vi "Real-Time v01.vi"() -> ()   [LabVIEW 2014]
uses:
  <vilib>/rvi/interface/nirviOpenFPGA/nirviOpenFPGA.xnode
  <vilib>/rvi/interface/nirviReadWriteControl/nirviReadWriteControl.xnode
  <vilib>/Platform/TimedLoop/XDataNode/XDataNode.xnode
  <vilib>/Platform/TimedLoop/XDataNode/nitl_modes.ctl
  <vilib>/Platform/TimedLoop/XDataNode/XDNodeRunTimeDep.lvlib
  <vilib>/Platform/TimedLoop/XDataNode/wakeup.ctl
  <vilib>/Platform/TimedLoop/XDataNode/timing_clust.ctl
  <vilib>/addons/control/pid/NI_PID_pid.lvlib
  <vilib>/rvi/errors/niLvFpgaAdjustHostInterfaceError.vi
  <vilib>/rvi/interface/nirviCloseFPGA/nirviCloseFPGA.xnode
  <vilib>/addons/control/pid/pid.llb/PID (DBL).vi
  NiFpgaLv.dll
  <vilib>/Utility/error.llb/Error Cluster From Error Code.vi
  FPGA Bitfiles/OMEGA_FPGATarget2_FPGASlavev02_Fgk3BcBTm4Y.lvbitx
  FPGA Bitfiles/OMEGA_FPGATarget_FPGAMainv01_bQBX2IVMCsY.lvbitx
  <vilib>/FPGAPlugInAG/cRIO-9067/niLvFpga_Open_cRIO-9067.vi
  <vilib>/FPGAPlugInAG/NI 9146/niLvFpga_Open_NI 9146.vi
  <vilib>/FPGAPlugInAG/cRIO-9067/niLvFpga_Close_cRIO-9067.vi
panel:
  in  "Tc":i32=1
  out "Selectable Tc Tref":dbl format="%#_13g"
  out "Selectable Tc MA":dbl format="%#_13g"
  in  "Red Limit":dbl
  in  "T ref":bool
  in  "Tc Alarm":bool
  in  "Target Temperature":dbl format="%0.2f"
  in  "Yellow Limit":dbl
  out "Fan Factor Speed":dbl
  in  "Fan Speed Recipe":bool
  out "Tstoic 2 R":bool
  out "Tstoic 2 Y":bool
  out "Tstoic 1 R":bool
  out "Tstoic 1 Y":bool
  out "Tspike 2 R":bool
  out "Tspike 2 Y":bool
  out "Omicron 2":bool
  out "Tspike 1 R":bool
  out "Tspike 1 Y":bool
  out "Tref 2 R":bool
  out "Tref 2 Y":bool
  out "Tref 1 R":bool
  out "Tref 1 Y":bool
  out "AutoChanges Spike":string[][](table)
  out "UserChanges Spike":string[][](table)
  out "HC Add":dbl
  out "Exceeded 2":bool
  in  "Write Log":bool
  out "AutoChanges":string[][](table)
  out "UserChanges":string[][](table)
  out "Furnace SP":dbl
  out "Exceeded":bool
  in  "Spike Control":bool
  in  "Target Tspike":dbl
  in  "Target Tstoic":dbl
  in  "Control TC 2":i32=2
  out "T Spike 2":dbl format="%0.2f"
  out "T Max 2":dbl format="%0.2f"
  out "T Stoic 2":dbl
  out "T Ref 2":dbl
  in  "HC 2 Factor":dbl
  in  "HC 2 Add Factor":dbl
  in  "Air-2 Factor":dbl
  in  "Air-2 Add Factor":dbl
  in  "O2-2 Factor":dbl
  in  "Power Limit":dbl
  out "Omicron":bool
  out "T Spike":dbl format="%0.2f"
  in  "TSpike":bool
  in  "TSpike Target":dbl format="%0.2f"
  in  "TStoic":bool
  in  "TStoic Target":dbl format="%0.2f"
  out "Alarm Output 2":bool[](array[boolean])
  in  "Flow":bool
  in  "Lambda":bool
  in  "Pressure":bool
  in  "Heat Exch Fan V":fxp<+/-,20,5>
  in  "Air Bal Transient":dbl
  in  "Air Bal Adaptive Control":bool
  in  "HC Bal Adaptive Control":bool
  in  "HC Bal Transient":dbl
  in  "TRef":bool
  in  "TRef Target":dbl format="%0.2f"
  out "T Max":dbl format="%0.2f"
  out "T Stoic":dbl
  out "T Ref":dbl
  in  "Extract Fan V":fxp<+/-,20,5>
  in  "ETAS Control":bool
  in  "Dual Evac":bool
  out "Valve 4":dbl
  out "Valve 3":dbl
  out "OSCArray":dbl[](array[numeric])
  out "Flow rate g/s":dbl
  out "OSC Stop":bool
  in  "O2 Factor":dbl
  in  "HC Switch":bool
  out "Time Step":i32
  out "O2":bool
  out "HC-2":bool
  out "N2-2":bool
  in  "Valve 3 SP":dbl=1.0
  in  "Valve 4 SP":dbl=1.0
  in  "N2 Age":dbl
  in  "N2 2":dbl format="%#_13g"
  in  "N2":dbl format="%#_13g"
  in  "O2":dbl format="%#_13g"
  out "Flow Avg":dbl
  in  "Flow Up":sgl=50.0
  in  "Flow Low":sgl
  out "Avg Control":dbl format="%0.2f"
  out "Uego Avg Fur":dbl
  in  "PID gains O2":T1={"proportional gain (Kc)"=1.0, "integral time (Ti, min)"=0.01, "derivative time (Td, min)"=0.0} {"derivative time (Td, min)" format="%.3f"; "integral time (Ti, min)" format="%.3f"; "proportional gain (Kc)" format="%.3f"}
  in  "PID gains CO":T1={"proportional gain (Kc)"=1.0, "integral time (Ti, min)"=0.01, "derivative time (Td, min)"=0.0} {"derivative time (Td, min)" format="%.3f"; "integral time (Ti, min)" format="%.3f"; "proportional gain (Kc)" format="%.3f"}
  in  "Manual Valve":bool
  in  "Control TC":i32=1
  in  "Flow Offset":dbl
  in  "HC Fact HCLO":dbl
  in  "HC Base HCLO":dbl
  in  "O2 Base HCLO":dbl
  in  "O2 Fact HCLO":dbl
  in  "Ageing Metric\nControl":enum32{"Catalyst 1 ", "Catalyst 2 ", "All"}(radio)
  out "UEGO Array":dbl[](array[numeric])
  in  "UEGO 3":i64=200
  out "UEGO Sensor Results":T2
  in  "SensorControl":T3={"UEGO1Enable"=TRUE, "UEGO2Enable"=TRUE, "EGO1Enable"=FALSE, "EGO2Enable"=FALSE, "EGO3Enable"=FALSE, "EGO4Enable"=FALSE, "UEGO1Range"=FALSE, "UEGO2Range"=FALSE, "FilterCutoff (Hz)"=10.0}
  in  "UEGO Back Pressure (bar)":T4={"UEGO1BackPressure (bar)"=1.013, "UEGO2BackPressure (bar)"=1.013}
  in  "UEGOModuleEnable":bool=TRUE
  out "UEGO Heater (V)":T5
  out "UEGO Diagnostics":T6={"ModulePresent"=FALSE, "UEGO1SensorFault"=63, "UEGO2SensorFault"=63, "UEGO1HeaterFault"=192, "UEGO2HeaterFault"=192, "UEGOFuseStatus"=0, "Battery (V)"=0.0, "LSUType"=0} {"LSUType" items=["LSU 4.9", "LSU 4.2"]; "UEGOFuseStatus" items=["FUSE OK", "FUSE BLOWN"]; "UEGO2SensorFault" items=["NO FAULT"=63, "SHORT TO GND OR BATT"=0]; "UEGO2HeaterFault" items=["SHORT TO GROUND"=0, "OPEN CIRCUIT"=64, "SHORT TO BATTERY"=128, "NO FAULT"=192]; "UEGO1SensorFault" items=["NO FAULT"=63, "SHORT TO GND OR BATT"=0]; "UEGO1HeaterFault" items=["SHORT TO GROUND"=0, "OPEN CIRCUIT"=64, "SHORT TO BATTERY"=128, "NO FAULT"=192]}
  out "UEGO Temperature (C)":T7
  in  "Start Test":bool
  out "Ready":bool
  in  "Reset AM 2":bool
  out "% Complete 2":dbl
  out "Complete 2":dbl(slide) scale=0.0..100.0
  out "Remaining Time 2":dbl format="%<%H:%M:%S>t"
  out "Ageing Time 2":dbl format="%<%H:%M:%S>t"
  in  "P-Transducer 1":enum32{"Druck ", "FUJI ", "Impress"}(radio)=enum."FUJI "
  out "Valve 2":dbl
  out "Valve 1":dbl
  in  "Valve 2 SP":dbl=1.0
  in  "Valve 1 SP":dbl=1.0
  out "Lambda Avg":dbl
  in  "Press Up":sgl=5.0
  in  "Press Low":sgl
  out "Loop No.":i32
  out "Air-2":bool
  out "HC-B":bool
  out "Air-B":bool
  out "N2":bool
  out "NO":bool
  out "Air":bool
  out "HC":bool
  out "CO":bool
  in  "NO/CO-2 Factor":dbl
  in  "CO Factor":dbl
  in  "Set-point Fan":dbl
  in  "Fan PID":bool
  in  "Furnace SP":dbl=2.0
  in  "Furnace Manual":bool
  in  "Reset AM 1":bool
  in  "Lambda Control":bool
  in  "Lambda SP 3":dbl
  in  "Output Low 3":dbl
  in  "Output High 3":dbl
  in  "PID Mop-up Catalyst":T1={"proportional gain (Kc)"=0.8, "integral time (Ti, min)"=0.8, "derivative time (Td, min)"=0.0}
  in  "NO PID Light-Off":T1={"proportional gain (Kc)"=1.0, "integral time (Ti, min)"=0.0, "derivative time (Td, min)"=0.0}
  in  "NO PID Sweep Test":T1={"proportional gain (Kc)"=1.0, "integral time (Ti, min)"=0.0, "derivative time (Td, min)"=0.0}
  in  "NO":dbl format="%#_13g"
  in  "CO":dbl format="%#_13g"
  out "% Complete":dbl
  out "Complete":dbl(slide) scale=0.0..100.0
  out "Remaining Time":dbl format="%<%H:%M:%S>t"
  out "Ageing Time":dbl format="%<%H:%M:%S>t"
  out "Tank Pressure":dbl
  out "Inlet Temp":sgl
  out "Cycle Length":i32
  in  "HC Cyc 2":dbl format="%#_13g"
  in  "HC Bal":dbl format="%#_13g"
  in  "Air Cyc 1":dbl format="%#_13g"
  in  "Air Cyc 2":dbl format="%#_13g"
  in  "Air Bal":dbl format="%#_13g"
  in  "HC Cyc 1":dbl format="%#_13g"
  in  "Furnace 1":sgl=10.0
  in  "Air Cyc Add Factor":dbl
  in  "Air Cyc Factor":dbl
  in  "HC Cyc Add Factor":dbl
  in  "HC Bal Factor":dbl
  in  "Air Bal Factor":dbl
  in  "HC Cyc Factor":dbl
  in  "Stoic Control":bool
  in  "Lambda \nTarget":sgl=5.0
  out "Flow 1":dbl
  out "Test Start":i32
  out "Control Variables":dbl[](array[numeric])
  out "Iteration \nDuration 3":i64
  in  "NO Base NOLO":dbl
  in  "NO Factor NOLO":dbl
  in  "CO Base NOLO":dbl
  in  "CO Factor NOLO":dbl
  in  "CO Base COLO":dbl
  in  "O2 Base COLO":dbl
  in  "CO Fact COLO":dbl
  in  "O2 Fact COLO":dbl
  in  "NO Furnace Inlet":dbl=5.0
  in  "CO Furnace Inlet":dbl=5.0
  in  "OSC Furnace Inlet":dbl=5.0
  in  "HC Furnace Inlet":dbl=0.2
  in  "Sw time":dbl
  in  "Age Furnace Inlet":dbl=5.0
  in  "Age Lam Lim":dbl=5.0
  in  "OSC Lam lim":dbl=5.0
  in  "CO Lam Lim":dbl=5.0
  in  "NO Lam Lim":dbl=5.0
  in  "Fan Speed V":dbl
  in  "HC Lam lim":dbl=0.2
  in  "STOP":bool
  in  "TankLo":dbl=1.5
  in  "TankHi":dbl=2.0
  out "DI no1":u32
  in  "PID Inverter":T1={"proportional gain (Kc)"=0.8, "integral time (Ti, min)"=0.8, "derivative time (Td, min)"=0.0}
  out "Iteration Duration 2":i64
  # "Spike Change Log"
  # "Furnace Change Log"
  # "OMEGA Real-Time"
  # "Loop Readings"
  # "MFC Alarms"
  # "System Readings"
  # "Pressure Release Limits"
  # "Ageing Metric 1"
  # "kPa"
  # "kPa"
  # "Fan Control"
  # "Cooling Fan Control"
  # "Warm-up"
  # "Rapidox Limit"
  # "Furnace Limit"
  # "Ageing Metric 2"
  # "g/s"
  # "Furnace Control"
  # "Ageing"
  # "Cycle Alarms"
  # "System Settings"
  # "Cycle Factors"
  # "System Balance Factors"
  # "Mopup Lambda PID Control"
  # "When Adaptive Control \nSelected Air Bal Factor \nwill adjust lambda up or\n down it will not affect \nTransients"
  # "When Adaptive Control \nSelected HC Bal Factor \nwill adjust lambda up or\n down it will not affect \nTransients"
  # "On ETAS\nOff Furnace"
  # "Furnace PID Control"
  # "Other PID Control"
  # "Select for Tref calc,\notherwise MA is used"
  # "Light Off's"
  # "UEGO Module 3"
  # "NO Light - off"
  # "HC Light - off"
  # "CO Light - off"
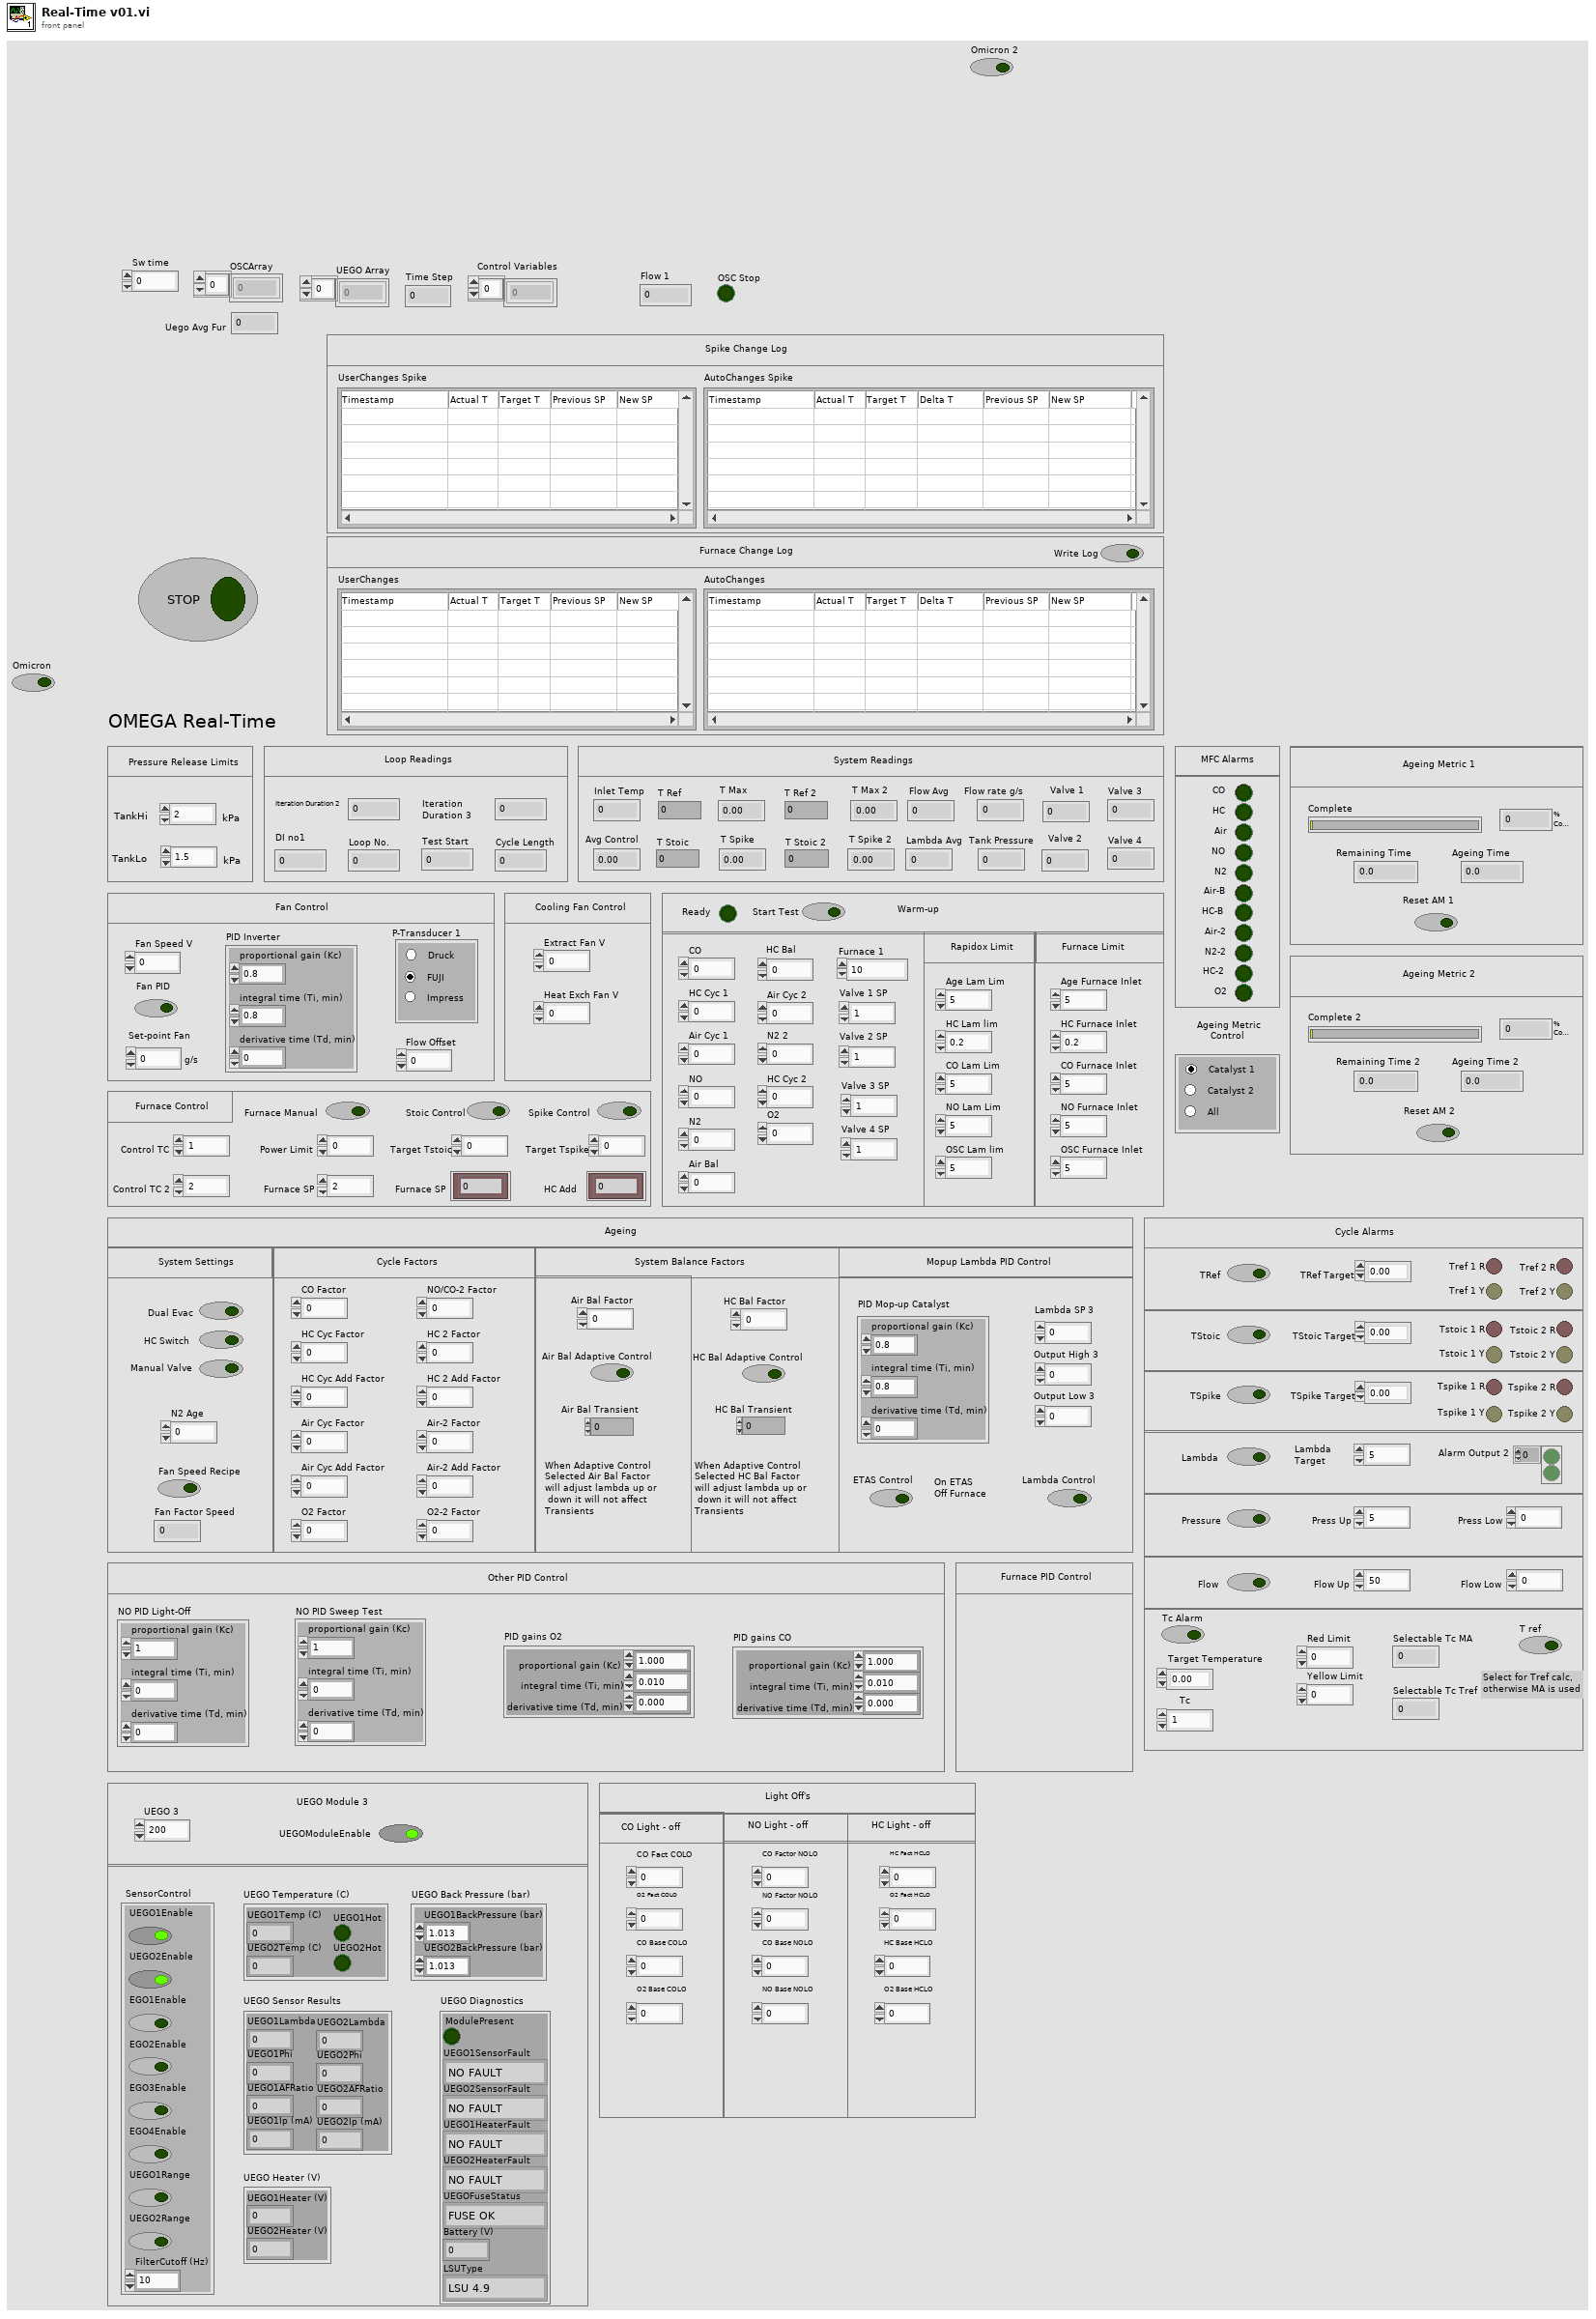
[diagram p1: front panel]
types:
  T1 = cluster{"proportional gain (Kc)":dbl, "integral time (Ti, min)":dbl, "derivative time (Td, min)":dbl}
  T2 = cluster{"UEGO1Lambda":sgl, "UEGO1Phi":sgl, "UEGO1AFRatio":sgl, "UEGO1Ip (mA)":sgl, "UEGO2Lambda":sgl, "UEGO2Phi":sgl, "UEGO2AFRatio":sgl, "UEGO2Ip (mA)":sgl}
  T3 = cluster{"UEGO1Enable":bool, "UEGO2Enable":bool, "EGO1Enable":bool, "EGO2Enable":bool, "EGO3Enable":bool, "EGO4Enable":bool, "UEGO1Range":bool, "UEGO2Range":bool, "FilterCutoff (Hz)":dbl}
  T4 = cluster{"UEGO1BackPressure (bar)":sgl, "UEGO2BackPressure (bar)":sgl}
  T5 = cluster{"UEGO1Heater (V)":sgl, "UEGO2Heater (V)":sgl}
  T6 = cluster{"ModulePresent":bool, "UEGO1SensorFault":u8, "UEGO2SensorFault":u8, "UEGO1HeaterFault":u8, "UEGO2HeaterFault":u8, "UEGOFuseStatus":u8, "Battery (V)":sgl, "LSUType":u8}
  T7 = cluster{"UEGO1Temp (C)":sgl, "UEGO2Temp (C)":sgl, "UEGO1Hot":bool, "UEGO2Hot":bool}
  T8 = cluster{string[][], string[][], dbl[], "Furnace Set-point":dbl, "It Out":i32}
  T9 = typedef "XDNodeRunTimeDep.lvlib/timing_clust.ctl" = cluster{"Expected End [f-1]":u64, "Actual End [f-1]":u64, "Finished Late? [f-1]":bool, "Expected End [i-1]":u64, "Actual End [i-1]":u64, "Finished Late? [i-1]":bool, "Expected Start [i]":u64, "Actual Start [i]":u64, "Expected Start [f]":u64, "Actual Start [f]":u64, "Source Name":string, "Structure Name":string, "Period":i64, "Deadline":i64, "Offset":i64, "Start":i64, "Priority":i32, "Timeout":i32, "Mode":T10, "Wakeup Reason":T11, "Error":errorcluster, "Source Type":string, "Secondary Source Type":string, "Global End Time":u64, "Global Start Time":u64, "Frame Duration":u64, "Iteration Duration":u64, "Assigned CPU":i32, "I/O Scan Engine Mode":u32}
  T10 = typedef "XDNodeRunTimeDep.lvlib/nitl_modes.ctl" = enum32{"No Change", "Process missed periods, maintain original phase", "Discard missed periods, maintain original phase", "Process missed periods, ignore original phase", "Discard missed periods, ignore original phase"}
  T11 = typedef "XDNodeRunTimeDep.lvlib/wakeup.ctl" = enum32{"Normal", "Aborted", "Asynchronous wakeup", "Timing source error", "Timed loop error", "Timeout"}
  T12 = cluster{"UserChanges":string[][], "AutoChanges":string[][], "Stoich Array":dbl[], "Furnace SP":dbl, "It Out":i32}
  T13 = cluster{"UserChanges":string[][], "AutoChanges":string[][], "Spike Array":dbl[], "User HC Add":dbl, "countdown":i32}
  T14 = cluster{"Stoich A/F Ratio":sgl, "IpArray (mA)":sgl[], "LambdaArray":sgl[]}
  T15 = cluster{"UEGO1Diag":u8, "UEGO2Diag":u8, "UEGO1Sensor":u16, "UEGO2Sensor":u16, "UEGO1Heater":u16, "UEGO2Heater":u16, "UEGO1AmpOffset":u16, "UEGO2AmpOffset":u16, "UEGO1RIOffset":u16, "UEGO2RIOffset":u16, "UEGO1HeaterGain":u16, "UEGO2HeaterGain":u16, "Fuse":u16, "EGO1Sensor":u16, "EGO2Sensor":u16, "EGO3Sensor":u16, "EGO4Sensor":u16, "Battery":u16, "ModulePresent":bool, "UEGO1ID":u8, "UEGO2ID":u8, "LSUType":u8}
  T16 = cluster{"ModuleEnable":bool, "WatchdogIn":bool, "UEGO1Hot":bool, "UEGO2Hot":bool, "Cal1Request":bool, "Cal2Request":bool, "UEGOHeaterPeriod":u16, "UEGO1HeaterPulseWidth":u16, "UEGO2HeaterPulseWidth":u16, "UEGO1Range":bool, "UEGO2Range":bool, "LSUType (F=4.9,T=4.2)":bool}
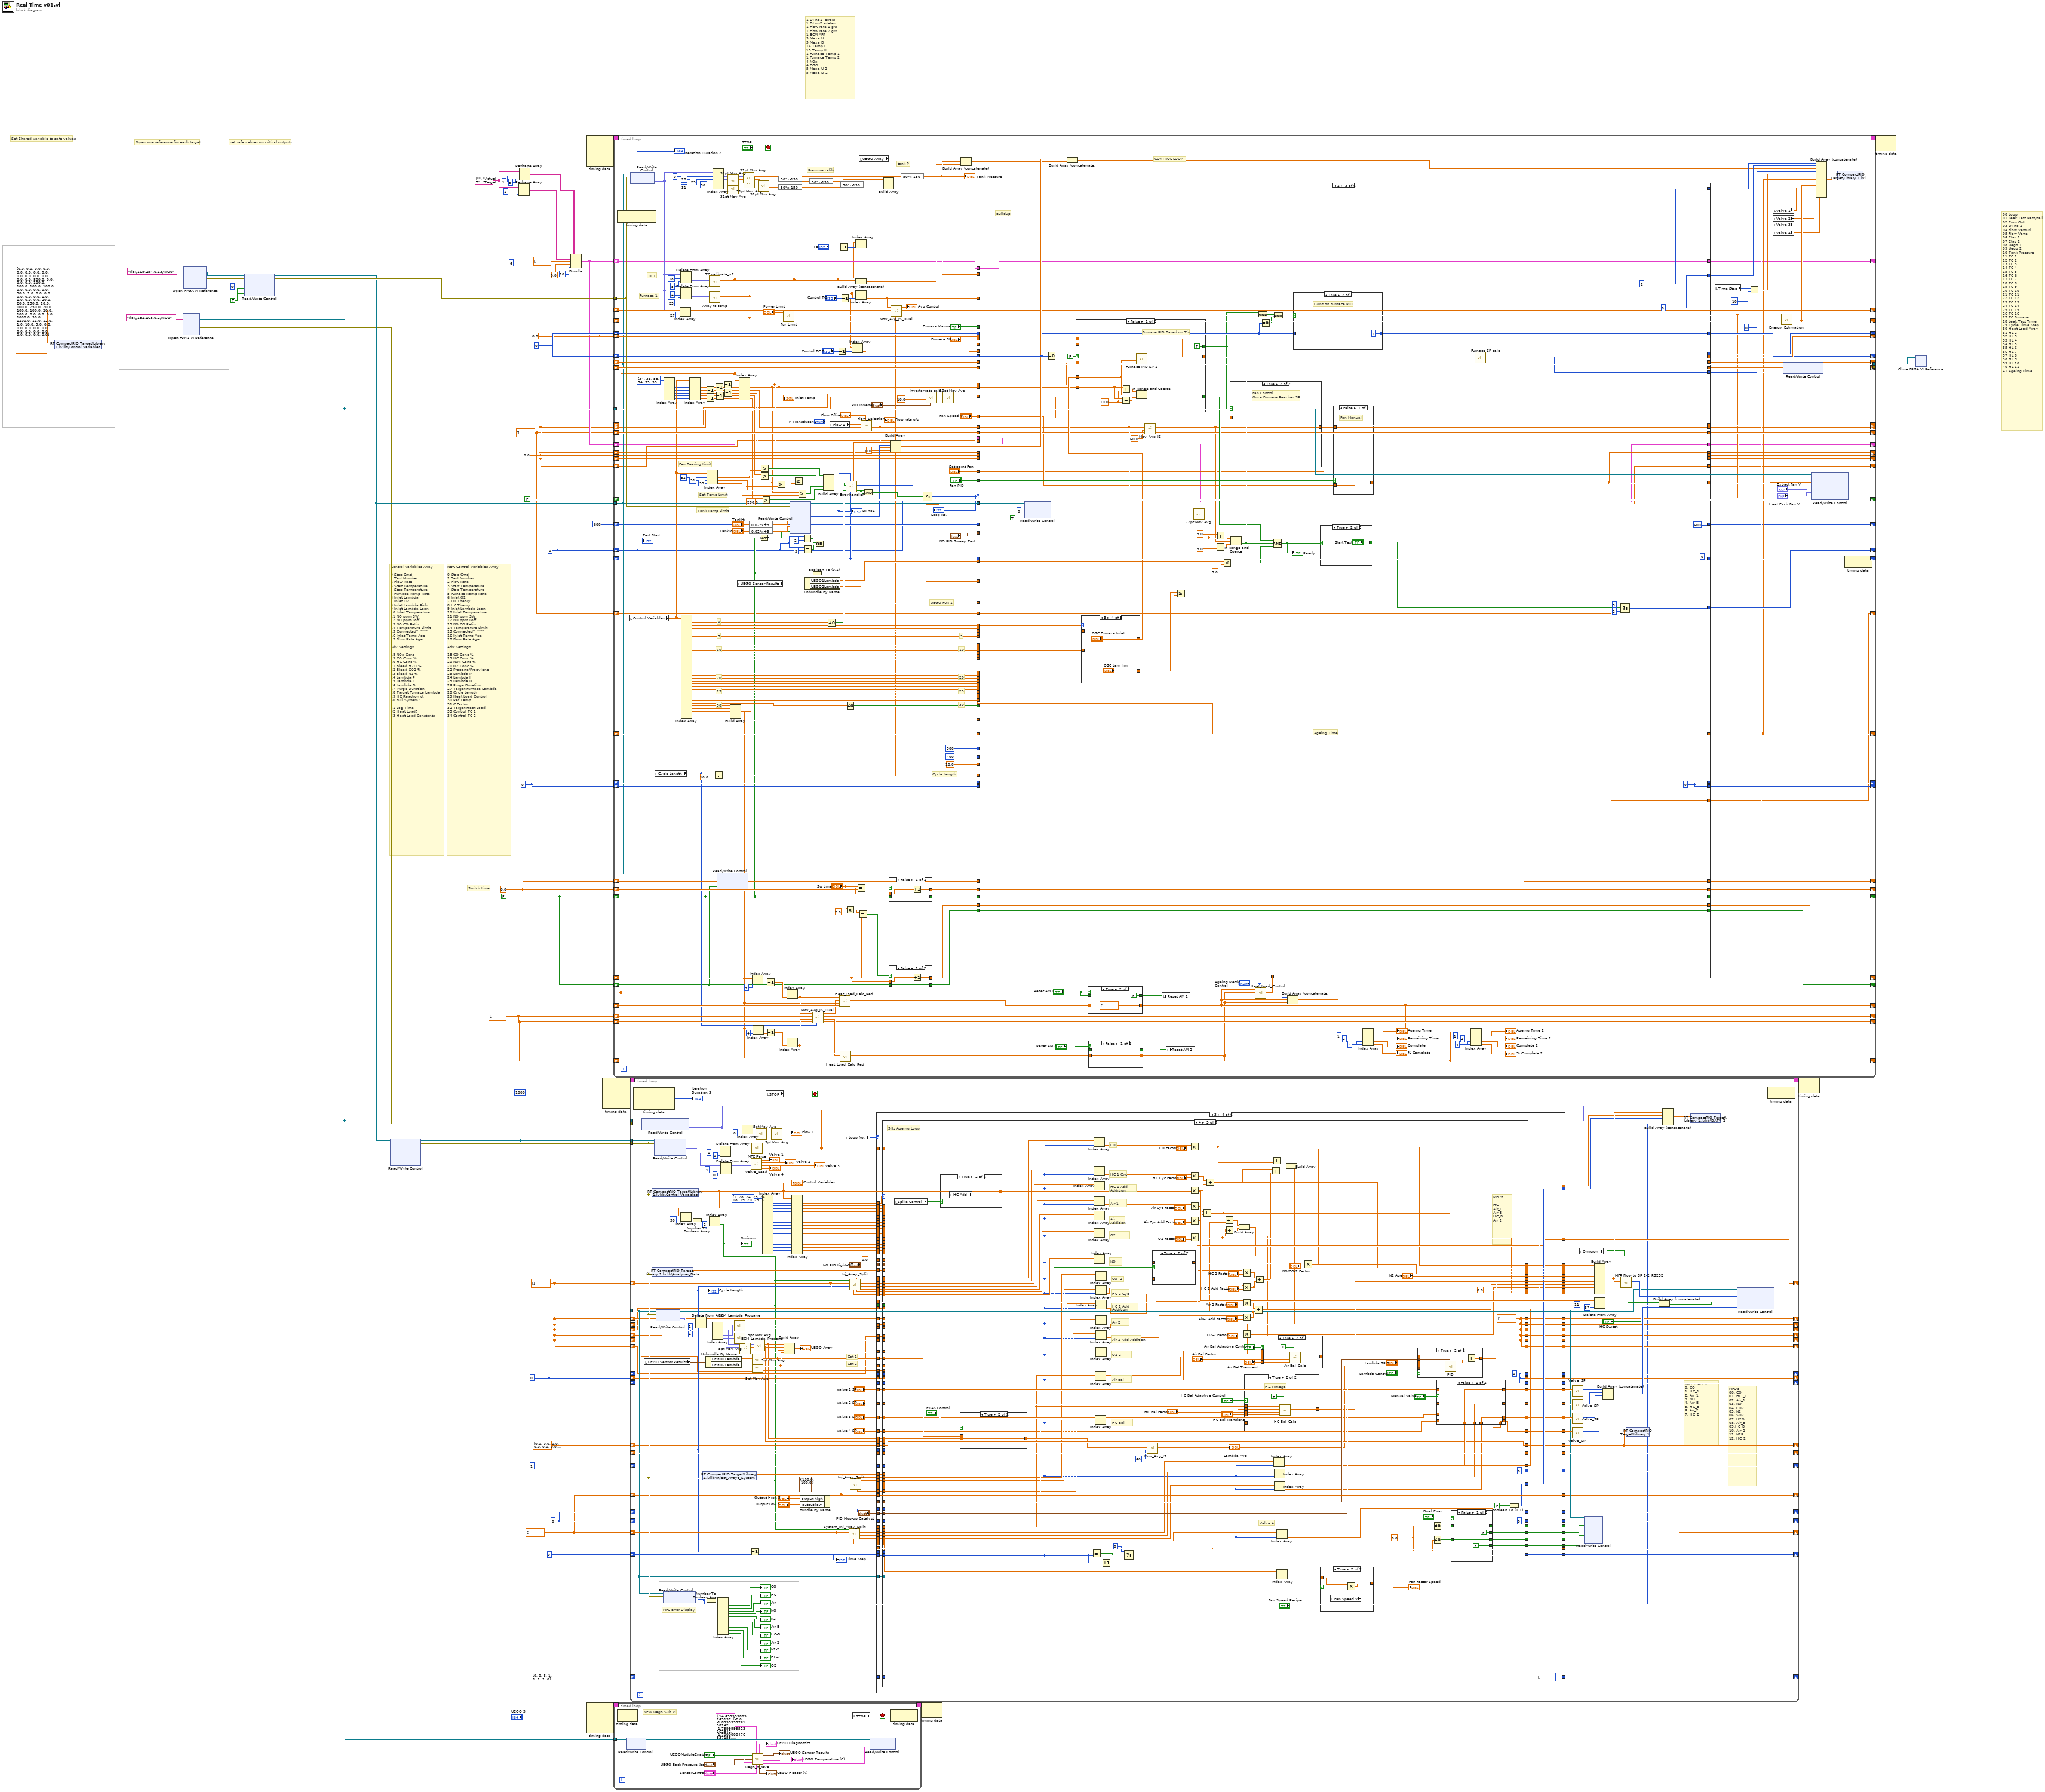
[diagram p0: block diagram]
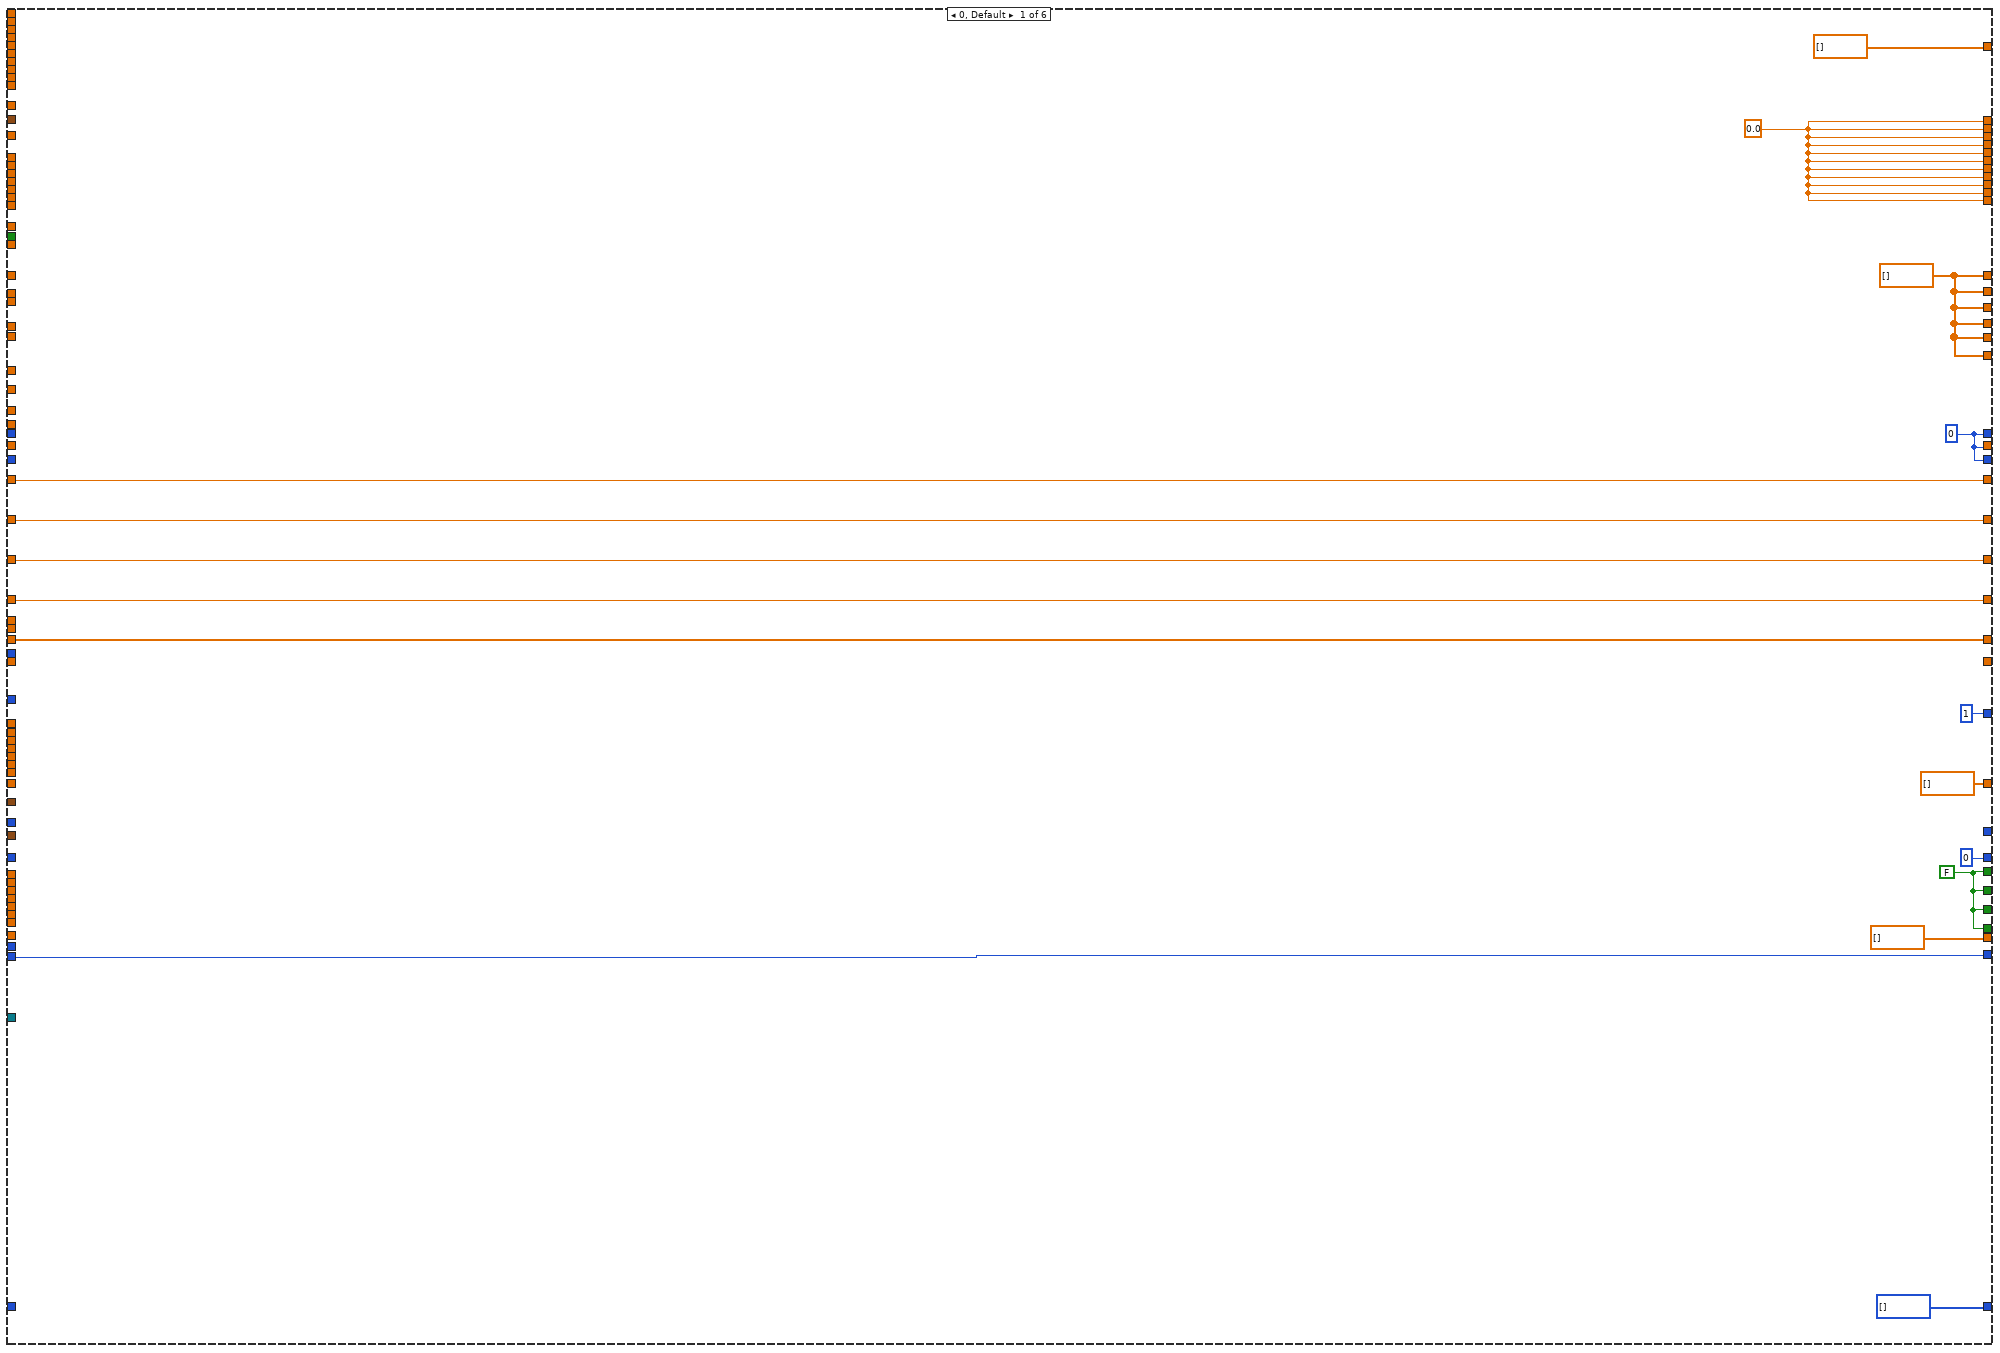
[diagram p2: hidden frame]
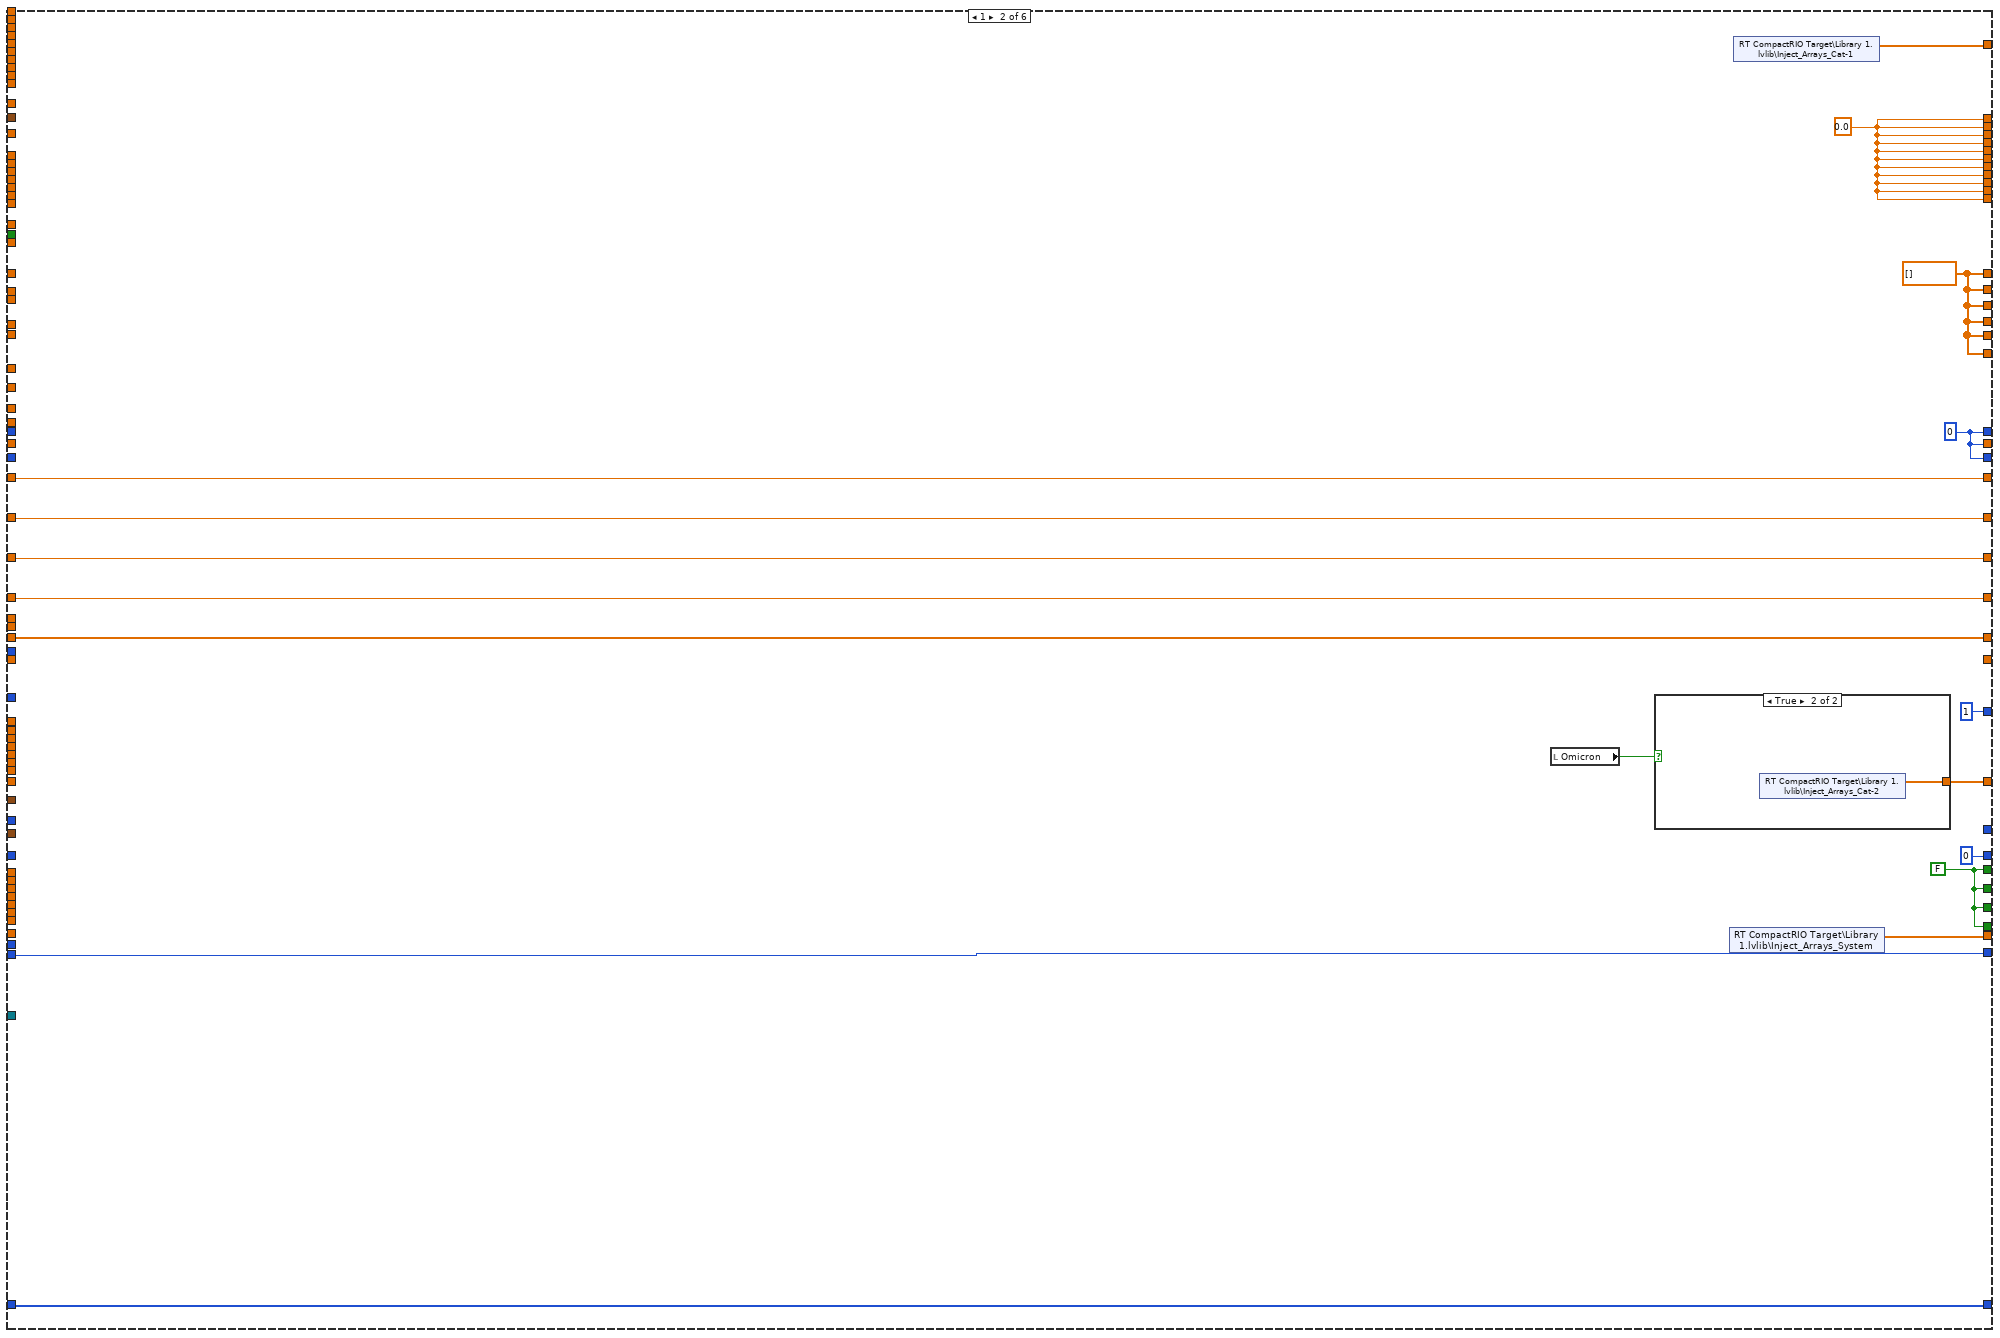
[diagram p3: hidden frame]
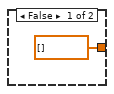
[diagram p4: hidden frame]
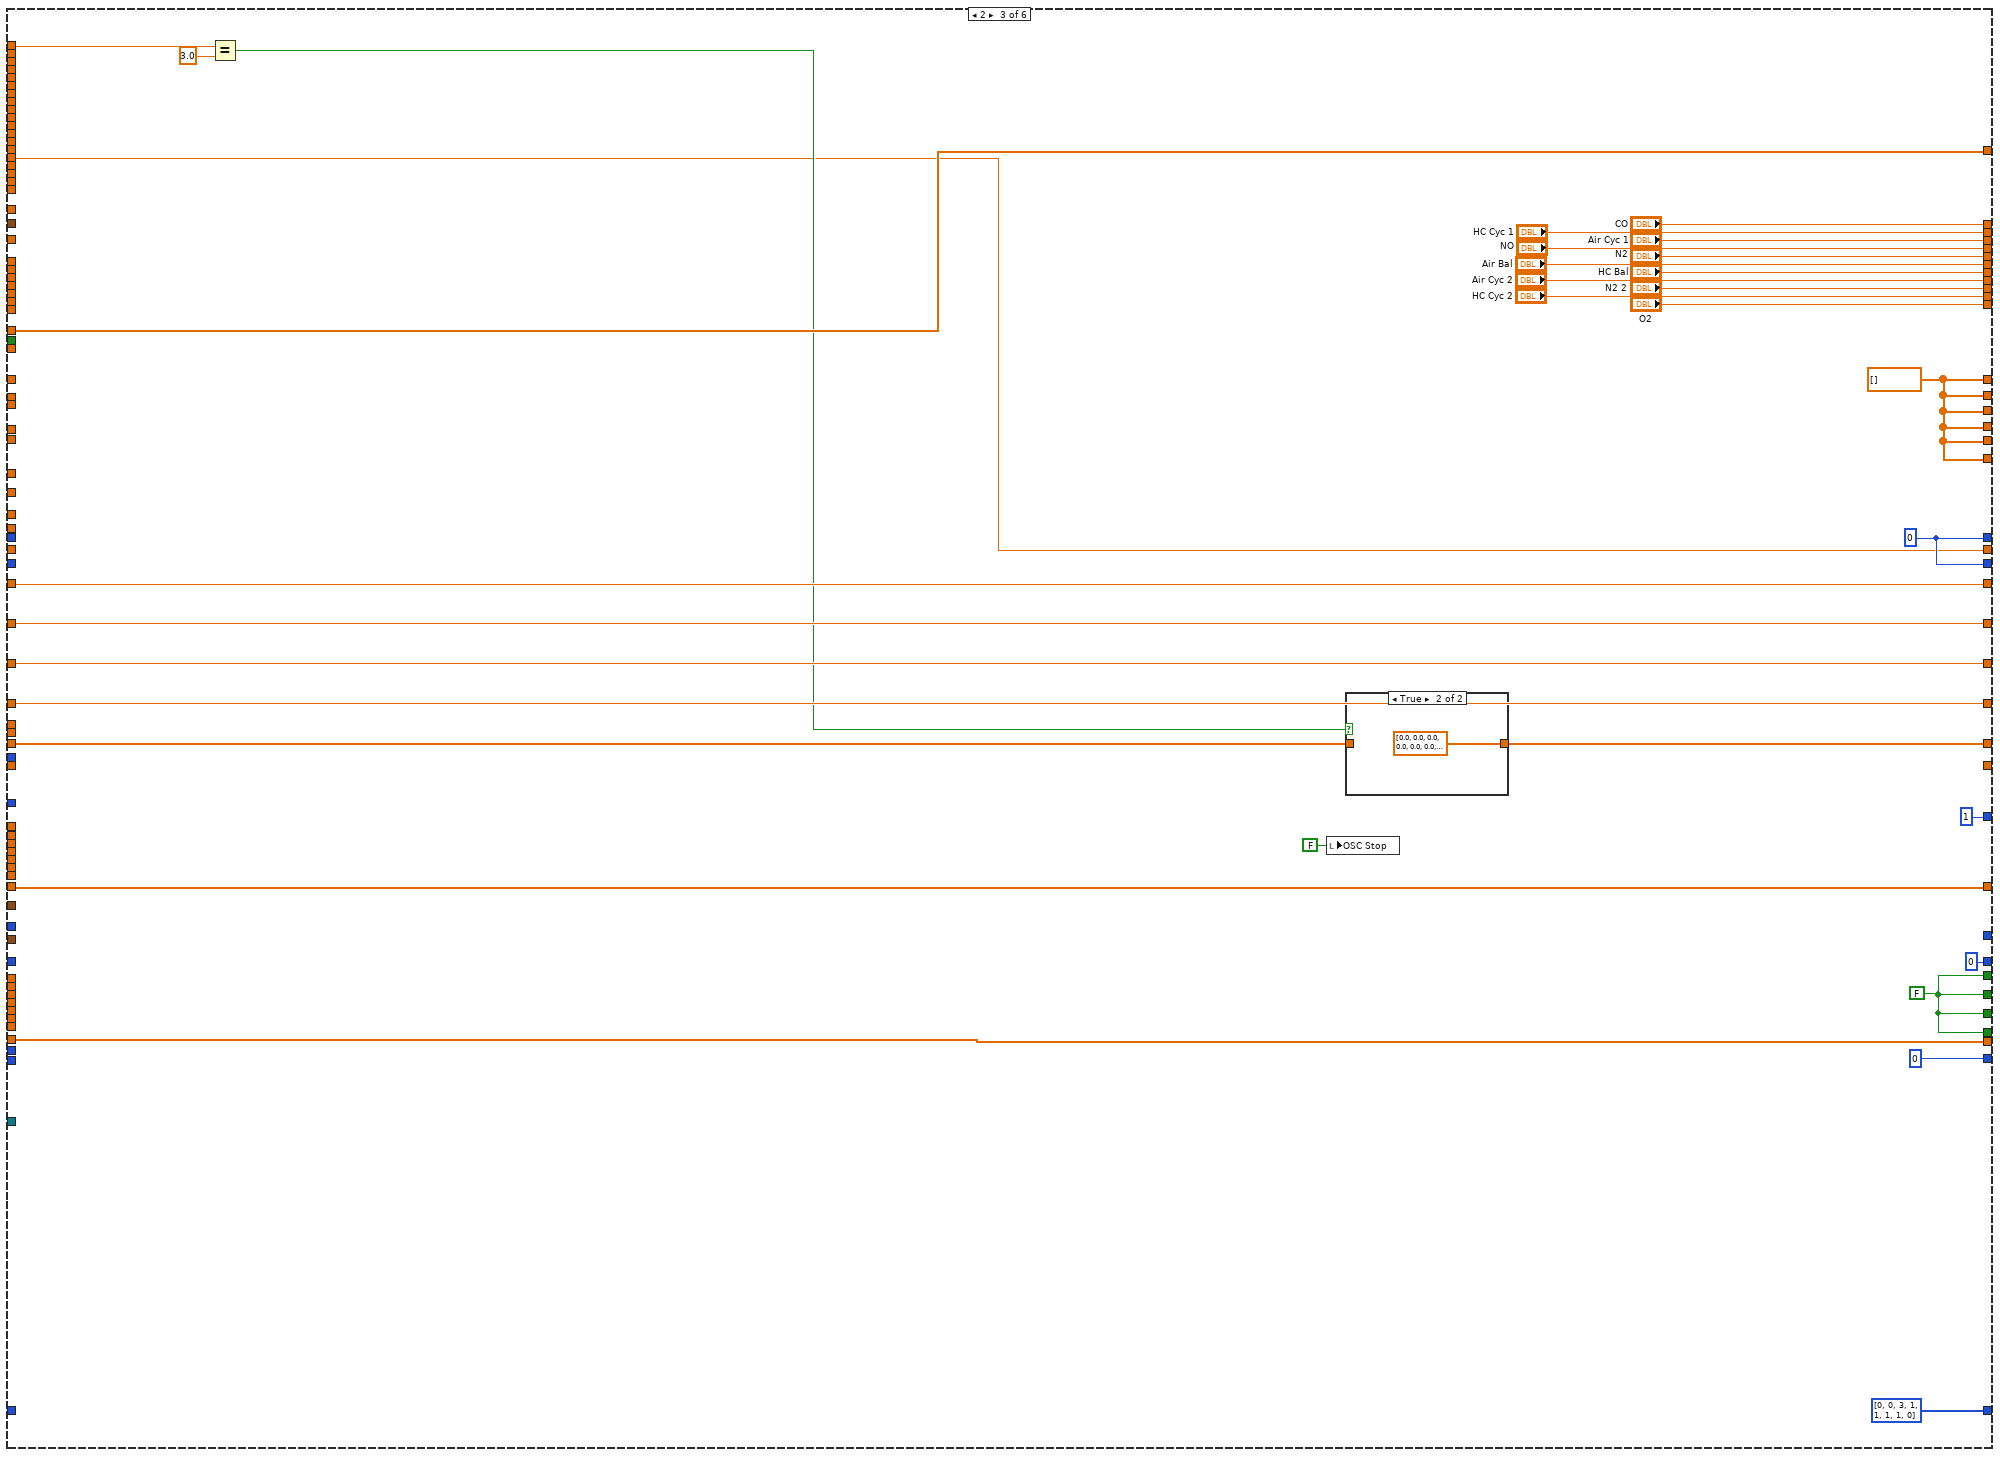
[diagram p5: hidden frame]
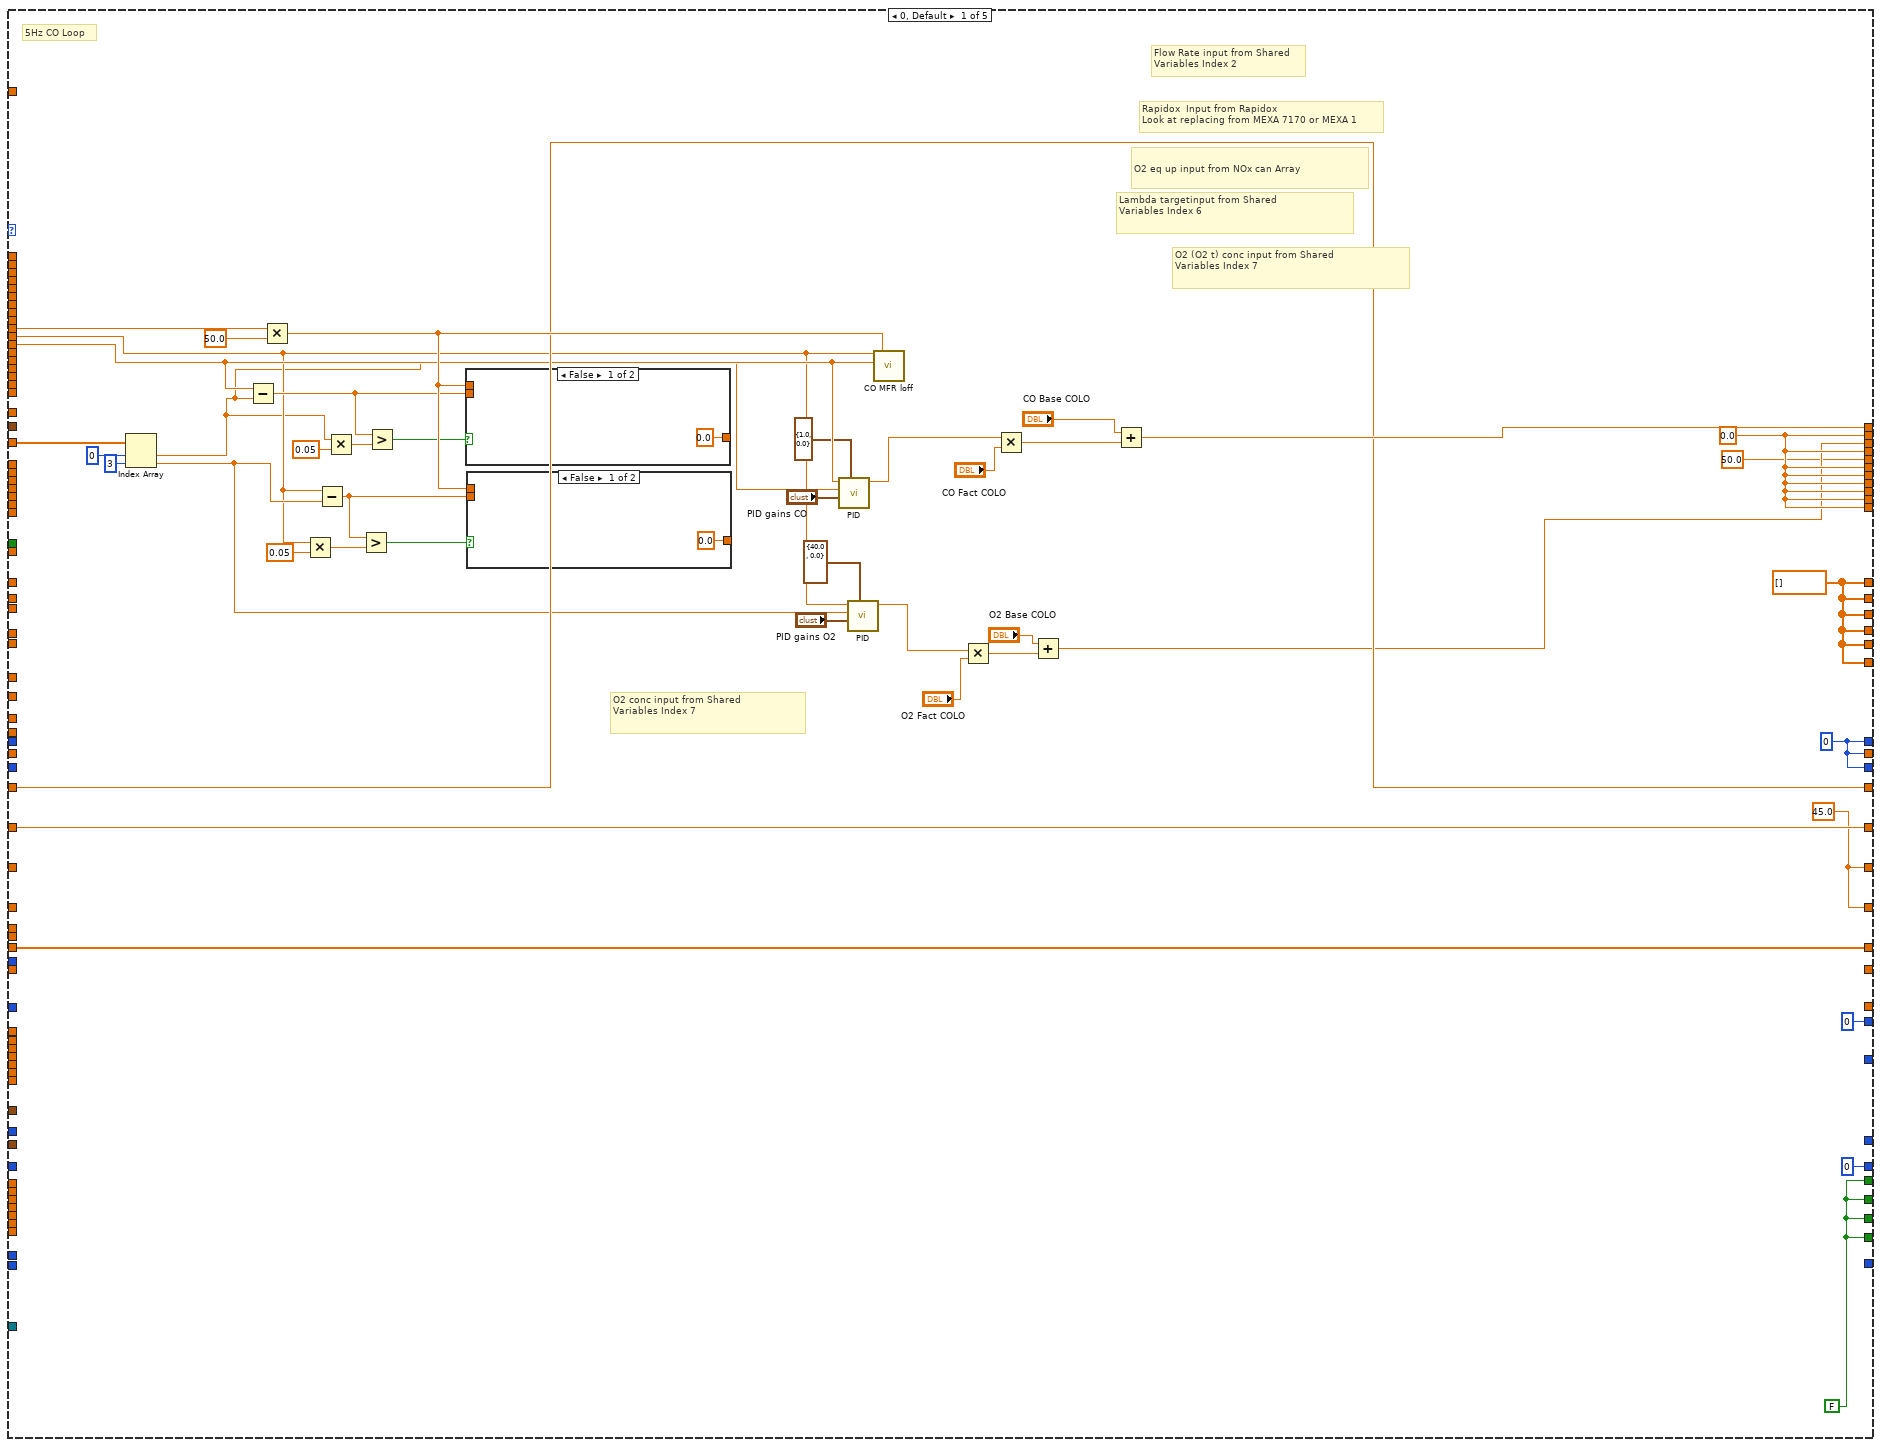
[diagram p7: hidden frame]
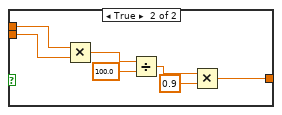
[diagram p8: hidden frame]
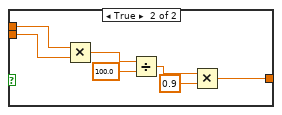
[diagram p9: hidden frame]
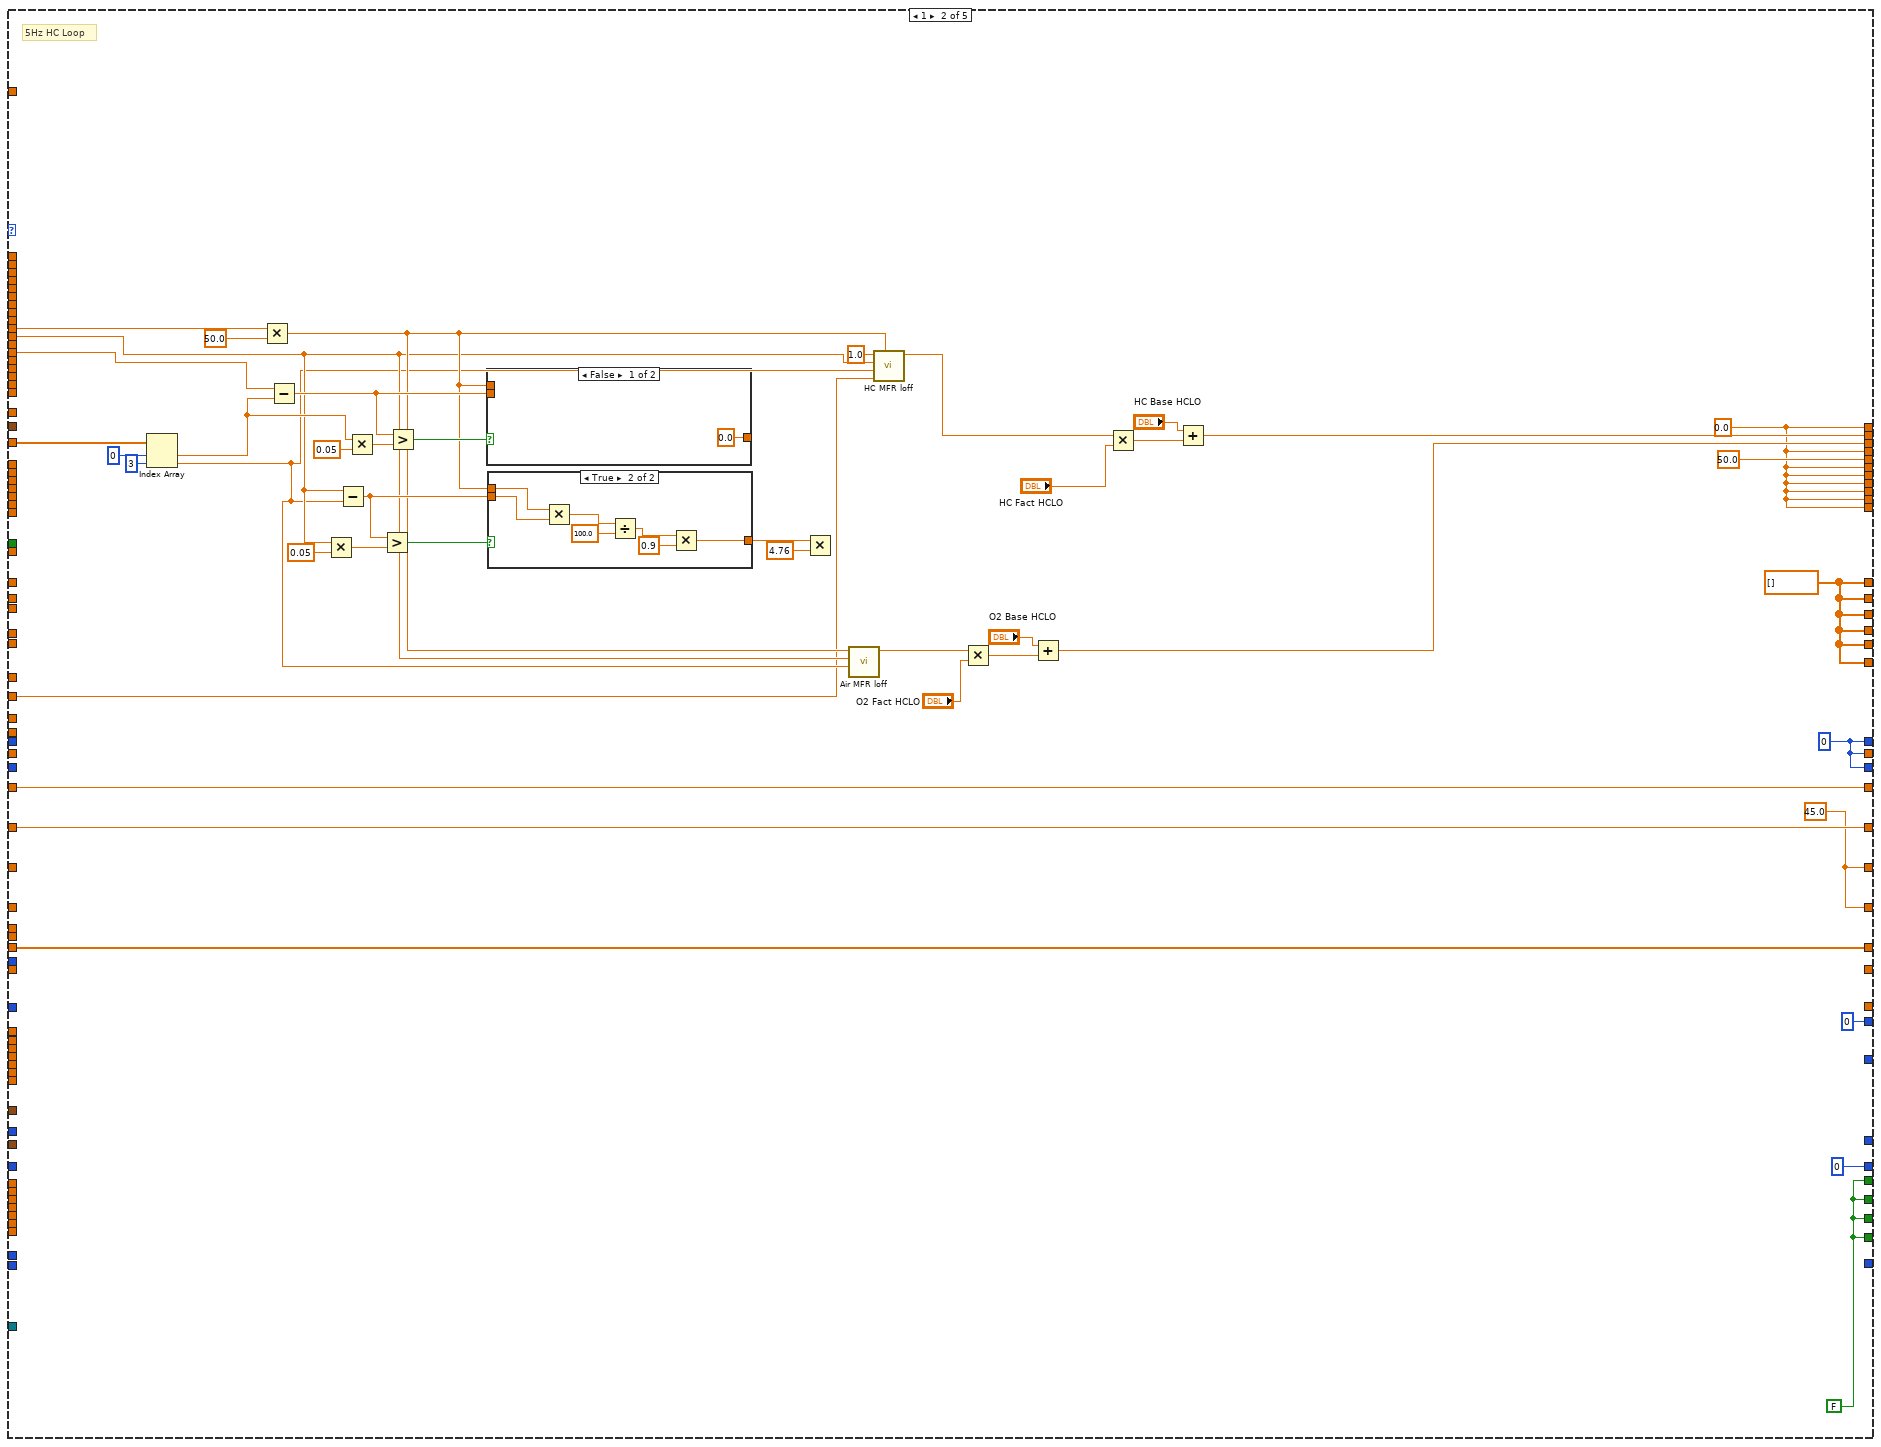
[diagram p10: hidden frame]
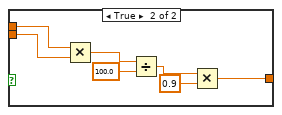
[diagram p11: hidden frame]
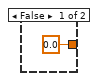
[diagram p12: hidden frame]
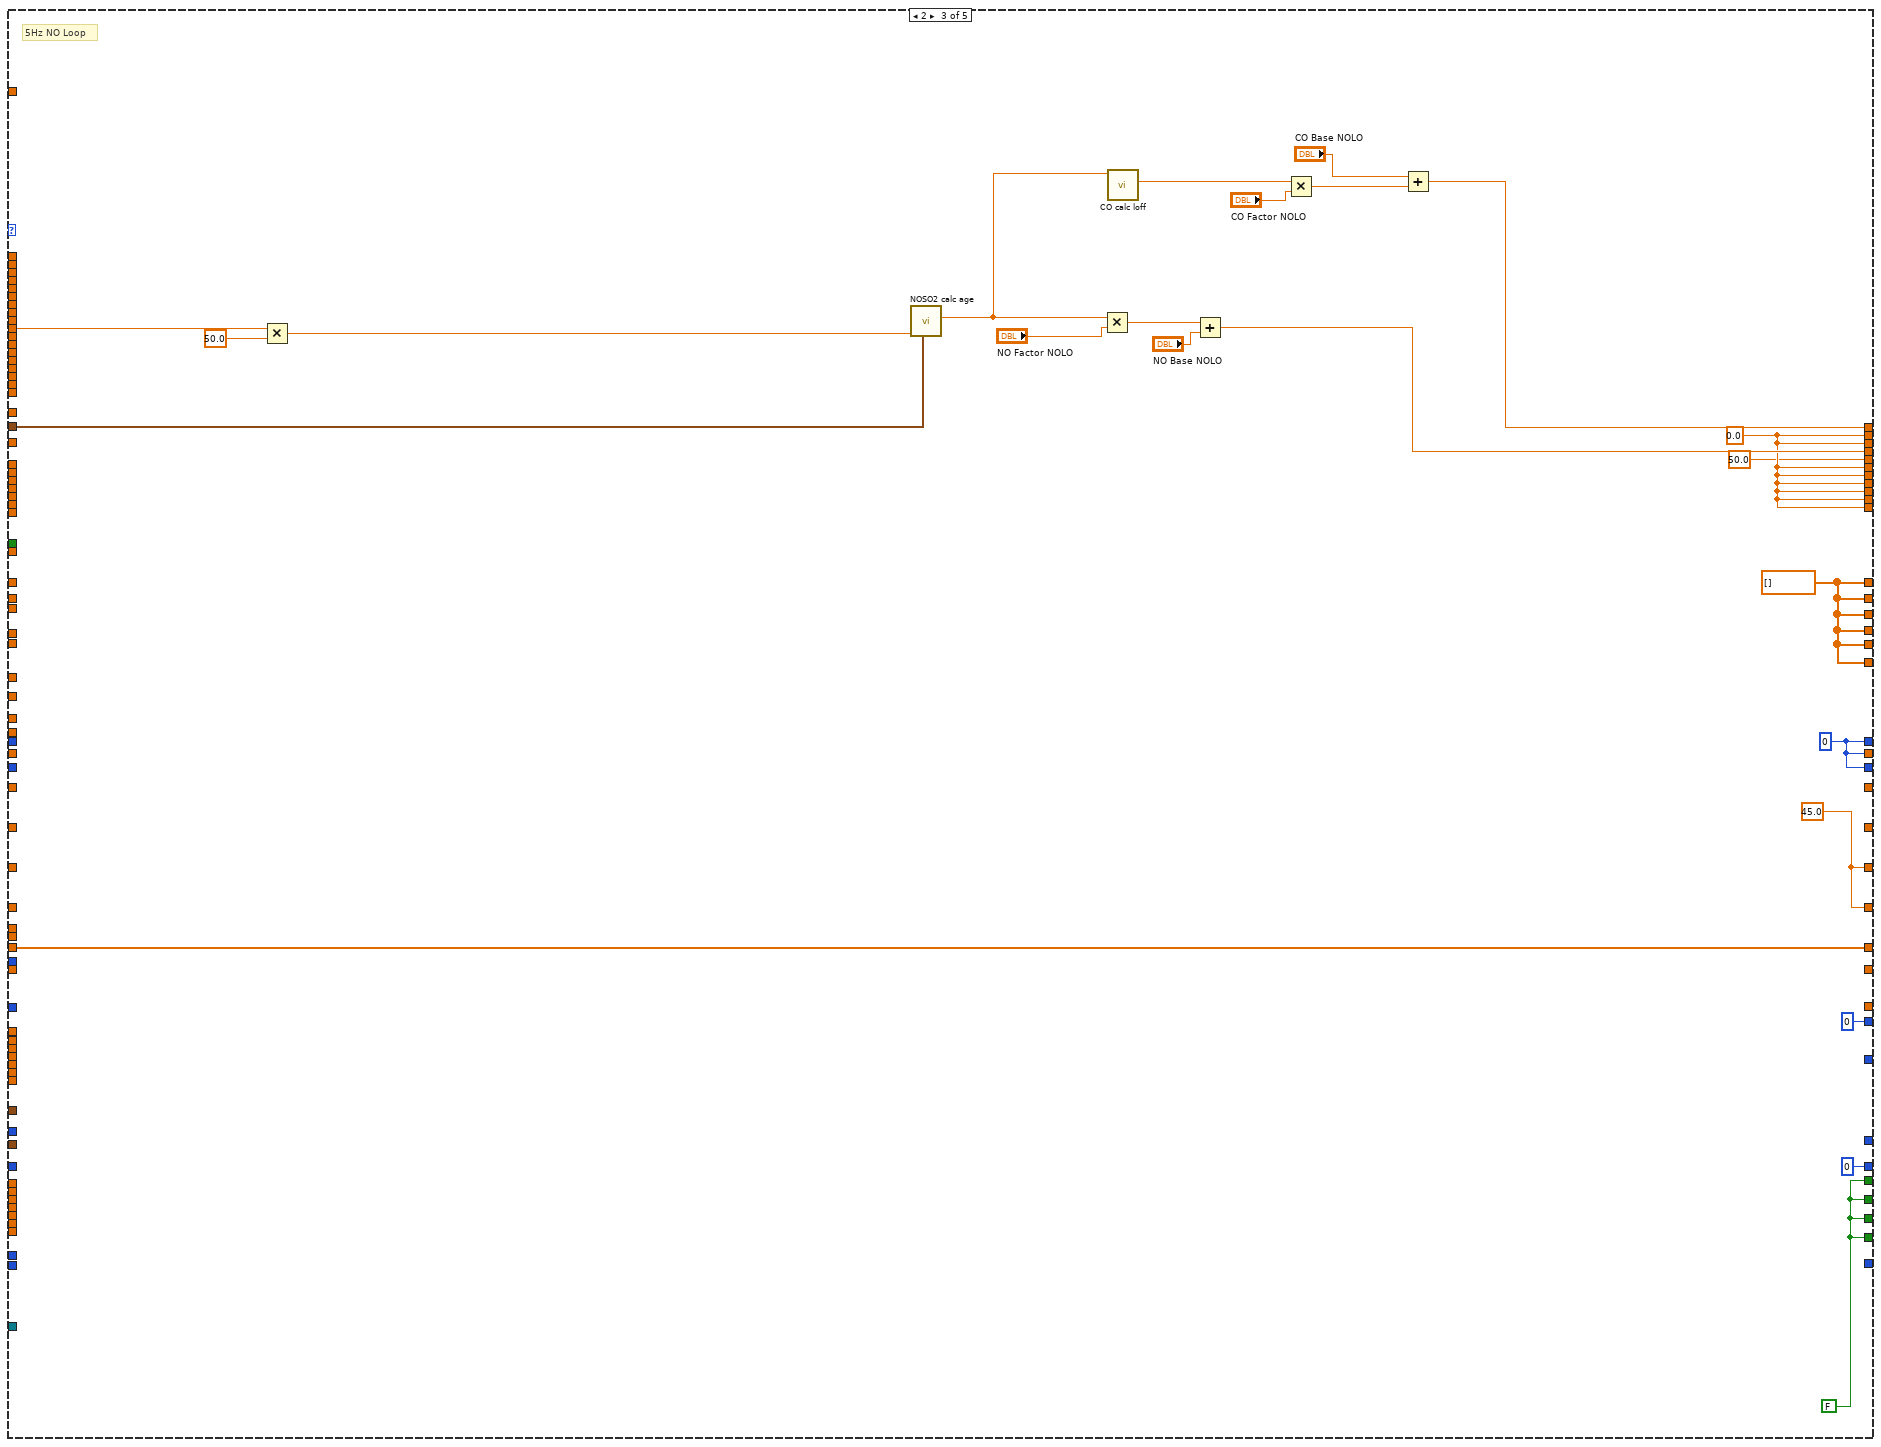
[diagram p13: hidden frame]
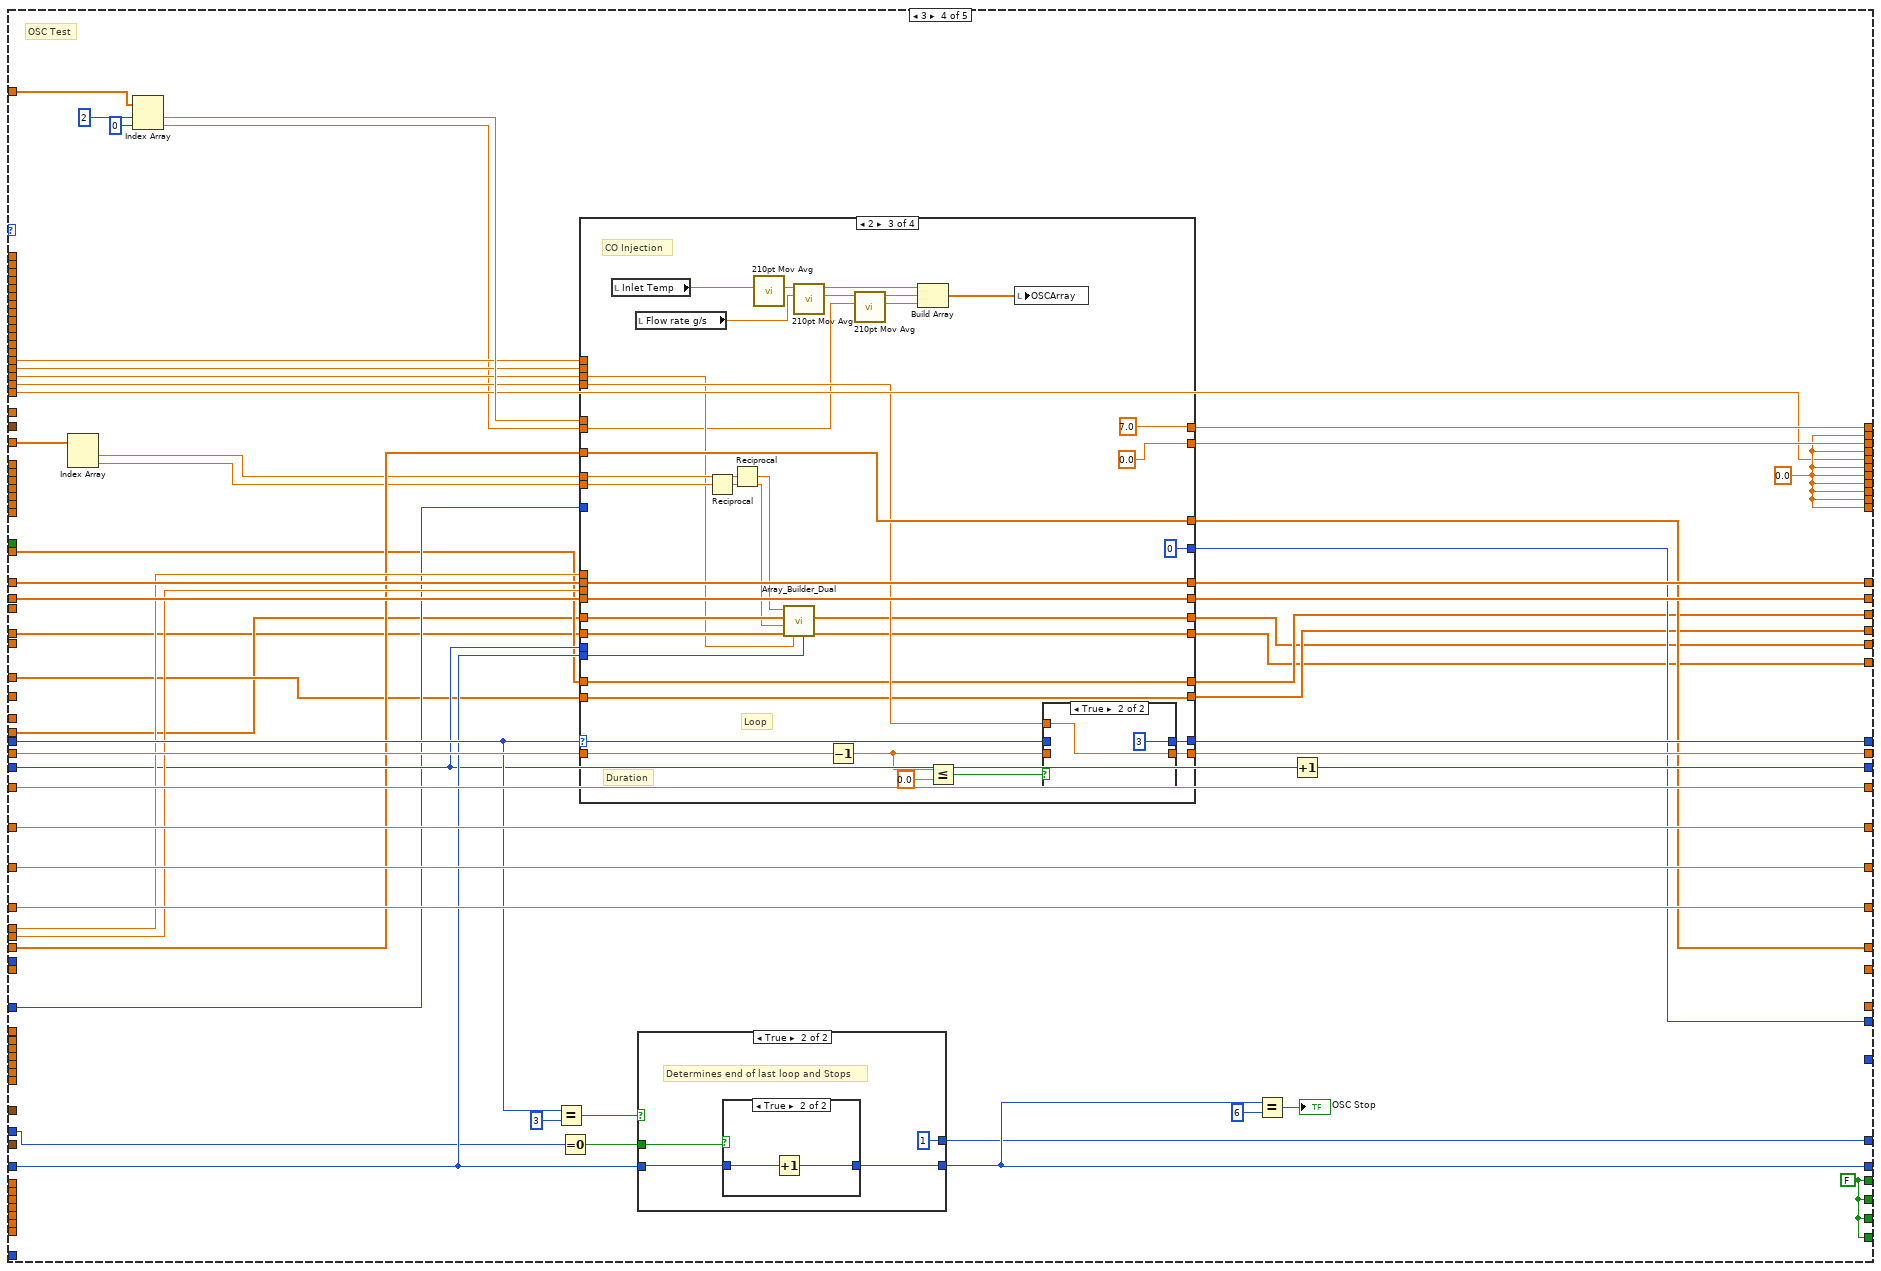
[diagram p14: hidden frame]
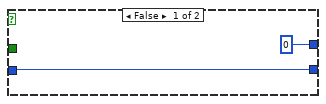
[diagram p15: hidden frame]
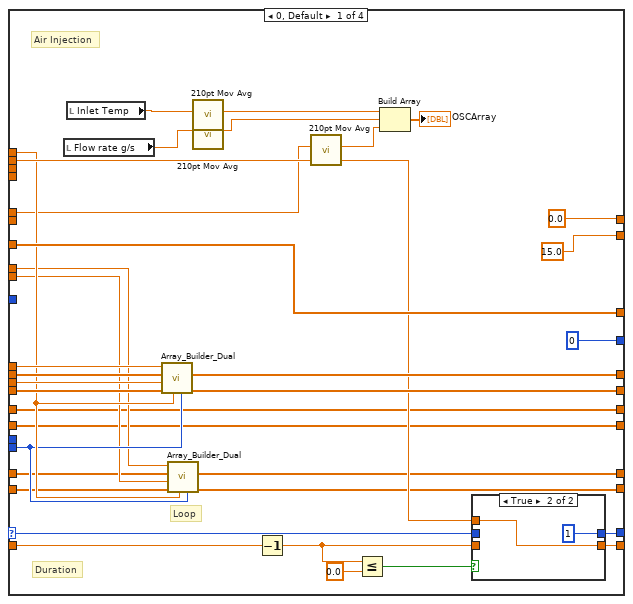
[diagram p17: hidden frame]
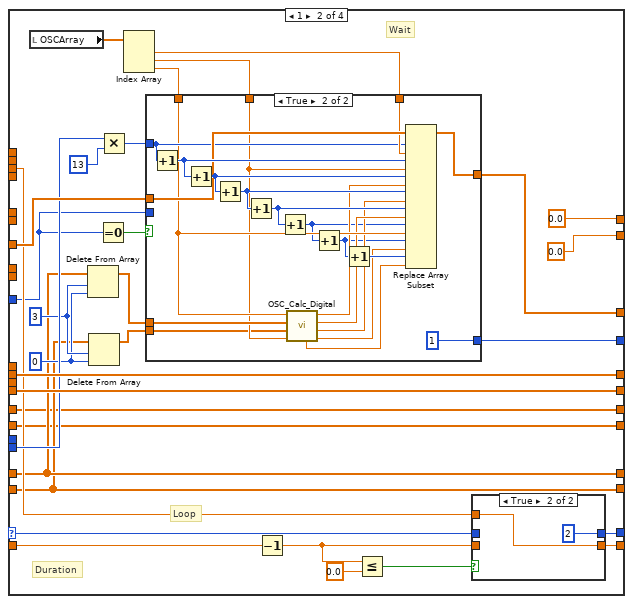
[diagram p19: hidden frame]
diagram:
  w4 = string[] ["", "Actual T", "Target T", "Delta T", "Previous Sp", "New Sp"]
  w1 = dbl[] [] ("Array Out Main")
  w21 = 0 ("t")
  w22 = i16 0
  w18 = dbl[] [] ("Array of Double")
  w14 = dbl[] [] ("Array of Double")
  w15 = dbl[] [] ("Array Out Main")
  w16 = 0.0 ("Furnace Set-point")
  w29 = 0 ("It Out")
  w25 = FALSE
  w30 = 0.0 ("Time to shut down 3")
  w2 = 0.0 ("output V")
  w34 = FALSE ("DIO On?")
  w23 = u16 0 ("UInt16")
  w53 = u16 0 ("length")
  # "00 Loop\n01 Leak Test Pass/Fail\n02 Error Out\n03 DI no 2\n04 Flow Venturi\n05 Flow Vane\n06 Etas 1\n07 Etas 2\n08 Uego 1\n09 Uego 2\n10 Tank Pressure\n11 TC 1\n12 TC 2\n13 TC 3\n14 TC 4\n15 TC 5\n16 TC 6\n17 TC 7\n18 TC 8\n19 TC 9\n20 TC 10\n21 TC 11\n22 TC 12\n23 TC 13\n24 TC 14\n25 TC 15\n26 TC 16\n27 TC Furnace\n28 Leak Test Time\n29 Cycle Time Step\n30 Heat Load Array\n31 HL 2\n32 HL 3\n33 HL 4\n34 HL 5\n35 HL 6\n36 HL 7\n37 HL 8\n38 HL 9\n39 HL 10\n40 HL 11\n41 Ageing Time"
  # "New Control Variables Array\n\n0 Stop Cmd\n1 Test Number\n2 Flow Rate\n3 Start Temperature\n4 Stop Temperature\n5 Furnace Ramp Rate\n6 Inlet O2\n7 CO Theory\n8 HC Theory\n9 Inlet Lambda Lean\n10 Inlet Temperature\n11 NO ppm SW\n12 NO ppm Loff\n13 NO:CO Ratio\n14 Temperature Limit\n15 Connected?  ****\n16 Inlet Temp Age\n17 Flow Rate Age\n\nAdv Settings\n\n18 CO Conc %\n19 HC Conc %\n20 NOx Conc %\n21 O2 Conc % \n22 Propane/Propylene\n23 Lambda P\n24 Lambda I\n25 Lambda D\n26 Purge Duration\n27 Target Furnace Lambda\n28 Cycle Length\n29 Heat Load Control\n30 Ref Temp\n31 C Factor\n32 Target Heat Load\n33 Control TC 1\n34 Control TC 2"
  # "1 DI no1 -errors\n1 DI no2 -states\n1 Flow rate 1 g/s\n1 Flow rate 2 g/s\n1 ECM AFR\n5 Mexa U\n5 Mexa D\n16 Temp I\n15 Temp II\n1 Furnace Temp 1\n1 Furnace Temp 2\n4 NOx\n4 EGO\n5 Mexa U 2\n5 MExa D 2"
  # "Control Variables Array\n\n0 Stop Cmd\n1 Test Number\n2 Flow Rate\n3 Start Temperature\n4 Stop Temperature\n5 Furnace Ramp Rate\n6 Inlet Lambda\n7 Inlet O2\n8 Inlet Lambda Rich\n9 Inlet Lambda Lean\n10 Inlet Temperature\n11 NO ppm SW\n12 NO ppm Loff\n13 NO:CO Ratio\n14 Temperature Limit\n15 Connected?  ****\n16 Inlet Temp Age\n17 Flow Rate Age\n\nAdv Settings\n\n18 NOx Conc\n19 CO Conc %\n20 HC Conc %\n21 Bleed H2O %\n22 Bleed CO2 %\n23 Bleed N2 %\n24 Lambda P\n25 Lambda I\n26 Lambda D\n27 Purge Duration\n28 Target Furnace Lambda\n29 HC Reaction ct\n30 Full System?\n\n31 Log Time\n32 Heat Load?\n33 Heat Load Constants"
  # "set safe values on critical outputs"
  # "Open one reference for each target"
  # "Set Shared Variable to safe values"
  # "Switch time"
  n1 = shared-variable "RT CompactRIO Target\\Library 1.lvlib\\Control Variables"(dbl[] [0.0, 0.0, 0.0, 0.0, 0.0, 0.0, 0.0, 0.0, 0.0, 0.0, 0.0, 0.0, 0.0, 0.0, 800.0, 0.0, 0.0, 0.0, 100.0, 100.0, 100.0, 100.0, 0.0, 0.0, 0.0, 0.0, 30.0, 1.0, 0.0, 0.0, 0.0, 0.0, 0.0, 1.0, 1.0, 0.0, 0.0, 20.0, 20.0, 250.0, 20.0, 100.0, 250.0, 20.0, 100.0, 100.0, 20.0, 100.0, 0.0, 0.0, 0.0, 1000.0, 50.0, 1200.0, 11.0, 12.0, 1.0, 10.0, 9.0, 0.0, 0.0, 0.0, 0.0, 0.0, 0.0, 0.0, 0.0, 0.0, 0.0, 0.0, 0.0, 0.0] ("Control Variables")) -> ()  [unwired: 1 in, 1 out]
  n2 = xnode "Open FPGA VI Reference"("resource name"=tag "rio://192.168.0.2/RIO0") -> ("FPGA VI Reference Out"=w24:refnum<k20>, "error out"=w33:errorcluster)  [unwired: 1 in]
  n3 = xnode "Open FPGA VI Reference"("resource name"=tag "rio:/169.254.0.13/RIO0") -> ("FPGA VI Reference Out"=w31:refnum<k20>, "error out"=w46:errorcluster)  [unwired: 1 in]
  n4 = xnode "Read/Write Control"("FPGA VI Reference In"=w31, "error in"=w46, "Command"=0, "Leak test on?"=w34, "DO On?"=w34) -> ("FPGA VI Reference Out"=w41:refnum<k20>, "error out"=w45:errorcluster)
  n5 = xnode "Read/Write Control"("FPGA VI Reference In"=w41) -> ("FPGA VI Reference Out"=w37:refnum<k20>, "error out"=w42:errorcluster)  [unwired: 5 in]
  n6 = Reshape Array(w4, 1 ("Settling Time"), 6 ("Settling Time")) -> (w5:string[][])
  n7 = Reshape Array(w4, 1 ("Settling Time"), 5 ("Settling Time")) -> (w6:string[][])
  n8 = Bundle(w6, w5, dbl[] [], "Furnace Set-point"=0.0, "It Out"=10) -> (w3:T8)  [unwired: 1 in]
  n9 = node-c288() -> (w50:T9)  [unwired: 4 in]
  n10 = node-c288("UEGO 3") -> (w28:T9)  [unwired: 3 in]
  n11 = node-c288(i64 1000 ("Period")) -> (w44:T9)  [unwired: 3 in]
  n12 = timed-loop {
    shift-right: [w327] -> _
    shift-left: w23 -> [w71]
    tunnel: w41 -> [w191]
    shift-right: [w326] -> _
    shift-left: w53 -> [w324]
    shift-right: [w325] -> _
    shift-left: w53 -> [w323]
    timing: w50 -> [_]
    timing-out: [_] -> w49
    shift-right: [w314] -> _
    shift-left: FALSE ("Alarm?") -> [_]
    tunnel: w24 -> [w275]
    tunnel: w45 -> [w296]
    shift-right: [w309] -> _
    shift-left: w2 -> [w308]
    shift-right: [w307] -> _
    shift-left: w2 -> [w306]
    shift-right: [w250] -> _
    shift-left: w30 -> [w253]
    shift-right: [w249] -> _
    shift-left: w25 -> [w150]
    shift-right: [w292] -> _
    shift-left: w23 -> [w77]
    shift-right: [w291] -> _
    shift-left: w29 -> [w289]
    shift-right: [w290] -> _
    shift-left: w16 -> [w288]
    shift-right: [w162] -> _
    shift-left: _ -> [w286]
    shift-right: [w166] -> _
    shift-left: _ -> [w285]
    tunnel: [w279] -> w36
    tunnel: [w278] -> w35
    shift-right: [w262] -> _
    shift-left: w29 -> [w263]
    shift-right: [w165] -> _
    shift-left: w15 -> [w226]
    shift-right: [w255] -> _
    shift-left: w2 -> [w256]
    shift-right: [w247] -> _
    shift-left: w30 -> [w248]
    shift-right: [w243] -> _
    shift-left: _ -> [w245]
    shift-right: [w242] -> _
    shift-left: _ -> [w244]
    shift-right: [w240] -> _
    shift-left: w1 -> [w241]
    shift-right: [w231] -> _
    shift-left: w15 -> [w233]
    shift-right: [w230] -> _
    shift-left: w15 -> [w232]
    shift-right: [w194] -> _
    shift-left: _ -> [w197]
    shift-right: [w193] -> _
    shift-left: w25 -> [w192]
    shift-right: [w187] -> _
    shift-left: _ -> [w188]
    shift-right: [w125] -> _
    shift-left: w2 -> [w124]
    shift-right: [w121] -> _
    shift-left: w2 -> [w123]
    shift-right: [w116] -> _
    shift-left: u32 600 ("number") -> [w115]
    shift-right: [w83] -> _
    shift-left: w16 -> [w84]
    shift-right: [w69] -> _
    shift-left: w3 -> [w70]
    shift-right: [w68] -> _
    shift-left: w3 -> [w67]
    shift-right: [w66] -> _
    shift-left: w2 -> [w65]
    shift-right: [w58] -> _
    shift-left: w1 -> [w59]
    stop <- "STOP" stop-if-true
    w210 = 4 ("index")
    w211 = 4 ("index")
    # "Tank Temp Limit"
    # "Set Temp Limit"
    # "Fan Bearing Limit"
    # "UEGO FUR 1"
    # "Cycle Length"
    # "30"
    # "25"
    # "20"
    # "10"
    # "5"
    # "30"
    # "25"
    # "20"
    # "10"
    # "5"
    # "0"
    # "Pressure calib"
    # "Furnace 1"
    # "tank P"
    # "CONTROL LOOP"
    # "TC I"
    n13 = node-c288() -> (→"Iteration Duration 2":i64)  [unwired: 1 in]
    n14 = local read "Control Variables"() -> (w139:dbl[])
    n15 = xnode "Read/Write Control"("FPGA VI Reference In"=w191, "error in"=w296) -> ("Array 1 In"=w107:fxp<+/-,35,9>[])  [unwired: 2 out]
    n16 = local read "Cycle Length"() -> (w223:i32)
    n17 = Index Array(array=i32[] [34, 33, 58, 54, 55, 59]) -> (element #1=w135:i32, element #2=w134:i32, element #3=w132:i32, element #4=w133:i32, element #5=w131:i32, element #6=w109:i32)  [unwired: 6 in]
    n18 = Index Array(array=w107, index=27) -> (element=w104:fxp<+/-,35,9>)
    n19 = Delete From Array(array=w107, length=18 ("index"), index=5 ("length")) -> (deleted portion=w102:fxp<+/-,35,9>[])  [unwired: 1 out]
    n20 = Delete From Array(array=w107, length=4, index=23) -> (deleted portion=w339:fxp<+/-,35,9>[])  [unwired: 1 out]
    n21 = Index Array(array=w139) -> (element #1=w337:dbl, element #2=w151:dbl, element #3=w336:dbl, element #4=w335:dbl, element #5=w311:dbl, element #6=w334:dbl, element #9=w332:dbl, element #10=w331:dbl, element #11=w158:dbl, element #12=w330:dbl, element #13=w329:dbl, element #14=w328:dbl, element #19=w305:dbl, element #20=w304:dbl, element #21=w159:dbl, element #22=w303:dbl, element #23=w302:dbl, element #24=w301:dbl, element #25=w299:dbl, element #26=w298:dbl, element #27=w297:dbl, element #28=w300:dbl, element #29=w154:dbl, element #30=w155:dbl, element #31=w152:dbl, element #32=w160:dbl, element #33=w153:dbl, element #34=w283:dbl, element #35=w282:dbl)  [unwired: 35 in, 6 out]
    n22 = Index Array(array=w139, index #1=w135, index #2=w134, index #3=w132, index #4=w133, index #5=w131, index #6=w109) -> (element #1=w180:dbl, element #2=w179:dbl, element #3=w178:dbl, element #4=w138:dbl, element #5=w137:dbl, element #6=w114:dbl)
    n23 = Decrement(x=w178) -> (x-1=w176:dbl)
    n24 = Decrement(x=w114) -> (x-1=w113:dbl)
    n25 = Index Array(array=w139, index #1=52 ("index"), index #2=51 ("index"), index #3=53 ("index")) -> (element #1=w182:dbl, element #2=w120:dbl, element #3=w181:dbl)
    n26 = call "TC calibrate_v2.vi"("TC in"=w102) -> ("TC out"=w55:sgl[])  [unwired: 10 in]
    n27 = call "Array to temp.vi"("Array"=w339) -> ("Temperature"=w105:sgl)  [unwired: 10 in]
    n28 = Index Array(array=w107, index #1=0 ("length"), index #2=28 ("index"), index #3=29 ("index"), index #4=30 ("index"), index #5=31 ("index")) -> (element #1=w228:fxp<+/-,35,9>, element #2=w94:fxp<+/-,35,9>, element #3=w95:fxp<+/-,35,9>, element #4=w96:fxp<+/-,35,9>, element #5=w97:fxp<+/-,35,9>)
    n29 = Divide(x=w223, y=10.0) -> (x/y=w189:dbl)
    n30 = Decrement(x=w179) -> (x-1=w177:dbl)
    n31 = Decrement(x=w137) -> (x-1=w174:dbl)
    n32 = xnode "Read/Write Control"("FPGA VI Reference In"=w191, "Emission SV 1"=w150, "Emission SV 2"=w192) -> ()  [unwired: 1 in, 2 out]
    n33 = Decrement(x=w180) -> (x-1=w173:dbl)
    n34 = Decrement(x=w138) -> (x-1=w175:dbl)
    n35 = call "31pt Mov Avg.vi"("Value in"=w94) -> ("Value out"=w93:dbl)  [unwired: 10 in]
    n36 = call "31pt Mov Avg.vi"("Value in"=w97) -> ("Value out"=w90:dbl)  [unwired: 10 in]
    n37 = Build Array(w152, w160, w153, w283, w282) -> (w222:dbl[])
    n38 = local read "UEGO Sensor Results"() -> (w272:T2)
    n39 = Index Array(array=w55, index #1=w173, index #2=w177, index #3=w176, index #4=w175, index #5=w174, index #6=w113) -> (element #1=w142:sgl, element #2=w119:sgl, element #3=w170:sgl, element #4=w171:sgl, element #5=w172:sgl, element #6=w112:sgl)
    "Inlet Temp" <- w119
    n40 = call "31pt Mov Avg.vi"("Value in"=w228) -> ("Value out"=w287:dbl)  [unwired: 10 in]
    n41 = call "31pt Mov Avg.vi"("Value in"=w95) -> ("Value out"=w92:dbl)  [unwired: 10 in]
    n42 = expression code="0.02*x+3"("TankHi") -> (w317:dbl)
    n43 = expression code="0.02*x+3"("TankLo") -> (w318:dbl)
    n44 = Index Array(array=w222, index=3) -> (element=w265:dbl)
    n45 = Index Array(array=w222, index=4) -> (element=w260:dbl)
    n46 = call "31pt Mov Avg.vi"("Value in"=w96) -> ("Value out"=w91:dbl)  [unwired: 10 in]
    n47 = Not(x=w150) -> ()  [unwired: 1 out]
    n48 = Greater?(x=w171, y=w182) -> (0:w146:bool)
    n49 = Greater?(x=w172, y=w182) -> (0:w145:bool)
    n50 = Greater?(x=w112, y=sgl 280.0) -> (0:w111:bool)
    n51 = Decrement(x=w265) -> (x-1=w264:dbl)
    n52 = Decrement(x=w260) -> (x-1=w261:dbl)
    n53 = Greater Or Equal?(x=w119, y=w120) -> (x >= y?=w143:bool)
    n54 = expression code="50*x-150"(w93) -> (w89:dbl)
    n55 = expression code="50*x-150"(w90) -> (w86:dbl)
    n56 = call "Fur_Limit.vi"("Furnace Temp"=w105, "Eurotherm Input"=w104, "Fur Limit"="Power Limit") -> ("Signal Out"=w85:dbl)  [unwired: 8 in]
    n57 = Index Array(array=w55, index=w264) -> (element=w237:sgl)
    n58 = Index Array(array=w55, index=w261) -> (element=w236:sgl)
    n59 = xnode "Read/Write Control"("FPGA VI Reference In"=w191, "error in"=w296, "TankHi"=w317, "TankLo"=w318, "ISO1_SV"=w150) -> ("FPGA VI Reference Out"=w157:refnum<k20>, "DI no 1"=w156:u16, "DI no 2"=w294:u8)  [unwired: 1 out]
    "DI no1" <- w156
    n60 = Greater Or Equal?(x=w142, y=w120) -> (x >= y?=w141:bool)
    n61 = Greater?(x=w119, y=w181) -> (0:w144:bool)
    n62 = Equal?(x=w71, y=u32 2) -> (x = y?=w75:bool)
    n63 = Equal?(x=w71, y=u32 3) -> (x = y?=w76:bool)
    n64 = Unbundle By Name(w272) -> ("UEGO1Lambda"=w212:sgl, "UEGO2Lambda"=w190:sgl)
    n65 = expression code="50*x-150"(w92) -> (w88:dbl)
    n66 = Boolean To (0,1)(Boolean=w150) -> ()  [unwired: 1 out]
    n67 = call "Mov_Avg_JS_Dual.vi"("Cycle Length"=w223, "Array In 2"=w232, "Input 2"=w236, "Array In"=w233, "Input"=w237) -> ("Array Out Main 2"=w230:dbl[], "Mean 2"=w234:dbl, "Array Out Main"=w231:dbl[], "Mean"=w235:dbl)  [unwired: 3 in]
    n68 = Or(x=w75, y=w76) -> (x .or. y?=w72:bool)
    n69 = Build Array(w146, w145, w141, w143, w144, w111) -> (w140:bool[])
    n70 = Not Equal To 0?(x=w337) -> (x != 0?=w322:bool)
    n71 = local read "Flow 1"() -> (w202:dbl)
    n72 = Decrement(x="Control TC 2") -> (x-1=w81:i32)
    n73 = Decrement(x="Tc") -> (x-1=w57:i32)
    n74 = Decrement(x="Control TC") -> (x-1=w204:i32)
    n75 = call "Heat_Load_Calc_Red.vi"("Input Array 2"=w285, "Input Array"=w222, "Avg Temp In"=w235, "Temp In"=w237) -> ("Output Array"=w224:dbl[])  [unwired: 4 in, 3 out]
    n76 = call "Heat_Load_Calc_Red.vi"("Input Array 2"=w226, "Input Array"=w222, "Avg Temp In"=w234, "Temp In"=w236) -> ("Output Array"=w225:dbl[])  [unwired: 4 in, 3 out]
    n77 = expression code="50*x-150"(w91) -> (w87:dbl)
    n78 = Not Equal To 0?(x=w155) -> (x != 0?=w310:bool)
    n79 = Multiply(x="Sw time", y=2.0) -> (x*y=w200:dbl)
    n80 = call "Error handler.vi"("Test Alarms"=w77, "DI no 1 in"=w156, "Stop Test"=w322, "Alarm Input Array"=w140) -> ("Alarm?"=w314:bool, "Loop out"=w321:u16, "Error no out"=w295:dbl)  [unwired: 5 in]
    n81 = Index Array(array=w55, index=w81) -> (element=w79:sgl)
    n82 = Index Array(array=w55, index=w57) -> (element=w54:sgl)
    n83 = Build Array (concatenate)(w55, w105) -> (w185:sgl[])
    n84 = Index Array(array=w55, index=w204) -> (element=w184:sgl)
    n85 = Equal?(x="Sw time", y=w253) -> (x = y?=w254:bool)
    n86 = Equal?(x=w200, y=w197) -> (x = y?=w201:bool)
    n87 = local read "UEGO Array"() -> (w227:dbl[])
    n88 = call "Flow_Selection.vi"("Offset"="Flow Offset", "Linearized Temperature"=w170, "Flow"=w202, "Pressure Transducer 2"="P-Transducer 1") -> ("Flow rate g/s"=w238:dbl)  [unwired: 6 in, 1 out]
    "Flow rate g/s" <- w238
    n89 = And(x=w314, y=w72) -> (x .and. y?=w313:bool)
    n90 = Build Array(w89, w88, w87, w86) -> (w82:dbl[])
    n91 = case shown="False" w254 {
      tunnel: [w352 w354] -> w251
      tunnel: w150 -> [w352 w355]
      tunnel: [w351 0.0] -> w252
      tunnel: w253 -> [w350 _]
      frame False {
        n92 = Increment(x=w350) -> (x+1=w351:dbl)
      }
      frame True {
        n93 = Not(x=w355) -> (.not. x?=w354:bool)
      }
    }
    n94 = case shown="False" w201 {
      tunnel: [w346 w348] -> w195
      tunnel: w192 -> [w346 w349]
      tunnel: [w345 0.0] -> w196
      tunnel: w197 -> [w344 _]
      frame False {
        n95 = Increment(x=w344) -> (x+1=w345:dbl)
      }
      frame True {
        n96 = Not(x=w349) -> (.not. x?=w348:bool)
      }
    }
    n97 = Build Array(w295, w294, w238, 0.0 ("element")) -> (w293:dbl[])
    n98 = call "Mov_Avg_JS_Dual.vi"("Cycle Length"=w189, "Array In"=w188, "Input"=w184) -> ("Array Out Main"=w187:dbl[], "Mean"=→"Avg Control":dbl)  [unwired: 5 in, 2 out]
    n99 = expression code="50*x-150"(w287) -> (w229:dbl)
    "Tank Pressure" <- w229
    n100 = Select(t=w321, s=w313, f=w71) -> (s? t:f=w78:i32)
    "Loop No." <- w78
    n101 = call "Invertor rate calc.vi"("PID gains"="PID Inverter", "V Max Flow"=sgl 10.0, "process variable g/s"=w124, "User setpoint g/s"=w123) -> ("output V"=w129:dbl)  [unwired: 5 in, 2 out]
    n102 = call "10pt Mov Avg.vi"("Value in"=w129) -> ("Value out"=w128:dbl)  [unwired: 10 in]
    n103 = Build Array (concatenate)(w227, w229, w185) -> (w273:dbl[])
    n104 = Build Array (concatenate)(w293, w273) -> (w274:dbl[])
    n105 = case shown="True" "Reset AM 1" {
      tunnel: [w361 dbl[] [] ("Output Array")] -> w166
      tunnel: w224 -> [w361 _]
      tunnel: "Reset AM 1" -> [w360 _]
      tunnel: [w360 FALSE ("Reset Heat Load")] -> w266
      frame False {
      }
      frame True {
      }
    }
    n106 = case shown="False" "Reset AM 2" {
      tunnel: [w357 dbl[] [] ("Output Array")] -> w165
      tunnel: w225 -> [w357 _]
      tunnel: "Reset AM 2" -> [w356 _]
      tunnel: [w356 FALSE ("Reset Heat Load")] -> w258
      frame False {
      }
      frame True {
      }
    }
    n107 = local write "Reset AM 1"(w266) -> ()
    n108 = local write "Reset AM 2"(w258) -> ()
    n109 = call "Heat_Load_Control.vi"("Heat Load Control"="Ageing Metric\nControl", "Catalyst 2"=w165, "Catalyst 1"=w166) -> ("Control Cat"=w221:dbl)  [unwired: 7 in, 1 out]
    n110 = case shown="2" w78 {
      tunnel: w157 -> [w381 w402 w464 w568 _ w1073]
      tunnel: [w383 2 w468 w584 w1054 u16 0 ("length")] -> w327
      tunnel: w238 -> [_ _ w418 w585 _ _]
      tunnel: w335 -> [_ _ w459 w520 _ _]
      tunnel: w336 -> [_ _ _ w586 _ _]
      tunnel: w334 -> [_ w401 _ _ _ _]
      tunnel: w311 -> [_ _ _ w583 _ _]
      tunnel: w151 -> [_ _ w458 w582 _ _]
      tunnel: w229 -> [_ _ _ w581 _ _]
      tunnel: w332 -> [_ _ _ w574 _ _]
      tunnel: w331 -> [_ _ _ w575 _ _]
      tunnel: w158 -> [_ _ w460 w578 _ _]
      tunnel: w324 -> [_ _ _ w580 _ _]
      tunnel: [w384 w405 w467 w579 w1053 w1072] -> w326
      tunnel: w323 -> [_ _ _ w577 _ _]
      tunnel: [w384 w405 w467 w576 w1053 w1072] -> w325
      tunnel: w330 -> [_ _ _ w573 _ _]
      tunnel: w329 -> [_ _ _ w572 _ _]
      tunnel: w328 -> [_ _ _ w571 _ _]
      tunnel: w305 -> [_ _ _ w570 _ _]
      tunnel: [w380 1 2 3 4 5] -> w333
      tunnel: w304 -> [_ _ _ w567 _ _]
      tunnel: w159 -> [_ _ _ w556 _ _]
      tunnel: w301 -> [_ _ _ w566 _ _]
      tunnel: w302 -> [_ _ _ w565 _ _]
      tunnel: [w380 0 0 w564 0 0] -> w316
      tunnel: "NO PID Sweep Test" -> [_ _ _ w563 _ _]
      tunnel: w300 -> [_ _ w430 _ _ _]
      tunnel: w303 -> [_ _ _ w561 _ _]
      tunnel: w310 -> [_ _ _ w562 _ _]
      tunnel: [_ _ _ w560 _ _] -> w309
      tunnel: w308 -> [_ _ _ w559 _ _]
      tunnel: [_ _ _ w558 _ _] -> w307
      tunnel: w306 -> [_ _ _ w557 _ _]
      tunnel: w299 -> [_ _ _ _ _ _]
      tunnel: w298 -> [_ _ _ _ _ _]
      tunnel: w297 -> [_ _ _ _ _ _]
      tunnel: [w379 w396 w457 w555 w1046 _] -> w292
      tunnel: w77 -> [w379 w396 w457 w554 w1046 _]
      tunnel: w105 -> [_ _ w453 w553 _ _]
      tunnel: [_ _ _ w552 _ _] -> w291
      tunnel: [_ _ _ w551 _ _] -> w290
      tunnel: w289 -> [_ _ _ w550 _ _]
      tunnel: w288 -> [_ _ _ w549 _ _]
      tunnel: [0.0 ("Numeric") 0.0 ("Numeric") w420 w547 0.0 ("Numeric") 0.0 ("Numeric")] -> w162
      tunnel: w286 -> [_ _ _ w548 _ _]
      tunnel: w153 -> [_ _ _ w546 _ _]
      tunnel: "Furnace Manual" -> [_ _ _ w545 _ _]
      tunnel: [u8[] [64, 160, 0, 0, 133, 108, 64, 160, 0, 0, 133, 108] ("SP&CRC") u8[] [64, 160, 0, 0, 133, 108, 64, 160, 0, 0, 133, 108] ("SP&CRC") w422 w544 w1036 u8[] [64, 160, 0, 0, 133, 108, 64, 160, 0, 0, 133, 108] ("SP&CRC")] -> w280
      tunnel: "Furnace SP" -> [_ _ w424 w543 _ _]
      tunnel: "Fan PID" -> [_ _ w451 w542 _ _]
      tunnel: 400 ("y") -> [_ _ _ w541 _ _]
      tunnel: 10.0 ("y") -> [_ _ _ w540 _ _]
      tunnel: w190 -> [_ _ w421 w539 _ _]
      tunnel: 300 ("y") -> [_ _ _ w538 _ _]
      tunnel: w263 -> [_ _ w441 _ _ _]
      tunnel: w119 -> [_ _ w439 _ _ _]
      tunnel: [_ _ w440 0 ("index") _ _] -> w262
      tunnel: w256 -> [_ _ _ w536 _ _]
      tunnel: [_ _ w423 _ _ _] -> w255
      tunnel: w142 -> [_ _ w433 _ _ _]
      tunnel: w252 -> [_ _ w432 w535 _ _]
      tunnel: w251 -> [_ _ w431 w534 _ _]
      tunnel: [w376 w393 w432 w535 w1039 w1063] -> w250
      tunnel: [w375 w392 w431 w534 w1038 w1062] -> w249
      tunnel: w248 -> [_ _ _ w533 w1041 _]
      tunnel: [w376 w393 w430 w533 w1040 w1063] -> w247
      tunnel: w189 -> [_ _ _ w532 _ _]
      tunnel: w245 -> [_ _ _ w531 _ _]
      tunnel: w244 -> [_ _ _ w530 _ _]
      tunnel: [_ _ _ w529 _ _] -> w243
      tunnel: [_ _ _ w528 _ _] -> w242
      tunnel: w241 -> [_ _ w417 w527 _ _]
      tunnel: [_ _ w416 w526 _ _] -> w240
      tunnel: w221 -> [_ _ _ w525 _ _]
      tunnel: w212 -> [_ _ w427 _ _ _]
      tunnel: w184 -> [_ _ _ w524 _ _]
      tunnel: w196 -> [_ _ w426 w523 _ _]
      tunnel: w195 -> [_ _ w425 w522 _ _]
      tunnel: [w376 w393 w426 w523 w1039 w1063] -> w194
      tunnel: [w375 w392 w425 w522 w1038 w1062] -> w193
      tunnel: [0.0 ("Value out") 0.0 ("Value out") w423 w521 0.0 ("Value out") 0.0 ("Value out")] -> w183
      tunnel: w154 -> [_ _ w420 _ _ _]
      tunnel: w128 -> [_ _ w413 w519 _ _]
      tunnel: "Fan Speed V" -> [_ _ w414 w518 _ _]
      tunnel: [w372 w390 w412 w516 w1035 w1060] -> w125
      tunnel: "Set-point Fan" -> [_ _ w411 w517 _ _]
      tunnel: [w372 w390 w411 w517 w1035 w1060] -> w121
      tunnel: [u32 600 ("number") u32 600 ("number") u32 600 ("number") w515 u32 600 ("number") u32 600 ("number")] -> w116
      tunnel: w115 -> [_ _ _ w514 _ _]
      tunnel: w79 -> [_ _ _ w513 _ _]
      tunnel: w70 -> [w370 w388 w409 w512 w1033 w1058]
      tunnel: [w370 w388 w409 w511 w1033 w1058] -> w69
      tunnel: [w369 w387 w407 w510 w1032 w1057] -> w68
      tunnel: w67 -> [w369 w387 w407 w509 w1032 w1057]
      tunnel: [w368 w386 w408 w508 w1031 w1056] -> w66
      tunnel: w65 -> [w368 w386 w408 w507 w1031 w1056]
      tunnel: w59 -> [w367 w385 w406 w506 w1030 w1055]
      tunnel: [w367 w385 w406 w505 w1030 w1055] -> w58
      tunnel: w54 -> [_ _ _ w504 _ _]
      frame 0, Default {
        w372 = 0.0 ("Set-point Fan")
        w376 = 0.0 ("Sw time")
        w375 = FALSE
        w380 = 0
        w384 = u16 0 ("length")
        n111 = local write "Lambda Avg"(1.0 ("Uego Avg")) -> ()
        n112 = xnode "Read/Write Control"("FPGA VI Reference In"=w381, "Command"=0) -> ()  [unwired: 1 in, 2 out]
        n113 = shared-variable "RT CompactRIO Target\\Library 1.lvlib\\Enum 1"() -> (w383:u16)  [unwired: 1 in, 1 out]
      }
      frame 1 {
        w390 = 0.0 ("Set-point Fan")
        w393 = 0.0 ("Sw time")
        w392 = FALSE
        w405 = u16 0
        # "Initialise"
        n114 = call "Furnace rate SP calc.vi"("SP"=w401) -> ("SP&CRC"=w397:u8[])  [unwired: 10 in]
        n115 = xnode "Read/Write Control"("FPGA VI Reference In"=w402, "Ramp rate,SP&CRC"=w397, "Command"=i16 1, "DO On?"=TRUE) -> ()  [unwired: 1 in, 2 out]
      }
      frame 2 {
        (unwired) u16 0 ("UInt16")
        w467 = u16 0
        # "Buildup"
        # "Ageing Time"
        n116 = xnode "Read/Write Control"("FPGA VI Reference In"=w464, "Command"=0, "DO On?"=TRUE) -> ()  [unwired: 1 in, 2 out]
        n117 = Equal To 0?(x=w441) -> ()  [unwired: 1 out]
        n118 = case shown="3" w458 {
          tunnel: w459 -> [_ _ _ _ _]
          tunnel: w460 -> [_ _ _ _ _]
          tunnel: ["CO Furnace Inlet" "HC Furnace Inlet" "NO Furnace Inlet" "OSC Furnace Inlet" "Age Furnace Inlet"] -> w445
          tunnel: ["CO Lam Lim" "HC Lam lim" "NO Lam Lim" "OSC Lam lim" "Age Lam Lim"] -> w456
          frame 0, Default {
          }
          frame 1 {
          }
          frame 2 {
          }
          frame 3 {
          }
          frame 4 {
          }
        }
        n119 = case shown="False" FALSE {
          tunnel: [w475 "Furnace 1"] -> w454
          tunnel: w453 -> [_ w484]
          tunnel: [TRUE w482] -> w438
          tunnel: w433 -> [w481 _]
          tunnel: w445 -> [w477 _]
          tunnel: w439 -> [w474 _]
          tunnel: [w476 FALSE] -> w435
          tunnel: w424 -> [w475 _]
          frame False {
            w473 = sgl 10.0 ("y")
            # "Furnace PID Based on Tin"
            n120 = Subtract(x=w474, y=w473) -> (x-y=w479:sgl)
            n121 = Add(x=w474, y=w473) -> (x+y=w478:sgl)
            n122 = call "Furnace PID SP 1.vi"("PV deg C"=w481, "User SP Deg C"=w477) -> ()  [unwired: 8 in, 2 out]
            n123 = In Range and Coerce(upper limit=w478, x=w477, lower limit=w479) -> (In Range?=w476:bool)  [unwired: 1 out]
          }
          frame True {
            # "Initial Temperature Ramp @ 1V"
            n124 = Subtract(x="Furnace 1", y=sgl 10.0) -> (x-y=w487:sgl)
            n125 = Add(x=sgl 10.0, y="Furnace 1") -> (x+y=w489:sgl)
            n126 = In Range and Coerce(upper limit=w489, x=w484, lower limit=w487) -> (In Range?=w482:bool)  [unwired: 1 out]
          }
        }
        n127 = call "Mov_Avg_JS.vi"("Array In"=w417, "Cycle Length"=60.0, "Input"=w418) -> ("Array Out Main"=w416:dbl[], "Mean"=w412:dbl)  [unwired: 7 in]
        n128 = Greater Or Equal?(x=w456, y=w421) -> ()  [unwired: 1 out]
        n129 = call "72pt Mov Avg.vi"("Value in"=w418) -> ("Value out"=w434:dbl)  [unwired: 10 in]
        n130 = Subtract(x=w434, y=sgl 3.0) -> (x-y=w449:dbl)
        n131 = Add(x=sgl 3.0, y=w434) -> (x+y=w450:dbl)
        n132 = Less?(x=w427, y=sgl 5.0) -> (x < y?=w436:bool)
        n133 = case shown="True" w438 {
          tunnel: [sgl 1.0 ("y") w493] -> w452
          tunnel: w413 -> [_ w493]
          frame False {
            # "Initial Fan SP"
          }
          frame True {
            # "Fan Control\nOnce Furnace Reaches SP"
          }
        }
        n134 = In Range and Coerce(upper limit=w450, x=w412, lower limit=w449) -> (In Range?=w437:bool)  [unwired: 1 out]
        n135 = And(x=w438, y=w437) -> (x .and. y?=w444:bool)
        n136 = Equal To 0?(x=w441) -> (x = 0?=w442:bool)
        n137 = And(x=w444, y=w442) -> (x .and. y?=w443:bool)
        n138 = Compound Arithmetic op=AND(w435, w437, w436) -> (w428:bool)
        "Ready" <- w428
        n139 = case shown="True" w443 {
          tunnel: w441 -> [w471 _]
          tunnel: [w471 1 ("index")] -> w440
          frame False {
          }
          frame True {
            # "Turns on Furnace PID"
          }
        }
        n140 = case shown="True" w428 {
          tunnel: [FALSE "Start Test"] -> w429
          frame False {
          }
          frame True {
          }
        }
        n141 = case shown="False" w451 {
          tunnel: w452 -> [_ w491]
          tunnel: [w490 w491] -> w423
          tunnel: w414 -> [w490 _]
          frame False {
            # "Fan Manual"
          }
          frame True {
          }
        }
        n142 = call "Furnace SP calc.vi"("SP"=w454) -> ("SP&CRC"=w422:u8[])  [unwired: 10 in]
        n143 = Select(t=3, s=w429, f=2) -> (s? t:f=w468:i32)
      }
      frame 3 {
        n144 = case shown="3" w582 {
          tunnel: w586 -> [_ _ w665 _ _]
          tunnel: w585 -> [w598 w624 w649 w692 w892]
          tunnel: [w610 w636 w670 w710 w909] -> w584
          tunnel: w583 -> [w607 w634 w669 _ _]
          tunnel: w581 -> [_ _ _ _ w895]
          tunnel: w580 -> [_ _ _ _ _]
          tunnel: [w608 w633 w672 w713 w912] -> w579
          tunnel: w578 -> [_ _ _ _ _]
          tunnel: w577 -> [_ _ _ _ _]
          tunnel: [w608 w633 w672 w713 w912] -> w576
          tunnel: w575 -> [_ _ _ _ _]
          tunnel: w574 -> [_ _ _ _ _]
          tunnel: w573 -> [_ _ _ _ _]
          tunnel: w572 -> [_ _ w661 _ _]
          tunnel: w571 -> [_ _ w659 _ _]
          tunnel: w570 -> [_ _ w660 _ _]
          tunnel: w568 -> [_ _ _ _ _]
          tunnel: [0 0 0 0 0] -> w564
          tunnel: w567 -> [_ _ w658 _ _]
          tunnel: w556 -> [_ _ _ _ _]
          tunnel: w566 -> [_ _ _ _ _]
          tunnel: w565 -> [_ _ _ _ _]
          tunnel: w563 -> [_ _ _ _ _]
          tunnel: w562 -> [_ _ _ _ w882]
          tunnel: w561 -> [_ _ _ _ _]
          tunnel: [_ _ _ w700 w749] -> w560
          tunnel: w559 -> [_ _ _ w708 w908]
          tunnel: [_ _ _ w700 w749] -> w558
          tunnel: w557 -> [_ _ _ w707 w907]
          tunnel: w518 -> [w603 w626 w650 w700 w750]
          tunnel: [_ _ _ _ w889] -> w555
          tunnel: w554 -> [_ _ _ _ _]
          tunnel: w553 -> [_ _ _ w703 w898]
          tunnel: [_ _ _ w702 w897] -> w552
          tunnel: [_ _ _ w701 w831] -> w551
          tunnel: w550 -> [_ _ _ w705 w900]
          tunnel: w549 -> [_ _ _ w704 w899]
          tunnel: w548 -> [_ _ _ _ w906]
          tunnel: [_ _ _ _ w903] -> w547
          tunnel: w546 -> [_ _ _ _ w902]
          tunnel: w545 -> [_ _ _ w706 w901]
          tunnel: [w595 w621 w646 w684 w884] -> w544
          tunnel: w543 -> [_ _ _ w699 w896]
          tunnel: w542 -> [w602 w627 w651 w698 w880]
          tunnel: w541 -> [_ _ _ _ _]
          tunnel: w540 -> [_ _ _ _ _]
          tunnel: w539 -> [_ _ w654 _ w883]
          tunnel: w538 -> [_ _ _ _ _]
          tunnel: w536 -> [_ _ _ _ _]
          tunnel: w532 -> [_ _ _ w689 w747]
          tunnel: w531 -> [_ _ _ w697 w894]
          tunnel: w530 -> [_ _ _ w696 w893]
          tunnel: [_ _ _ w694 w842] -> w529
          tunnel: [_ _ _ w693 w840] -> w528
          tunnel: w527 -> [w601 w629 w653 w691 w891]
          tunnel: [w600 w628 w652 w690 w890] -> w526
          tunnel: w525 -> [_ _ _ _ w888]
          tunnel: w524 -> [w599 w625 w648 w686 w887]
          tunnel: [w594 w620 w647 w685 w885] -> w521
          tunnel: w520 -> [_ _ _ _ _]
          tunnel: w519 -> [w592 w618 w645 w682 w879]
          tunnel: [w593 w619 w644 w681 w878] -> w516
          tunnel: [u32 600 ("number") u32 600 ("number") u32 600 ("number") u32 600 ("number") w850] -> w515
          tunnel: w514 -> [_ _ _ _ w849]
          tunnel: w513 -> [_ _ _ _ w839]
          tunnel: w512 -> [w590 w616 w642 w678 w838]
          tunnel: [w590 w616 w642 w678 w830] -> w511
          tunnel: [w589 w615 w641 w677 w820] -> w510
          tunnel: w509 -> [w589 w615 w641 w677 w813]
          tunnel: [w588 w614 w640 w676 w812] -> w508
          tunnel: w507 -> [w588 w614 w640 w676 w811]
          tunnel: w506 -> [w587 w613 w639 w675 w742]
          tunnel: [w587 w613 w639 w675 w741] -> w505
          tunnel: w504 -> [_ _ _ _ w737]
          frame 0, Default {
            w608 = u16 0
            # "1Hz MFC's\n\n0. CO2\n1. N2\n2. SO2\n3. H2O\n4. N2P"
            # "CO Light-Off"
            n145 = Greater Or Equal?(x=w599, y=w607) -> (x >= y?=w609:bool)
            n146 = call "Mov_Avg_JS.vi"("Array In"=w601, "Cycle Length"=60.0, "Input"=w598) -> ("Array Out Main"=w600:dbl[], "Mean"=w593:dbl)  [unwired: 7 in]
            n147 = case shown="True" w602 {
              tunnel: [w611 w612] -> w594
              tunnel: w603 -> [w611 _]
              tunnel: w592 -> [_ w612]
              frame False {
                # "Manual Set-point"
              }
              frame True {
              }
            }
            n148 = Select(t=4, s=w609, f=3) -> (s? t:f=w610:i32)
            n149 = call "Furnace SP calc.vi"("SP"=sgl 1000.0) -> ("SP&CRC"=w595:u8[])  [unwired: 10 in]
          }
          frame 1 {
            w633 = u16 0
            # "1Hz MFC's\n\n0. CO2\n1. N2\n2. SO2\n3. H2O\n4. N2P"
            # "Need to Review for new injection"
            # "Need to Review for new injection"
            # "HC Light-Off"
            n150 = call "Mov_Avg_JS.vi"("Array In"=w629, "Cycle Length"=60.0, "Input"=w624) -> ("Array Out Main"=w628:dbl[], "Mean"=w619:dbl)  [unwired: 7 in]
            n151 = Greater Or Equal?(x=w625, y=w634) -> (x >= y?=w635:bool)
            n152 = case shown="True" w627 {
              tunnel: [w637 w638] -> w620
              tunnel: w626 -> [w637 _]
              tunnel: w618 -> [_ w638]
              frame False {
                # "Manual Set-point"
              }
              frame True {
              }
            }
            n153 = Select(t=4, s=w635, f=3) -> (s? t:f=w636:i32)
            n154 = call "Furnace SP calc.vi"("SP"=sgl 1000.0) -> ("SP&CRC"=w621:u8[])  [unwired: 10 in]
          }
          frame 2 {
            w672 = 0 ("t")
            # "NO Light-Off"
            n155 = Multiply(x=w665, y=60.0) -> (x*y=w666:dbl)
            n156 = Divide(x=w666, y=1.2) -> (x/y=w664:dbl)
            n157 = Greater Or Equal?(x=w648, y=w669) -> (x >= y?=w671:bool)
            n158 = call "NOSO2 calc age.vi"("Flow Rate"=w664, "NO/SO2 m ppm"=w654, "NO/SO2 Conc"=w660, "NO/SO2 t ppm"=w661) -> ("NO/SO2 MFR"=w656:dbl)  [unwired: 7 in]
            n159 = call "Mov_Avg_JS.vi"("Array In"=w653, "Input"=w649) -> ("Array Out Main"=w652:dbl[], "Mean"=w644:dbl)  [unwired: 8 in]
            n160 = call "CO calc loff.vi"("CO conc"=w658, "NO conc"=w660, "NO:CO ratio"=w659, "NOx MFR"=w656) -> ()  [unwired: 7 in, 1 out]
            n161 = case shown="False" w651 {
              tunnel: [w673 w674] -> w647
              tunnel: w650 -> [w673 _]
              tunnel: w645 -> [_ w674]
              frame False {
                # "Manual Set-point"
              }
              frame True {
              }
            }
            n162 = Select(t=4, s=w671, f=3) -> (s? t:f=w670:i32)
            n163 = call "Furnace SP calc.vi"("SP"=sgl 1000.0) -> ("SP&CRC"=w646:u8[])  [unwired: 10 in]
          }
          frame 3 {
            w713 = 0
            # "Full System"
            # "1Hz MFC's\n\n0. CO2\n1. N2\n2. SO2\n3. H2O\n4. N2P"
            # "last value of the fan"
            # "Original\n0. CO - x\n1. HC - x\n2. Air - x\n3. NO - x\n4. CO2 \n5. N2\n6. SO2\n7. H2O\n8. AirB - x"
            # "OSC Test"
            n164 = call "Mov_Avg_JS_Dual.vi"("Cycle Length"=w689, "Array In 2"=w696, "Array In"=w697, "Input"=w686) -> ("Array Out Main 2"=w693:dbl[], "Array Out Main"=w694:dbl[], "Mean"=w695:dbl)  [unwired: 4 in, 1 out]
            n165 = call "Mov_Avg_JS.vi"("Array In"=w691, "Cycle Length"=60.0, "Input"=w692) -> ("Array Out Main"=w690:dbl[], "Mean"=w681:dbl)  [unwired: 7 in]
            n166 = Multiply(x=w689, y=10.0) -> (x*y=w688:dbl)
            n167 = case shown="False" w706 {
              tunnel: [w722 w733] -> w701
              tunnel: [w721 w734] -> w702
              tunnel: w705 -> [w720 w734]
              tunnel: w704 -> [w719 _]
              tunnel: w695 -> [w718 _]
              tunnel: w703 -> [w717 _]
              tunnel: w699 -> [w714 w733]
              tunnel: w688 -> [w716 _]
              frame False {
                # "Closed Loop"
                n168 = case shown="False" TRUE {
                  tunnel: [w723 w732] -> w722
                  tunnel: [w724 w731] -> w721
                  tunnel: w720 -> [w724 w730]
                  tunnel: w719 -> [_ w729]
                  tunnel: w714 -> [w723 w728]
                  tunnel: w718 -> [_ w727]
                  tunnel: w717 -> [_ w726]
                  tunnel: w716 -> [_ w725]
                  frame False {
                    # "Furnace PID"
                  }
                  frame True {
                    # "Furnace VI"
                    n169 = call "Furnace_Control_2.vi"("T Furnace"=w726, "Counter Interval"=w725, "T Cat"=w727, "T Set-Point"=w728, "Furnace Set-point"=w729, "Counter In"=w730) -> ("Furnace Set-point"=w732:dbl, "Counter Out"=w731:i32)  [unwired: 4 in]
                  }
                }
              }
              frame True {
                # "Furnace Manual Mode"
              }
            }
            n170 = case shown="False" w698 {
              tunnel: [w735 w736] -> w685
              tunnel: w708 -> [_ _]
              tunnel: w707 -> [_ _]
              tunnel: w700 -> [w735 _]
              tunnel: w682 -> [_ w736]
              frame False {
                # "Manual Set-point"
              }
              frame True {
              }
            }
            n171 = call "Furnace SP calc.vi"("SP"=w701) -> ("SP&CRC"=w684:u8[])  [unwired: 10 in]
            n172 = local read "OSC Stop"() -> (w683:bool)
            n173 = Select(t=4 ("s? t:f"), s=w683, f=3 ("s? t:f")) -> (s? t:f=w710:i32)
          }
          frame 4 {
            w841 = 5.0 ("Multiple")
            w912 = 0
            # "last value of the fan"
            # "NO"
            # "Ageing Test"
            n174 = local read "Fan Speed Recipe"() -> (w751:bool)
            n175 = case shown="True" w751 {
              tunnel: w750 -> [w913 _]
              tunnel: [w913 w914] -> w749
              frame False {
              }
              frame True {
                n176 = local read "Fan Factor Speed"() -> (w914:dbl)
              }
            }
            n177 = call "60pt Mov Avg.vi"("Value in"=w883) -> ("Value out"=→"Uego Avg Fur":dbl)  [unwired: 10 in]
            n178 = Multiply(x=5.0, y=w747) -> (x*y=w877:dbl)
            n179 = call "Mov_Avg_JS_Dual.vi"("Cycle Length"=w877, "Array In 2"=w893, "Input 2"=w839, "Array In"=w894, "Input"=w887) -> ("Array Out Main 2"=w840:dbl[], "Array Out Main"=w842:dbl[])  [unwired: 3 in, 2 out]
            n180 = case shown="True" "Pressure" {
              tunnel: w895 -> [_ w968]
              tunnel: [FALSE w967] -> w859
              frame False {
              }
              frame True {
                # "Press Alarm"
                n181 = Greater?(x=w968, y="Press Up") -> (0:w969:bool)
                n182 = Less?(x=w968, y="Press Low") -> (x < y?=w970:bool)
                n183 = Or(x=w969, y=w970) -> (x .or. y?=w967:bool)
              }
            }
            n184 = call "Mov_Avg_JS.vi"("Array In"=w891, "Cycle Length"=w747, "Input"=w892) -> ("Array Out Main"=w890:dbl[], "Mean"=w878:dbl)  [unwired: 7 in]
            "Flow Avg" <- w878
            n185 = case shown="True" "Flow" {
              tunnel: w878 -> [_ w961]
              tunnel: [FALSE w960] -> w858
              frame False {
              }
              frame True {
                # "Flow Alarm"
                n186 = Greater?(x=w961, y="Flow Up") -> (0:w965:bool)
                n187 = Less?(x=w961, y="Flow Low") -> (x < y?=w964:bool)
                n188 = Or(x=w965, y=w964) -> (x .or. y?=w960:bool)
              }
            }
            n189 = call "Ref_Temp_Calc.vi"("Temp Array"=w842) -> ("T Ref"=w875:dbl)  [unwired: 10 in]
            "T Ref" <- w875
            n190 = call "Stoic_Mean_Calc.vi"("Cycle Length"=w747, "Multiple"=w841, "Array In"=w842) -> ("Max"=w862:dbl, "Mean"=w861:dbl)  [unwired: 1 in, 6 out]
            "T Stoic" <- w861
            "T Max" <- w862
            n191 = call "Alarm_Limit.vi"("Alarm On"="TRef", "Yellow Limit"=7.0, "Red Limit"=12.0, "Target"="TRef Target", "Reading"=w875) -> ("Alarm Output"=w802:bool[])  [unwired: 6 in]
            n192 = Subtract(x=w862, y=w861) -> (x-y=w819:dbl)
            "T Spike" <- w819
            n193 = call "Alarm_Limit.vi"("Alarm On"="TStoic", "Yellow Limit"=7.0, "Red Limit"=12.0, "Target"="TStoic Target", "Reading"=w861) -> ("Alarm Output"=w856:bool[])  [unwired: 6 in]
            n194 = call "Alarm_Limit.vi"("Alarm On"="TSpike", "Yellow Limit"=7.0, "Red Limit"=12.0, "Target"="TSpike Target", "Reading"=w819) -> ("Alarm Output"=w855:bool[])  [unwired: 6 in]
            n195 = Unbundle(w838) -> ("UserChanges"=w837:string[][], "AutoChanges"=w836:string[][], "Stoich Array"=w835:dbl[], "Furnace Set-point"=w834:dbl, "It Out"=w833:i32)
            n196 = local read "Omicron"() -> (w755:bool)
            n197 = case shown="True" w880 {
              tunnel: [w1028 w1029] -> w885
              tunnel: w908 -> [_ _]
              tunnel: w907 -> [_ _]
              tunnel: w749 -> [w1028 _]
              tunnel: w879 -> [_ w1029]
              frame False {
                # "Manual Set-point"
              }
              frame True {
              }
            }
            n198 = local read "Omicron"() -> (w780:bool)
            n199 = Index Array(array=w856, index #1=0 ("index"), index #2=1 ("index")) -> (element #1=w759:bool, element #2=w760:bool)
            "Tstoic 1 Y" <- w760
            "Tstoic 1 R" <- w759
            n200 = Index Array(array=w802, index #1=0 ("index"), index #2=1 ("index")) -> (element #1=w794:bool, element #2=w791:bool)
            "Tref 1 Y" <- w791
            "Tref 1 R" <- w794
            n201 = local read "Omicron"() -> (w800:bool)
            n202 = Index Array(array=w855, index #1=0 ("index"), index #2=1 ("index")) -> (element #1=w771:bool, element #2=w774:bool)
            "Tspike 1 Y" <- w774
            "Tspike 1 R" <- w771
            n203 = case shown="False" w901 {
              tunnel: [w980 w1017] -> w831
              tunnel: [w990 w1021] -> w897
              tunnel: w900 -> [w989 w1021]
              tunnel: w899 -> [w988 _]
              tunnel: w898 -> [_ _]
              tunnel: w896 -> [w985 w1017]
              tunnel: w861 -> [w986 _]
              tunnel: w837 -> [w977 w1020]
              tunnel: w836 -> [w976 w1019]
              tunnel: w835 -> [w975 w1018]
              tunnel: w834 -> [w974 _]
              tunnel: w833 -> [w973 w1016]
              tunnel: [w983 w1020] -> w826
              tunnel: [w982 w1019] -> w827
              tunnel: [w981 w1018] -> w832
              tunnel: [w979 w1017] -> w829
              tunnel: [w978 w1016] -> w828
              frame False {
                n204 = case shown="True" "Stoic Control" {
                  tunnel: [w997 w1013] -> w980
                  tunnel: [w998 w1015] -> w990
                  tunnel: w989 -> [w998 w1015]
                  tunnel: w988 -> [_ w1004]
                  tunnel: w985 -> [w997 w1001]
                  tunnel: w986 -> [_ w1003]
                  tunnel: [FALSE w1014] -> w984
                  tunnel: [w995 w1012] -> w983
                  tunnel: [w994 w1011] -> w982
                  tunnel: [w992 w1010] -> w979
                  tunnel: [w993 w1009] -> w981
                  tunnel: [w991 w1008] -> w978
                  tunnel: w977 -> [w995 w1007]
                  tunnel: w976 -> [w994 w1006]
                  tunnel: w975 -> [w993 w1002]
                  tunnel: w974 -> [w992 w1000]
                  tunnel: w973 -> [w991 w999]
                  frame False {
                    # "Manual Mode"
                  }
                  frame True {
                    # "Furnace VI"
                    n205 = call "FurnaceControl_ME.vi"("StoichTemp"=w1003, "Stoich Array"=w1002, "Target Temp"="Target Tstoic", "Furnace Setpoint"=w1004, "Previous Setpoint"=w1000, "User Setpoint"=w1001, "Auto Change"=w1006, "Countdown"=w999, "User Change"=w1007) -> ("UserChanges"=w1012:string[][], "AutoChanges"=w1011:string[][], "Furnace Setpoint"=w1013:dbl, "User Setpoint"=w1010:dbl, "Stoich Array"=w1009:dbl[], "countdown"=w1008:i32, "Limit Exceeded"=w1014:bool)  [unwired: 4 in]
                  }
                }
                "Furnace SP" <- w980
                "Exceeded" <- w984
              }
              frame True {
                # "Furnace Manual Mode"
              }
            }
            "UserChanges" <- w826
            "AutoChanges" <- w827
            n206 = Decrement(x=w906) -> (x-1=w905:dbl)
            n207 = And(x=w780, y="TSpike") -> (x .and. y?=w778:bool)
            n208 = And(x=w800, y="TRef") -> (x .and. y?=w801:bool)
            n209 = call "Ref_Temp_Calc.vi"("Temp Array"=w840) -> ("T Ref"=w806:dbl)  [unwired: 10 in]
            "T Ref 2" <- w806
            n210 = And(x=w755, y="TStoic") -> (x .and. y?=w754:bool)
            n211 = call "Stoic_Mean_Calc.vi"("Cycle Length"=w747, "Multiple"=w841, "Array In"=w840) -> ("Max"=w843:dbl, "Mean"=w752:dbl)  [unwired: 1 in, 6 out]
            "T Stoic 2" <- w752
            "T Max 2" <- w843
            n212 = Subtract(x=w843, y=w752) -> (x-y=w776:dbl)
            "T Spike 2" <- w776
            n213 = call "Alarm_Limit.vi"("Alarm On"=w754, "Yellow Limit"=7.0, "Red Limit"=12.0, "Target"="TStoic Target", "Reading"=w752) -> ("Alarm Output"=w765:bool[])  [unwired: 6 in]
            n214 = call "Alarm_Limit.vi"("Alarm On"=w801, "Yellow Limit"=7.0, "Red Limit"=12.0, "Target"="TRef Target", "Reading"=w806) -> ("Alarm Output"=w798:bool[])  [unwired: 6 in]
            n215 = call "Alarm_Limit.vi"("Alarm On"=w778, "Yellow Limit"=7.0, "Red Limit"=12.0, "Target"="TSpike Target", "Reading"=w776) -> ("Alarm Output"=w783:bool[])  [unwired: 6 in]
            n216 = Index Array(array=w783, index #1=0 ("index"), index #2=1 ("index")) -> (element #1=w772:bool, element #2=w773:bool)
            "Tspike 2 Y" <- w773
            "Tspike 2 R" <- w772
            n217 = Index Array(array=w765, index #1=0 ("index"), index #2=1 ("index")) -> (element #1=w762:bool, element #2=w761:bool)
            "Tstoic 2 Y" <- w761
            "Tstoic 2 R" <- w762
            n218 = Index Array(array=w798, index #1=0 ("index"), index #2=1 ("index")) -> (element #1=w793:bool, element #2=w792:bool)
            "Tref 2 Y" <- w792
            "Tref 2 R" <- w793
            n219 = call "selectable tc alarm.vi"("Red Limit"="Red Limit", "Linearized Temperature"=w737, "T ref"="T ref", "Array Out Main in"=w742, "Tc Alarm"="Tc Alarm", "Target"="Target Temperature", "Yellow Limit"="Yellow Limit", "Numeric"=w747) -> ("Alarm Output"=w748:bool[], "Tref"=→"Selectable Tc Tref":dbl, "MA"=→"Selectable Tc MA":dbl, "Array Out Main out"=w741:dbl[])
            n220 = Or(x=w792, y=w791) -> (x .or. y?=w788:bool)
            n221 = Or(x=w773, y=w774) -> (x .or. y?=w770:bool)
            n222 = Or(x=w762, y=w759) -> (x .or. y?=w757:bool)
            n223 = Or(x=w793, y=w794) -> (x .or. y?=w790:bool)
            n224 = Or(x=w761, y=w760) -> (x .or. y?=w758:bool)
            n225 = Or(x=w772, y=w771) -> (x .or. y?=w769:bool)
            n226 = local read "HC Cyc Add Factor"() -> (w810:dbl)
            n227 = local read "Lambda Avg"() -> (w869:dbl)
            n228 = case shown="False" w790 {
              selector: w790 -> [w929 w931]
              tunnel: [w927 w930] -> w789
              tunnel: w788 -> [w928 _]
              frame False {
                n229 = Build Array(w929, w928) -> (w927:bool[])
              }
              frame True {
                n230 = Build Array(w931, FALSE) -> (w930:bool[])
              }
            }
            n231 = case shown="False" w757 {
              selector: w757 -> [w923 w925]
              tunnel: [w921 w924] -> w785
              tunnel: w758 -> [w922 _]
              frame False {
                n232 = Build Array(w923, w922) -> (w921:bool[])
              }
              frame True {
                n233 = Build Array(w925, FALSE) -> (w924:bool[])
              }
            }
            n234 = case shown="False" w769 {
              selector: w769 -> [w917 w919]
              tunnel: [w915 w918] -> w786
              tunnel: w770 -> [w916 _]
              frame False {
                n235 = Build Array(w917, w916) -> (w915:bool[])
              }
              frame True {
                n236 = Build Array(w919, FALSE) -> (w918:bool[])
              }
            }
            n237 = Unbundle(w813) -> ("UserChanges"=w818:string[][], "AutoChanges"=w817:string[][], "Spike Array"=w816:dbl[], "Furnace Set-point"=w815:dbl, "It Out"=w814:i32)
            n238 = case shown="False" w882 {
              tunnel: w905 -> [w1023 w1027]
              tunnel: [w1022 w1024] -> w904
              tunnel: [w1023 w1027] -> w903
              tunnel: w902 -> [_ w1025]
              tunnel: w888 -> [_ w1026]
              frame False {
                n239 = Less Or Equal To 0?(x=w1023) -> (x <= 0?=w1022:bool)
              }
              frame True {
                n240 = Greater Or Equal?(x=w1026, y=w1025) -> (x >= y?=w1024:bool)
              }
            }
            n241 = case shown="True" "Spike Control" {
              tunnel: [w939 w955] -> w808
              tunnel: [w938 w954] -> w809
              tunnel: [w937 w953] -> w823
              tunnel: [FALSE w952] -> w824
              tunnel: [w935 w951] -> w821
              tunnel: [w936 w941] -> w822
              tunnel: w818 -> [w939 w950]
              tunnel: w817 -> [w938 w949]
              tunnel: w819 -> [_ w948]
              tunnel: w816 -> [w937 w947]
              tunnel: w815 -> [w936 w945]
              tunnel: w814 -> [w935 w944]
              tunnel: [w934 w940] -> w812
              tunnel: w811 -> [_ w943]
              tunnel: w810 -> [w934 w942]
              frame False {
              }
              frame True {
                n242 = call "SpikeControl_ME.vi"("Temp Spike"=w948, "Spike Array"=w947, "Target Spike"="Target Tspike", "HC Add"=w943, "Previous HC Add"=w945, "User HC Add"=w942, "Auto Change"=w949, "Countdown"=w944, "User Change"=w950) -> ("UserChanges"=w955:string[][], "AutoChanges"=w954:string[][], "HC Add"=w940:dbl, "User HC Add"=w941:dbl, "Spike Array"=w953:dbl[], "countdown"=w951:i32, "Limit Exceeded"=w952:bool)  [unwired: 4 in]
                "HC Add" <- w940
              }
            }
            "Exceeded 2" <- w824
            "UserChanges Spike" <- w808
            "AutoChanges Spike" <- w809
            n243 = call "Alarm_Limit.vi"("Alarm On"="Lambda", "Yellow Limit"=0.03 ("Red Limit"), "Red Limit"=0.07, "Target"="Lambda \nTarget", "Reading"=w869) -> ("Alarm Output"=w860:bool[])  [unwired: 6 in]
            "Alarm Output 2" <- w860
            n244 = Index Array(array=w860, index=0) -> (element=w854:bool)
            n245 = Build Array(w790, w757, w769, w854) -> (w851:bool[])
            n246 = Boolean Array To Number(Boolean array=w851) -> (number=w853:u32)
            n247 = Equal To 0?(x=w853) -> (x = 0?=w852:bool)
            n248 = Less Or Equal To 0?(x=w849) -> (x <= 0?=w848:bool)
            n249 = case shown="True" w852 {
              tunnel: [w957 u32 30 ("number")] -> w850
              tunnel: w849 -> [w956 _]
              frame False {
                n250 = Decrement(x=w956) -> (x-1=w957:u32)
              }
              frame True {
              }
            }
            n251 = call "Furnace SP calc.vi"("SP"=w831) -> ("SP&CRC"=w884:u8[])  [unwired: 10 in]
            n252 = Bundle("UserChanges"=w826, "AutoChanges"=w827, "Stoich Array"=w832, "Furnace SP"=w829, "It Out"=w828) -> (w830:T12)  [unwired: 1 in]
            n253 = Build Array (concatenate)(w789, w785, w786, w860, w859, w748, w858, w848) -> (w857:bool[])
            n254 = Select(t=4 ("s? t:f"), s=w904, f=3 ("s? t:f")) -> (s? t:f=w909:i32)
            n255 = Bundle("UserChanges"=w808, "AutoChanges"=w809, "Spike Array"=w823, "User HC Add"=w822, "countdown"=w821) -> (w820:T13)  [unwired: 1 in]
            n256 = Boolean Array To Number(Boolean array=w857) -> (number=w889:u32)
          }
        }
      }
      frame 4 {
        w1035 = 0.0 ("Set-point Fan")
        w1039 = 0.0 ("Sw time")
        w1038 = FALSE
        w1053 = 0
        # "Shutdown/cooldown"
        # "follow condition \nthen go to standby"
        n257 = Decrement(x=w1041) -> (x-1=w1040:dbl)
        n258 = Less Or Equal?(x=w1040, y=0.0) -> (x <= y?=w1048:bool)
        n259 = Select(t=5, s=w1048, f=4) -> (s? t:f=w1054:i32)
        n260 = local write "TankHi"(0.5 ("TankHi")) -> ()
        n261 = local write "TankLo"(0.0 ("TankHi")) -> ()
        n262 = call "Furnace SP calc.vi"("SP"=sgl 10.0) -> ("SP&CRC"=w1036:u8[])  [unwired: 10 in]
      }
      frame 5 {
        w1060 = 0.0 ("Set-point Fan")
        w1063 = 0.0 ("Sw time")
        w1062 = FALSE
        w1066 = FALSE ("DO On?")
        w1072 = u16 0 ("length")
        # "Off"
        n263 = xnode "Read/Write Control"("FPGA VI Reference In"=w1073, "Command"=2, "DO On?"=w1066, "Leak test on?"=w1066) -> ()  [unwired: 1 in, 2 out]
        n264 = shared-variable "RT CompactRIO Target\\Library 1.lvlib\\Enum 1"(u16 0 ("Enum 1")) -> ()  [unwired: 1 in, 1 out]
      }
    }
    n265 = Build Array (concatenate)("Ageing Metric\nControl", w166, w165) -> (w163:dbl[])
    n266 = Index Array(array=w166, index #1=1 ("index"), index #2=2 ("index"), index #3=w211, index #4=w211) -> (element #1=→"Ageing Time":dbl, element #2=→"Remaining Time":dbl, element #3=→"Complete":dbl, element #4=→"% Complete":dbl)
    n267 = Index Array(array=w165, index #1=1 ("index"), index #2=2 ("index"), index #3=w210, index #4=w210) -> (element #1=→"Ageing Time 2":dbl, element #2=→"Remaining Time 2":dbl, element #3=→"Complete 2":dbl, element #4=→"% Complete 2":dbl)
    n268 = local read "Time Step"() -> (w168:i32)
    n269 = Divide(x=w168, y=10) -> (x/y=w164:dbl)
    n270 = local read "Valve 1"() -> (w64:dbl)
    n271 = local read "Valve 2"() -> (w63:dbl)
    n272 = local read "Valve 3"() -> (w62:dbl)
    n273 = local read "Valve 4"() -> (w61:dbl)
    n274 = call "Energy_Estimation.vi"("Energy Total"=w84, "Signal Out"=w85) -> ("Energy Out"=w83:dbl)  [unwired: 9 in]
    n275 = xnode "Read/Write Control"("FPGA VI Reference In"=w191, "Furnace Array Out"=w280) -> ("FPGA VI Reference Out"=w279:refnum<k20>, "error out"=w278:errorcluster)  [unwired: 1 in]
    n276 = xnode "Read/Write Control"("FPGA VI Reference In"=w275, "Fan Voltage Out"=w183, "Extract Fan Out"="Extract Fan V", "Heat Exch Fan"="Heat Exch Fan V", "Furnace Power"=w85) -> ()  [unwired: 1 in, 2 out]
    n277 = Build Array (concatenate)(w333, w316, w274, 0 ("index"), w164, w163, w162, w82, w83, w64, w63, w62, w61) -> (w338:dbl[])
    n278 = shared-variable "RT CompactRIO Target\\Library 1.lvlib\\DATA"(w338) -> ()  [unwired: 1 in, 1 out]
    n279 = node-c288() -> ()  [unwired: 1 in, 1 out]
    "Test Start" <- w71
  }
  n280 = timed-loop {
    timing: w28 -> [_]
    timing-out: [_] -> w27
    tunnel: w24 -> [w1086]
    stop <- w1074 stop-if-true
    # "NEW Uego Sub Vi"
    n281 = node-c288() -> ()  [unwired: 1 in, 1 out]
    n282 = xnode "Read/Write Control"("FPGA VI Reference In"=w1086) -> ("FPGA VI Reference Out"=w1077:refnum<k20>, "O2Data"=w1078:T15)  [unwired: 1 in, 1 out]
    n283 = call <vilib>:"uego_rt_reve.vi"("UEGOModuleEnable"="UEGOModuleEnable", "UEGOCalibration"=T14 {"Stoich A/F Ratio"=14.7, "IpArray (mA)"=[-2.0, -1.9, -1.8, -1.7, -1.602, -1.5, -1.4, -1.3, -1.243, -1.1, -1.0, -0.927, -0.8, -0.7, -0.652, -0.5, -0.405, -0.183, -0.0746, -0.0398, -0.007, 0.0, 0.0146, 0.057, 0.097, 0.15, 0.193, 0.25, 0.329, 0.35, 0.4, 0.45, 0.509, 0.55, 0.6, 0.67, 0.7, 0.75, 0.8, 0.85, 0.9, 0.938, 1.0, 1.05, 1.1, 1.15, 1.2, 1.25, 1.3, 1.35, 1.4, 1.45, 1.5, 1.55, 1.6, 1.65, 1.7, 1.75, 1.8, 1.85, 1.9, 1.95, 2.0, 2.05, 2.1, 2.15, 2.2, 2.25, 2.3, 2.3565], "LambdaArray"=[0.65, 0.6607, 0.6732, 0.6866, 0.7, 0.714, 0.7278, 0.7418, 0.75, 0.7716, 0.7876, 0.7999, 0.8224, 0.841, 0.8502, 0.8802, 0.8999, 0.9501, 0.9791, 0.9895, 1.0, 1.0032, 1.01, 1.0301, 1.0498, 1.077, 1.1, 1.1319, 1.179, 1.1921, 1.2243, 1.2581, 1.3002, 1.331, 1.3703, 1.4289, 1.4554, 1.5016, 1.5504, 1.6021, 1.657, 1.701, 1.7774, 1.8437, 1.9145, 1.9904, 2.0719, 2.1597, 2.2545, 2.3571, 2.4687, 2.5904, 2.7236, 2.8701, 3.0321, 3.212, 3.4131, 3.6393, 3.8958, 4.189, 4.5275, 4.9229, 5.3907, 5.9531, 6.6421, 7.5061, 8.6219, 10.1187, 12.2328, 15.99]}, "UEGO Back Pressure (bar)"="UEGO Back Pressure (bar)", "UEGOData (From FPGA)"=w1078, "SensorControl"="SensorControl") -> ("UEGO Diagnostics"=→"UEGO Diagnostics":T6, "UEGO Sensor Results"=→"UEGO Sensor Results":T2, "UEGO Heater (V)"=→"UEGO Heater (V)":T5, "UEGO Temperature (C)"=→"UEGO Temperature (C)":T7, "UEGOControl (To FPGA)"=w1079:T16)  [unwired: 1 out]
    n284 = local read "STOP"() -> (w1074:bool)
    n285 = xnode "Read/Write Control"("FPGA VI Reference In"=w1077, "O2Control"=w1079) -> ()  [unwired: 1 in, 2 out]
    n286 = node-c288() -> ()  [unwired: 1 in, 1 out]
  }
  n287 = timed-loop {
    timing: w44 -> [_]
    timing-out: [_] -> w43
    shift-right: [w1289] -> _
    shift-left: 0 ("t") -> [w1290]
    tunnel: w42 -> [w1212]
    tunnel: w37 -> [w1259]
    shift-right: [w1280] -> _
    shift-left: i32[] [0, 0, 3, 1, 1, 1, 1, 0] -> [w1281]
    tunnel: w37 -> [w1178]
    tunnel: w24 -> [w1242]
    tunnel: w33 -> [w1241]
    shift-right: [w1222] -> _
    shift-left: _ -> [w1223]
    shift-right: [w1208] -> _
    shift-left: w18 -> [w1205]
    shift-right: [w1207] -> _
    shift-left: w14 -> [w1206]
    shift-right: [w1170] -> _
    shift-left: w22 -> [w1173]
    shift-right: [w1171] -> _
    shift-left: w22 -> [w1172]
    shift-right: [w1168] -> _
    shift-left: w21 -> [w1169]
    shift-right: [w1164] -> _
    shift-left: w18 -> [w1166]
    shift-right: [w1163] -> _
    shift-left: w18 -> [w1165]
    shift-right: [w1161] -> _
    shift-left: w22 -> [w1162]
    shift-right: [w1111] -> _
    shift-left: dbl[] [0.0, 0.0, 0.0, 0.0, 0.0, 0.0, 0.0, 0.0, 0.0, 0.0, 0.0, 0.0, 0.0, 0.0, 0.0, 0.0, 0.0, 0.0, 0.0, 0.0, 0.0, 0.0, 0.0, 0.0, 0.0, 0.0, 0.0, 0.0, 0.0, 0.0, 0.0, 0.0, 0.0, 0.0, 0.0, 0.0, 0.0, 0.0, 0.0, 0.0, 0.0, 0.0, 0.0, 0.0, 0.0, 0.0, 0.0, 0.0, 0.0, 0.0, 0.0, 0.0, 0.0, 0.0, 0.0, 0.0, 0.0, 0.0, 0.0, 0.0, 0.0, 0.0, 0.0, 0.0, 0.0] ("Array of Double") -> [w1160]
    shift-right: [w1158] -> _
    shift-left: w21 -> [w1157]
    shift-right: [w1127] -> _
    shift-left: 1 ("index") -> [w1126]
    shift-right: [w1120] -> _
    shift-left: w18 -> [w1118]
    shift-right: [w1119] -> _
    shift-left: w18 -> [w1117]
    shift-right: [w1116] -> _
    shift-left: w18 -> [w1114]
    shift-right: [w1115] -> _
    shift-left: w18 -> [w1113]
    shift-right: [w1109] -> _
    shift-left: w14 -> [w1098]
    stop <- w1110 stop-if-true
    # "Cat 2"
    # "Cat 1"
    # "MFC Error Display"
    # "10 Hz MFC's\n0. CO\n1. HC_1\n2. Air_1\n3. NO\n4. Air_B\n5. HC_B\n6. Air_2\n7. HC_2"
    # "MFC's\n00. CO\n01. HC _1\n02. Air_1\n03. NO\n04. CO2\n05. N2\n06. SO2\n07. H2O\n08. Air_B\n09.HC_B\n10. Air_2\n11. N2P\n12. HC_2"
    n288 = node-c288() -> (→"Iteration \nDuration 3":i64)  [unwired: 1 in, 2 out]
    n289 = xnode "Read/Write Control"("FPGA VI Reference In"=w1242, "error in"=w1241) -> ("Expansion Input Array"=w1192:fxp<+/-,34,9>[])  [unwired: 2 out]
    n290 = local read "UEGO Sensor Results"() -> (w1220:T2)
    n291 = shared-variable "RT CompactRIO Target\\Library 1.lvlib\\Control Variables"(error in=w1212) -> (w1105:dbl[])  [unwired: 1 out]
    "Control Variables" <- w1105
    n292 = shared-variable "RT CompactRIO Target\\Library 1.lvlib\\Analyser_Data"(error in=w1212) -> (w1211:dbl[])  [unwired: 1 out]
    n293 = xnode "Read/Write Control"("FPGA VI Reference In"=w1259, "error in"=w1212) -> ("MFC Array In"=w1239:fxp<+/-,30,9>[], "Valve Array In"=w1193:fxp<+/-,30,9>[])  [unwired: 2 out]
    n294 = xnode "Read/Write Control"("FPGA VI Reference In"=w1178, "error in"=w1212) -> ("Array 1 In"=w1266:fxp<+/-,35,9>[])  [unwired: 2 out]
    n295 = xnode "Read/Write Control"("FPGA VI Reference In"=w1178, "error in"=w1212) -> ("MFC Error No."=w1112:u16)  [unwired: 2 out]
    n296 = Index Array(array=w1105, index=50) -> (element=w1106:dbl)
    n297 = Number To Boolean Array(number=w1106) -> (Boolean array=w1107:bool[])
    n298 = Delete From Array(array=w1266, length=4, index=1) -> (deleted portion=w1263:fxp<+/-,35,9>[])  [unwired: 1 out]
    n299 = shared-variable "RT CompactRIO Target\\Library 1.lvlib\\Inject_Arrays_System"(error in=w1212) -> (w1260:dbl[])  [unwired: 1 out]
    n300 = Unbundle By Name(w1220) -> ("UEGO1Lambda"=w1219:sgl, "UEGO2Lambda"=w1203:sgl)
    n301 = Number To Boolean Array(number=w1112) -> (Boolean array=w1243:bool[])
    n302 = Index Array(array=w1107, index=2) -> (element=w1090:bool)
    "Omicron" <- w1090
    n303 = Index Array(array=w1263) -> (element #1=w1180:fxp<+/-,35,9>, element #2=w1181:fxp<+/-,35,9>, element #3=w1182:fxp<+/-,35,9>, element #4=w1183:fxp<+/-,35,9>)  [unwired: 4 in]
    n304 = Index Array(array=w1243) -> (element #1=→"CO":bool, element #2=→"HC":bool, element #3=→"Air":bool, element #4=→"NO":bool, element #5=→"N2":bool, element #6=→"Air-B":bool, element #7=→"HC-B":bool, element #8=→"Air-2":bool, element #9=→"N2-2":bool, element #10=→"HC-2":bool, element #11=→"O2":bool)  [unwired: 11 in]
    n305 = Delete From Array(array=w1239, length=1, index=0) -> (array with subset deleted=w1236:fxp<+/-,30,9>[])  [unwired: 1 out]
    n306 = Delete From Array(array=w1193, length=1, index=0) -> (array with subset deleted=w1125:fxp<+/-,30,9>[])  [unwired: 1 out]
    n307 = call "ECM_Lambda_Propane.vi"("V In"=w1182) -> ("Lambda Corr"=w1175:dbl)  [unwired: 6 in, 2 out]
    n308 = call "ECM_Lambda_Propane.vi"("V In"=w1183) -> ("Lambda Corr"=w1218:dbl)  [unwired: 6 in, 2 out]
    n309 = call "5pt Mov Avg.vi"("Value in"=w1181) -> ("Value out"=w1167:dbl)  [unwired: 10 in]
    n310 = Index Array(array=w1192, index=0) -> (element=w1279:fxp<+/-,34,9>)
    n311 = call "Valve_Read.vi"("In Array"=w1125) -> ("Valve 4"=→"Valve 4":dbl, "Valve 3"=→"Valve 3":dbl, "Valve 2"=→"Valve 2":dbl, "Valve 1"=→"Valve 1":dbl)  [unwired: 5 in]
    n312 = call "MFC Parse.vi"("MFC Raw"=w1236) -> ("Array"=w1159:dbl[])
    n313 = call "5pt Mov Avg.vi"("Value in"=w1219) -> ("Value out"=w1202:dbl)  [unwired: 10 in]
    n314 = call "5pt Mov Avg.vi"("Value in"=w1203) -> ("Value out"=w1209:dbl)  [unwired: 10 in]
    n315 = call "5pt Mov Avg.vi"("Value in"=w1180) -> ("Value out"=w1174:dbl)  [unwired: 10 in]
    n316 = call "5pt Mov Avg.vi"("Value in"=w1279) -> ("Value out"=w1278:dbl)  [unwired: 10 in]
    n317 = Index Array(array=i32[] [1, 28, 24, 25, 26, 18, 19, 20, 29, 30, 2, 6, 7, 8, 14, 15, 16, 17, 13] ("appended array")) -> (element #1=w1151:i32, element #2=w1150:i32, element #3=w1149:i32, element #4=w1148:i32, element #5=w1147:i32, element #6=w1146:i32, element #7=w1145:i32, element #8=w1144:i32, element #9=w1143:i32, element #10=w1142:i32, element #11=w1141:i32, element #12=w1140:i32, element #13=w1139:i32, element #14=w1138:i32, element #15=w1137:i32, element #16=w1136:i32, element #17=w1135:i32, element #18=w1134:i32, element #19=w1128:i32)  [unwired: 19 in]
    n318 = local read "STOP"() -> (w1110:bool)
    n319 = call "5pt Mov Avg.vi"("Value in"=w1278) -> ("Value out"=→"Flow 1":dbl)  [unwired: 10 in]
    n320 = Build Array(w1174, w1167, w1202, w1209) -> (→"UEGO Array":dbl[])
    n321 = Index Array(array=w1105, index #1=w1151, index #2=w1150, index #3=w1149, index #4=w1148, index #5=w1147, index #6=w1146, index #7=w1145, index #8=w1144, index #9=w1143, index #10=w1142, index #11=w1141, index #12=w1140, index #13=w1139, index #14=w1138, index #15=w1137, index #16=w1136, index #17=w1135, index #18=w1134, index #19=w1128) -> (element #1=w1155:dbl, element #2=w1291:dbl, element #3=w1292:dbl, element #4=w1293:dbl, element #5=w1294:dbl, element #6=w1288:dbl, element #7=w1287:dbl, element #8=w1286:dbl, element #9=w1285:dbl, element #10=w1284:dbl, element #11=w1216:dbl, element #12=w1215:dbl, element #13=w1214:dbl, element #14=w1210:dbl, element #15=w1156:dbl, element #16=w1154:dbl, element #17=w1153:dbl, element #18=w1152:dbl, element #19=w1129:dbl)
    n322 = Bundle By Name(cluster=cluster{"output high":dbl, "output low":dbl} {"output high"=100.0, "output low"=-100.0} ("output range"), "output high"="Output High 3", "output low"="Output Low 3") -> (w1252:cluster{"output high":dbl, "output low":dbl})
    n323 = local read "Loop No."() -> (w1240:i32)
    n324 = call "System_Inj_Array_Split.vi"("Inject_Arrays"=w1206, "Omicron"=w1090) -> ("Valve 3"=w1100:dbl[], "Valve 2"=w1099:dbl[], "Valve 1"=w1231:dbl[], "HC Bal"=w1232:dbl[], "Evac 1"=w1102:dbl[], "Air Bal"=w1233:dbl[], "Evac 2"=w1101:dbl[])  [unwired: 2 in, 1 out]
    n325 = call "Inj_Array_Split.vi"("Inject_Arrays"=w1205, "Omicron"=w1090) -> ("Air Add"=w1272:dbl[], "Air Cyc"=w1273:dbl[], "HC Add"=w1274:dbl[], "HC Cyc"=w1275:dbl[], "O2"=w1271:dbl[], "CO"=w1276:dbl[], "NO"=w1277:dbl[], "Cycle Length"=w1204:i32)  [unwired: 2 in]
    "Cycle Length" <- w1204
    n326 = Decrement(x=w1204) -> (x-1=w1267:i32)
    n327 = call "Inj_Array_Split.vi"("Inject_Arrays"=w1098, "Omicron"=w1090) -> ("Air Add"=w1094:dbl[], "Air Cyc"=w1093:dbl[], "HC Add"=w1095:dbl[], "HC Cyc"=w1096:dbl[], "O2"=w1092:dbl[], "CO"=w1097:dbl[])  [unwired: 2 in, 2 out]
    n328 = case shown="3" w1240 {
      tunnel: [w1310 w1326 "Air Cyc 1" w1484 w2074 w2088] -> w1298
      tunnel: [w1310 w1326 "NO" w1483 w2074 w2088] -> w1297
      tunnel: [w1310 w1326 "N2" w1482 50.0 ("Numeric") 0.0 ("Numeric")] -> w1270
      tunnel: [w1310 w1326 "HC Cyc 1" w1481 w2074 w2088] -> w1269
      tunnel: [w1310 w1326 "Air Bal" w1480 w2074 w2088] -> w1296
      tunnel: 0.0 ("y") -> [_ _ _ w1479 _ _]
      tunnel: w1294 -> [_ _ _ w1478 _ _]
      tunnel: w1293 -> [_ _ _ w1477 _ _]
      tunnel: w1292 -> [_ _ _ w1476 _ _]
      tunnel: w1291 -> [_ _ _ w1475 _ _]
      tunnel: w1156 -> [_ _ w1339 w1397 _ _]
      tunnel: w1290 -> [w1315 w1331 _ w1474 _ _]
      tunnel: [w1315 w1331 0 ("t") w1473 0 ("t") 0 ("t")] -> w1289
      tunnel: w1276 -> [_ _ _ w1472 _ _]
      tunnel: w1275 -> [_ _ _ w1471 _ _]
      tunnel: w1274 -> [_ _ _ w1470 _ _]
      tunnel: w1288 -> [_ _ _ w1469 _ _]
      tunnel: w1287 -> [_ _ _ w1468 _ _]
      tunnel: w1286 -> [_ _ _ w1467 _ _]
      tunnel: w1285 -> [_ _ _ w1466 _ _]
      tunnel: w1284 -> [_ _ _ w1465 _ _]
      tunnel: w1277 -> [_ _ _ w1464 _ _]
      tunnel: w1281 -> [_ w1332 _ w1463 _ _]
      tunnel: [i32[] [] w1332 i32[] [0, 0, 3, 1, 1, 1, 1, 0] i32[] [] i32[] [] i32[] []] -> w1280
      tunnel: w1267 -> [_ _ _ w1462 _ _]
      tunnel: w1273 -> [_ _ _ w1461 _ _]
      tunnel: [w1310 w1326 "HC Bal" w1460 w2074 w2088] -> w1268
      tunnel: w1272 -> [_ _ _ w1459 _ _]
      tunnel: w1271 -> [_ _ _ w1458 _ _]
      tunnel: [_ _ _ w1457 _ _] -> w1262
      tunnel: w1175 -> [_ _ _ w1456 _ _]
      tunnel: w1218 -> [_ _ _ w1455 _ _]
      tunnel: [_ _ _ w1447 _ _] -> w1261
      tunnel: w1260 -> [_ _ _ w1454 _ _]
      tunnel: w1204 -> [_ _ _ w1453 _ _]
      tunnel: [w1310 w1326 "Air Cyc 2" w1452 w2074 w2088] -> w1258
      tunnel: [w1310 w1326 "CO" w1451 w2074 w2088] -> w1257
      tunnel: "PID Mop-up Catalyst" -> [_ _ _ w1450 _ _]
      tunnel: w1252 -> [_ _ _ w1449 _ _]
      tunnel: w1178 -> [_ _ _ w1448 _ _]
      tunnel: w1174 -> [_ _ _ w1446 _ _]
      tunnel: w1233 -> [_ _ _ w1445 _ _]
      tunnel: w1232 -> [_ _ _ w1444 _ _]
      tunnel: w1231 -> [_ _ _ w1443 _ _]
      tunnel: "Valve 1 SP" -> [w1314 w1330 w1360 w1442 _ _]
      tunnel: "Valve 2 SP" -> [w1313 w1329 w1359 w1440 _ _]
      tunnel: [w1314 w1330 w1360 w1441 w2073 w2087] -> w1225
      tunnel: [w1313 w1329 w1359 w1439 w2073 w2087] -> w1224
      tunnel: w1223 -> [_ _ _ w1438 _ _]
      tunnel: [_ _ _ w1437 _ _] -> w1222
      tunnel: w1202 -> [_ _ _ w1436 _ _]
      tunnel: w1209 -> [_ _ _ w1435 _ _]
      tunnel: w1216 -> [_ _ _ w1434 _ _]
      tunnel: w1215 -> [_ _ _ w1433 _ _]
      tunnel: w1214 -> [_ _ _ w1432 _ _]
      tunnel: "NO PID Light-Off" -> [_ _ _ w1431 _ _]
      tunnel: w1211 -> [_ _ _ w1430 _ _]
      tunnel: w1210 -> [_ _ _ w1429 _ _]
      tunnel: [dbl[] [] ("Array of Double") w1328 w1357 w1427 w2076 w2090] -> w1208
      tunnel: [dbl[] [] ("Array of Double") w1327 w1358 w1428 w2077 w2091] -> w1207
      tunnel: w1206 -> [_ _ w1358 w1428 w2077 w2091]
      tunnel: w1205 -> [_ _ w1357 w1427 w2076 w2090]
      tunnel: [w1309 w1325 w1349 w1423 w2073 w2087] -> w1199
      tunnel: [w1308 w1324 w1348 w1422 w2073 w2087] -> w1198
      tunnel: [w1310 w1326 "N2 2" w1426 w2074 w2088] -> w1196
      tunnel: [w1310 w1326 "HC Cyc 2" w1425 w2074 w2088] -> w1195
      tunnel: [w1310 w1326 "O2" w1424 w2074 w2088] -> w1194
      tunnel: "Valve 3 SP" -> [w1309 w1325 w1349 w1421 _ _]
      tunnel: "Valve 4 SP" -> [w1308 w1324 w1348 w1420 _ _]
      tunnel: [w1300 w1316 w1335 w1418 w2064 w2078] -> w1177
      tunnel: [w1300 w1316 w1335 w1417 w2064 w2078] -> w1176
      tunnel: w1173 -> [_ _ _ w1413 _ _]
      tunnel: w1172 -> [_ _ _ w1415 _ _]
      tunnel: [w1305 w1322 w1346 w1416 w2069 w2083] -> w1171
      tunnel: [w1305 w1322 w1339 w1414 w2069 w2083] -> w1170
      tunnel: w1169 -> [_ _ _ w1412 _ _]
      tunnel: [0 ("t") 0 ("t") 0 ("t") w1411 0 ("t") 0 ("t")] -> w1168
      tunnel: w1167 -> [_ _ _ w1410 _ _]
      tunnel: w1166 -> [_ _ _ w1409 _ _]
      tunnel: w1165 -> [_ _ _ w1408 _ _]
      tunnel: [w1302 w1319 w1337 w1407 w2066 w2080] -> w1164
      tunnel: [w1302 w1319 w1337 w1406 w2066 w2080] -> w1163
      tunnel: w1162 -> [_ _ _ w1405 _ _]
      tunnel: [w1305 w1322 w1346 w1404 w2069 w2083] -> w1161
      tunnel: w1160 -> [w1304 w1321 w1341 w1403 w2068 w2082]
      tunnel: [w1304 w1321 w1342 w1402 w2068 w2082] -> w1111
      tunnel: w1159 -> [_ _ _ w1401 _ _]
      tunnel: [_ _ _ w1400 _ _] -> w1158
      tunnel: w1157 -> [_ _ _ w1399 _ _]
      tunnel: w1155 -> [_ _ w1344 w1398 _ _]
      tunnel: w1154 -> [_ _ _ w1396 _ _]
      tunnel: w1153 -> [_ _ _ w1395 _ _]
      tunnel: w1152 -> [_ _ _ w1394 _ _]
      tunnel: w1129 -> [_ _ _ w1393 _ _]
      tunnel: [1 ("index") 1 ("index") 1 ("index") w1392 1 ("index") 1 ("index")] -> w1127
      tunnel: w1126 -> [_ _ _ w1391 _ _]
      tunnel: [w1302 w1319 w1337 w1390 w2066 w2080] -> w1120
      tunnel: [w1302 w1319 w1337 w1389 w2066 w2080] -> w1119
      tunnel: w1118 -> [_ _ _ w1388 _ _]
      tunnel: w1117 -> [_ _ _ w1387 _ _]
      tunnel: [w1302 w1319 w1337 w1386 w2066 w2080] -> w1116
      tunnel: [w1302 w1319 w1337 w1385 w2066 w2080] -> w1115
      tunnel: w1114 -> [_ _ _ w1384 _ _]
      tunnel: w1113 -> [_ _ _ w1383 _ _]
      tunnel: [dbl[] [] ("Array of Double") w1318 w1336 w1382 w2065 w2079] -> w1109
      tunnel: w1098 -> [_ _ w1336 w1382 w2065 w2079]
      tunnel: [w1300 w1316 w1335 w1381 w2064 w2078] -> w1104
      tunnel: [w1300 w1316 w1335 w1380 w2064 w2078] -> w1103
      tunnel: w1102 -> [_ _ _ w1379 _ _]
      tunnel: w1101 -> [_ _ _ w1378 _ _]
      tunnel: w1100 -> [_ _ _ w1377 _ _]
      tunnel: w1099 -> [_ _ _ w1376 _ _]
      tunnel: w1090 -> [_ _ _ w1375 _ _]
      tunnel: w1097 -> [_ _ _ w1374 _ _]
      tunnel: w1096 -> [_ _ _ w1373 _ _]
      tunnel: w1095 -> [_ _ _ w1372 _ _]
      tunnel: w1094 -> [_ _ _ w1371 _ _]
      tunnel: w1093 -> [_ _ _ w1370 _ _]
      tunnel: w1092 -> [_ _ _ w1369 _ _]
      frame 0, Default {
        w1302 = dbl[] [] ("Array Out Main")
        w1305 = i16 0
        w1300 = FALSE
        w1310 = 0.0 ("Numeric")
      }
      frame 1 {
        w1319 = dbl[] [] ("Array Out Main")
        w1322 = i16 0
        w1316 = FALSE
        w1326 = 0.0 ("Numeric")
        n329 = local read "Omicron"() -> (w1317:bool)
        n330 = case shown="True" w1317 {
          tunnel: [dbl[] [] ("Array of Double") w1334] -> w1318
          frame False {
          }
          frame True {
            n331 = shared-variable "RT CompactRIO Target\\Library 1.lvlib\\Inject_Arrays_Cat-2"() -> (w1334:dbl[])  [unwired: 1 in, 1 out]
          }
        }
        n332 = shared-variable "RT CompactRIO Target\\Library 1.lvlib\\Inject_Arrays_System"() -> (w1327:dbl[])  [unwired: 1 in, 1 out]
        n333 = shared-variable "RT CompactRIO Target\\Library 1.lvlib\\Inject_Arrays_Cat-1"() -> (w1328:dbl[])  [unwired: 1 in, 1 out]
      }
      frame 2 {
        w1335 = FALSE
        w1337 = dbl[] [] ("Array Out Main")
        w1346 = i16 0
        n334 = Equal?(x=w1344, y=3.0) -> (x = y?=w1340:bool)
        n335 = local write "OSC Stop"(FALSE ("OSC Stop")) -> ()
        n336 = case shown="True" w1340 {
          tunnel: [w1367 dbl[] [0.0, 0.0, 0.0, 0.0, 0.0, 0.0, 0.0, 0.0, 0.0, 0.0, 0.0, 0.0, 0.0, 0.0, 0.0, 0.0, 0.0, 0.0, 0.0, 0.0, 0.0, 0.0, 0.0, 0.0, 0.0, 0.0, 0.0, 0.0, 0.0, 0.0, 0.0, 0.0, 0.0, 0.0, 0.0, 0.0, 0.0, 0.0, 0.0, 0.0, 0.0, 0.0, 0.0, 0.0, 0.0, 0.0, 0.0, 0.0, 0.0, 0.0, 0.0, 0.0, 0.0, 0.0, 0.0, 0.0, 0.0, 0.0, 0.0, 0.0, 0.0, 0.0, 0.0, 0.0, 0.0] ("Array of Double")] -> w1342
          tunnel: w1341 -> [w1367 _]
          frame False {
          }
          frame True {
          }
        }
      }
      frame 3 {
        n337 = case shown="4" w1398 {
          tunnel: [w1493 w1555 w1611 w1672 w1902] -> w1484
          tunnel: [w1494 w1552 w1613 w1652 w1910] -> w1483
          tunnel: [50.0 ("Numeric") 50.0 ("Numeric") 50.0 ("Numeric") w1642 "N2 Age"] -> w1482
          tunnel: [w1494 w1554 w1611 w1652 w1907] -> w1481
          tunnel: w1475 -> [_ _ _ _ _]
          tunnel: w1478 -> [_ _ _ _ _]
          tunnel: w1477 -> [_ _ _ _ _]
          tunnel: w1476 -> [_ _ _ _ _]
          tunnel: [w1494 w1552 w1611 w1652 w1951] -> w1480
          tunnel: w1479 -> [_ _ _ _ _]
          tunnel: w1474 -> [_ _ _ _ w1889]
          tunnel: [_ _ _ _ w2011] -> w1473
          tunnel: w1472 -> [_ _ _ _ w1935]
          tunnel: w1471 -> [_ _ _ _ w1993]
          tunnel: w1470 -> [_ _ _ _ w1992]
          tunnel: w1469 -> [_ _ _ _ _]
          tunnel: w1468 -> [_ _ _ _ _]
          tunnel: w1467 -> [_ _ _ _ _]
          tunnel: w1466 -> [_ _ _ _ _]
          tunnel: w1465 -> [_ _ _ _ _]
          tunnel: w1464 -> [_ _ _ _ w1931]
          tunnel: w1463 -> [_ _ _ _ _]
          tunnel: w1462 -> [_ _ _ _ w2003]
          tunnel: w1461 -> [_ _ _ _ w1934]
          tunnel: [w1494 w1552 w1611 w1652 w1956] -> w1460
          tunnel: w1459 -> [_ _ _ _ w1933]
          tunnel: w1458 -> [_ _ _ _ w1932]
          tunnel: [_ _ _ _ w2004] -> w1457
          tunnel: w1456 -> [_ _ _ _ _]
          tunnel: w1455 -> [_ _ _ _ _]
          tunnel: w1454 -> [_ _ _ _ _]
          tunnel: w1453 -> [_ _ _ _ _]
          tunnel: [w1494 w1552 w1611 w1652 w1901] -> w1452
          tunnel: [w1524 w1552 w1612 w1673 w1909] -> w1451
          tunnel: w1450 -> [_ _ _ _ w1999]
          tunnel: w1449 -> [_ _ _ _ w2000]
          tunnel: w1448 -> [_ _ _ _ _]
          tunnel: [_ _ _ _ w1985] -> w1447
          tunnel: w1446 -> [_ _ _ w1665 w1964]
          tunnel: w1445 -> [_ _ _ _ w1937]
          tunnel: w1444 -> [_ _ _ _ w1936]
          tunnel: w1443 -> [_ _ _ _ w1938]
          tunnel: w1442 -> [w1507 w1557 _ w1674 w1988]
          tunnel: [w1507 w1557 _ w1674 w1982] -> w1441
          tunnel: [w1506 w1556 _ w1675 w1983] -> w1439
          tunnel: w1440 -> [w1506 w1556 _ w1675 w1987]
          tunnel: w1438 -> [_ _ _ _ w1990]
          tunnel: [_ _ _ _ w1989] -> w1437
          tunnel: w1436 -> [_ w1551 _ _ w1962]
          tunnel: w1435 -> [_ _ _ _ _]
          tunnel: w1434 -> [w1520 w1585 w1618 _ _]
          tunnel: w1433 -> [w1500 w1560 _ _ _]
          tunnel: w1432 -> [w1503 _ _ _ _]
          tunnel: w1431 -> [_ _ w1616 _ _]
          tunnel: w1430 -> [w1518 w1567 _ w1639 _]
          tunnel: w1429 -> [_ w1566 _ _ _]
          tunnel: [w1494 w1552 w1611 w1652 w1898] -> w1426
          tunnel: [w1494 w1552 w1611 w1652 w1906] -> w1425
          tunnel: [w1494 w1552 w1611 w1652 w1899] -> w1424
          tunnel: [w1491 w1550 w1609 w1676 w1942] -> w1423
          tunnel: [w1491 w1550 w1609 w1677 w1890] -> w1422
          tunnel: w1421 -> [_ _ _ w1676 w1943]
          tunnel: w1420 -> [_ _ _ w1677 w1891]
          tunnel: [w1485 w1544 w1603 w1626 w1968] -> w1418
          tunnel: [w1485 w1544 w1603 w1626 w1966] -> w1417
          tunnel: [w1489 w1548 w1607 w1658 w1977] -> w1416
          tunnel: w1415 -> [_ _ _ w1671 _]
          tunnel: [w1489 w1548 w1607 w1679 w1977] -> w1414
          tunnel: w1413 -> [_ _ _ w1678 _]
          tunnel: w1412 -> [_ _ _ w1663 _]
          tunnel: [0 ("t") 0 ("t") 0 ("t") w1668 0 ("t")] -> w1411
          tunnel: w1410 -> [_ _ _ w1664 _]
          tunnel: w1409 -> [_ _ _ w1667 _]
          tunnel: w1408 -> [_ _ _ w1666 _]
          tunnel: [w1486 w1545 w1604 w1660 w1970] -> w1407
          tunnel: [w1486 w1545 w1604 w1659 w1970] -> w1406
          tunnel: w1405 -> [_ _ _ w1662 _]
          tunnel: [w1489 w1548 w1607 w1661 w1977] -> w1404
          tunnel: w1403 -> [w1488 w1547 w1606 w1657 w1976]
          tunnel: [w1488 w1547 w1606 w1656 w1976] -> w1402
          tunnel: w1401 -> [_ _ _ w1655 _]
          tunnel: [_ _ _ w1651 _] -> w1400
          tunnel: w1399 -> [_ _ _ w1650 _]
          tunnel: w1397 -> [_ _ _ w1646 _]
          tunnel: w1396 -> [_ _ _ w1645 _]
          tunnel: w1395 -> [_ _ _ w1644 _]
          tunnel: w1394 -> [_ _ _ w1643 _]
          tunnel: w1393 -> [_ _ _ w1642 _]
          tunnel: [0 ("index") 0 ("index") 0 ("index") w1641 0 ("index")] -> w1392
          tunnel: w1391 -> [_ _ _ w1640 _]
          tunnel: [w1486 w1545 w1604 w1636 w1970] -> w1390
          tunnel: [w1486 w1545 w1604 w1635 w1970] -> w1389
          tunnel: w1388 -> [_ _ _ w1634 _]
          tunnel: w1387 -> [_ _ _ w1633 _]
          tunnel: [w1486 w1545 w1604 w1632 w1970] -> w1386
          tunnel: [w1486 w1545 w1604 w1631 w1970] -> w1385
          tunnel: w1384 -> [_ _ _ w1630 _]
          tunnel: w1383 -> [_ _ _ w1629 _]
          tunnel: [w1485 w1544 w1603 w1626 w1947] -> w1381
          tunnel: [w1485 w1544 w1603 w1626 w1946] -> w1380
          tunnel: w1379 -> [_ _ _ _ w1945]
          tunnel: w1378 -> [_ _ _ _ w1944]
          tunnel: w1377 -> [_ _ _ _ w1940]
          tunnel: w1376 -> [_ _ _ _ w1939]
          tunnel: w1375 -> [_ _ _ _ w1927]
          tunnel: w1374 -> [_ _ _ _ w1926]
          tunnel: w1373 -> [_ _ _ _ w1925]
          tunnel: w1372 -> [_ _ _ _ w1924]
          tunnel: w1371 -> [_ _ _ _ w1922]
          tunnel: w1370 -> [_ _ _ _ w1923]
          tunnel: w1369 -> [_ _ _ _ w1921]
          frame 0, Default {
            w1486 = dbl[] [] ("Array Out Main")
            w1489 = i16 0
            w1485 = FALSE
            w1491 = 45.0 ("Numeric")
            w1494 = 0.0 ("Numeric")
            # "Rapidox  Input from Rapidox \nLook at replacing from MEXA 7170 or MEXA 1"
            # "Flow Rate input from Shared\nVariables Index 2"
            # "O2 eq up input from NOx can Array"
            # "Lambda targetinput from Shared\nVariables Index 6"
            # "O2 (O2 t) conc input from Shared\nVariables Index 7"
            # "O2 conc input from Shared\nVariables Index 7"
            # "5Hz CO Loop"
            n338 = Index Array(array=w1518, index #1=0 ("index"), index #2=3 ("index")) -> (element #1=w1495:dbl, element #2=w1501:dbl)
            n339 = Subtract(x=w1503, y=w1495) -> (x-y=w1502:dbl)
            n340 = Multiply(x=w1520, y=50.0) -> (x*y=w1512:dbl)
            n341 = Multiply(x=w1500, y=0.05) -> (x*y=w1513:dbl)
            n342 = Subtract(x=w1500, y=w1501) -> (x-y=w1515:dbl)
            n343 = Multiply(x=w1495, y=0.05) -> (x*y=w1511:dbl)
            n344 = Greater?(x=w1515, y=w1513) -> (0:w1509:bool)
            n345 = Greater?(x=w1502, y=w1511) -> (0:w1508:bool)
            n346 = case shown="False" w1508 {
              tunnel: w1502 -> [_ w1534]
              tunnel: w1512 -> [_ w1535]
              tunnel: [0.0 w1529] -> _
              frame False {
              }
              frame True {
                n347 = Multiply(x=w1535, y=w1534) -> (x*y=w1533:dbl)
                n348 = Divide(x=w1533, y=100.0) -> (x/y=w1531:dbl)
                n349 = Multiply(x=w1531, y=0.9) -> (x*y=w1529:dbl)
              }
            }
            n350 = case shown="False" w1509 {
              tunnel: w1515 -> [_ w1542]
              tunnel: w1512 -> [_ w1543]
              tunnel: [0.0 w1537] -> _
              frame False {
              }
              frame True {
                n351 = Multiply(x=w1543, y=w1542) -> (x*y=w1541:dbl)
                n352 = Divide(x=w1541, y=100.0) -> (x/y=w1539:dbl)
                n353 = Multiply(x=w1539, y=0.9) -> (x*y=w1537:dbl)
              }
            }
            n354 = call-poly <vilib>:"PID.vi"("output range"=cluster{"output high":dbl, "output low":dbl} {"output high"=1.0, "output low"=0.0}, "PID gains"="PID gains CO", "process variable"=w1495, "setpoint"=w1503) -> ("output"=w1504:dbl)  [unwired: 6 in, 1 out]
            n355 = call-poly <vilib>:"PID.vi"("output range"=cluster{"output high":dbl, "output low":dbl} {"output high"=40.0, "output low"=0.0}, "PID gains"="PID gains O2", "process variable"=w1501, "setpoint"=w1500) -> ("output"=w1505:dbl)  [unwired: 6 in, 1 out]
            n356 = call "CO MFR loff.vi"("Flow rate"=w1512, "O2t %"=w1503, "Lambda_t"=w1500) -> ()  [unwired: 8 in, 1 out]
            n357 = Multiply(x=w1505, y="O2 Fact COLO") -> (x*y=w1522:dbl)
            n358 = Multiply(x=w1504, y="CO Fact COLO") -> (x*y=w1526:dbl)
            n359 = Add(x="O2 Base COLO", y=w1522) -> (x+y=w1493:dbl)
            n360 = Add(x="CO Base COLO", y=w1526) -> (x+y=w1524:dbl)
          }
          frame 1 {
            w1545 = dbl[] [] ("Array Out Main")
            w1548 = i16 0
            w1544 = FALSE
            w1550 = 45.0 ("Numeric")
            w1552 = 0.0 ("Numeric")
            # "5Hz HC Loop"
            n361 = Index Array(array=w1567, index #1=0 ("index"), index #2=3 ("index")) -> (element #1=w1571:dbl, element #2=w1559:dbl)
            n362 = Multiply(x=w1585, y=50.0) -> (x*y=w1565:dbl)
            n363 = Subtract(x=w1566, y=w1571) -> (x-y=w1570:dbl)
            n364 = Multiply(x=w1560, y=0.05) -> (x*y=w1574:dbl)
            n365 = Subtract(x=w1560, y=w1559) -> (x-y=w1576:dbl)
            n366 = Multiply(x=w1571, y=0.05) -> (x*y=w1573:dbl)
            n367 = Greater?(x=w1576, y=w1574) -> (0:w1569:bool)
            n368 = Greater?(x=w1570, y=w1573) -> (0:w1568:bool)
            n369 = case shown="False" w1568 {
              tunnel: w1570 -> [_ w1593]
              tunnel: w1565 -> [_ w1594]
              tunnel: [0.0 w1588] -> _
              frame False {
              }
              frame True {
                n370 = Multiply(x=w1594, y=w1593) -> (x*y=w1592:dbl)
                n371 = Divide(x=w1592, y=100.0) -> (x/y=w1590:dbl)
                n372 = Multiply(x=w1590, y=0.9) -> (x*y=w1588:dbl)
              }
            }
            n373 = case shown="True" w1569 {
              tunnel: w1576 -> [_ w1601]
              tunnel: w1565 -> [_ w1602]
              tunnel: [0.0 w1596] -> w1563
              frame False {
              }
              frame True {
                n374 = Multiply(x=w1602, y=w1601) -> (x*y=w1600:dbl)
                n375 = Divide(x=w1600, y=100.0) -> (x/y=w1598:dbl)
                n376 = Multiply(x=w1598, y=0.9) -> (x*y=w1596:dbl)
              }
            }
            n377 = Multiply(x=w1563, y=4.76) -> ()  [unwired: 1 out]
            n378 = call "Air MFR loff.vi"("O2 Measured"=w1559, "O2t %"=w1560, "Flow rate"=w1565) -> ("Air MFR"=w1558:dbl)  [unwired: 8 in]
            n379 = call "HC MFR loff.vi"("Flow rate"=w1565, "O2 Eq Up"=w1551, "O2 Measured"=w1559, "O2t %"=w1560, "Lambda_t"=1.0) -> ("HC MFR"=w1562:dbl)  [unwired: 6 in]
            n380 = Multiply(x=w1558, y="O2 Fact HCLO") -> (x*y=w1583:dbl)
            n381 = Add(x="O2 Base HCLO", y=w1583) -> (x+y=w1555:dbl)
            n382 = Multiply(x=w1562, y="HC Fact HCLO") -> (x*y=w1580:dbl)
            n383 = Add(x="HC Base HCLO", y=w1580) -> (x+y=w1554:dbl)
          }
          frame 2 {
            w1604 = dbl[] [] ("Array Out Main")
            w1607 = i16 0
            w1603 = FALSE
            w1609 = 45.0 ("Numeric")
            w1611 = 0.0 ("Numeric")
            # "5Hz NO Loop"
            n384 = Multiply(x=w1618, y=50.0) -> (x*y=w1617:dbl)
            n385 = call "NOSO2 calc age.vi"("PID"=w1616, "Flow Rate"=w1617) -> ("NO/SO2 MFR"=w1615:dbl)  [unwired: 9 in]
            n386 = Multiply(x=w1615, y="NO Factor NOLO") -> (x*y=w1621:dbl)
            n387 = call "CO calc loff.vi"("NOx MFR"=w1615) -> ("CO MFR"=w1614:dbl)  [unwired: 10 in]
            n388 = Add(x=w1621, y="NO Base NOLO") -> (x+y=w1613:dbl)
            n389 = Multiply(x=w1614, y="CO Factor NOLO") -> (x*y=w1624:dbl)
            n390 = Add(x="CO Base NOLO", y=w1624) -> (x+y=w1612:dbl)
          }
          frame 3 {
            w1626 = FALSE
            w1652 = 0.0 ("Numeric")
            # "OSC Test"
            n391 = Index Array(array=w1639) -> (element #1=w1638:dbl, element #2=w1637:dbl)  [unwired: 2 in]
            n392 = Index Array(array=w1655, index #1=2 ("index"), index #2=0 ("index")) -> (element #1=w1653:dbl, element #2=w1627:dbl)
            n393 = Equal?(x=w1671, y=i16 3) -> (x = y?=w1649:bool)
            n394 = Equal To 0?(x=w1650) -> (x = 0?=w1648:bool)
            n395 = case shown="2" w1671 {
              selector: w1671 -> [w1723 w1758 w1818 w1858]
              tunnel: [w1722 w1757 w1817 w1857] -> w1658
              tunnel: w1678 -> [w1721 w1756 w1816 w1856]
              tunnel: [w1720 w1755 w1815 w1855] -> w1679
              tunnel: [0.0 ("Numeric") 0.0 ("Numeric") 7.0 ("Numeric") 0.0 ("Numeric")] -> w1673
              tunnel: [15.0 ("Numeric") 0.0 ("Numeric") 0.0 ("Numeric") 0.0 ("Numeric")] -> w1672
              tunnel: w1665 -> [w1716 _ _ _]
              tunnel: w1664 -> [w1715 _ _ _]
              tunnel: w1666 -> [w1714 w1749 w1811 w1851]
              tunnel: w1667 -> [w1713 w1751 w1812 w1852]
              tunnel: w1663 -> [w1705 w1743 w1797 w1833]
              tunnel: [w1712 w1751 w1812 w1852] -> w1660
              tunnel: [w1711 w1749 w1811 w1851] -> w1659
              tunnel: w1662 -> [_ _ _ _]
              tunnel: [w1710 w1738 w1810 w1835] -> w1656
              tunnel: w1657 -> [w1710 w1746 w1810 w1831]
              tunnel: w1653 -> [w1696 _ _ _]
              tunnel: w1646 -> [w1706 _ _ w1850]
              tunnel: w1645 -> [w1708 _ _ _]
              tunnel: w1644 -> [_ w1742 w1796 _]
              tunnel: w1643 -> [_ _ w1809 _]
              tunnel: [i16 0 w1741 0 ("index") w1838] -> w1641
              tunnel: w1640 -> [_ w1739 _ w1845]
              tunnel: w1638 -> [w1704 _ w1802 _]
              tunnel: w1637 -> [w1703 _ w1801 _]
              tunnel: w1634 -> [w1702 w1735 w1808 w1849]
              tunnel: w1633 -> [w1701 w1734 w1807 w1848]
              tunnel: [w1700 w1735 w1808 w1849] -> w1636
              tunnel: [w1699 w1734 w1807 w1848] -> w1635
              tunnel: [w1698 w1731 w1806 w1837] -> w1632
              tunnel: [w1697 w1730 w1805 w1836] -> w1631
              tunnel: w1630 -> [w1698 w1731 w1804 w1837]
              tunnel: w1629 -> [w1697 w1730 w1803 w1836]
              tunnel: w1627 -> [_ _ w1794 _]
              frame 0, Default {
                # "Air Injection"
                # "Duration"
                # "Loop"
                n396 = local read "Flow rate g/s"() -> (w1692:dbl)
                n397 = local read "Inlet Temp"() -> (w1694:sgl)
                n398 = call "Array_Builder_Dual.vi"("OSC Number"=w1705, "Cycle Length"=w1706, "Array In 2"=w1714, "Input 2"=w1715, "Array In"=w1713, "Input"=w1716) -> ("Array Out Main 2"=w1711:dbl[], "Array Out Main"=w1712:dbl[])  [unwired: 4 in]
                n399 = call "Array_Builder_Dual.vi"("OSC Number"=w1705, "Cycle Length"=w1706, "Array In 2"=w1701, "Input 2"=w1703, "Array In"=w1702, "Input"=w1704) -> ("Array Out Main 2"=w1699:dbl[], "Array Out Main"=w1700:dbl[])  [unwired: 4 in]
                n400 = call "210pt Mov Avg.vi"("Value in"=w1694) -> ("Value out"=w1693:dbl)  [unwired: 10 in]
                n401 = call "210pt Mov Avg.vi"("Value in"=w1692) -> ("Value out"=w1691:dbl)  [unwired: 10 in]
                n402 = Decrement(x=w1721) -> (x-1=w1690:dbl)
                n403 = call "210pt Mov Avg.vi"("Value in"=w1696) -> ("Value out"=w1695:dbl)  [unwired: 10 in]
                n404 = Less Or Equal?(x=w1690, y=0.0) -> (x <= y?=w1717:bool)
                n405 = Build Array(w1693, w1691, w1695) -> (→"OSCArray":dbl[])
                n406 = case shown="True" w1717 {
                  tunnel: w1723 -> [w1725 _]
                  tunnel: [w1725 i16 1] -> w1722
                  tunnel: w1690 -> [w1724 _]
                  tunnel: [w1724 w1726] -> w1720
                  tunnel: w1708 -> [_ w1726]
                  frame False {
                  }
                  frame True {
                  }
                }
              }
              frame 1 {
                w1737 = 3 ("length")
                w1736 = 0 ("index")
                # "Wait"
                # "Duration"
                # "Loop"
                n407 = local read "OSCArray"() -> (w1752:dbl[])
                n408 = Delete From Array(array=w1735, length=w1737, index=w1736) -> (array with subset deleted=w1733:dbl[])  [unwired: 1 out]
                n409 = Delete From Array(array=w1734, length=w1737, index=w1736) -> (array with subset deleted=w1732:dbl[])  [unwired: 1 out]
                n410 = Equal To 0?(x=w1739) -> (x = 0?=w1740:bool)
                n411 = Multiply(x=w1743, y=13) -> (x*y=w1748:i32)
                n412 = Index Array(array=w1752) -> (element #1=w1745:dbl, element #2=w1747:dbl, element #3=w1744:dbl)  [unwired: 3 in]
                n413 = case shown="True" w1740 {
                  tunnel: w1748 -> [_ w1775]
                  tunnel: w1747 -> [_ w1771]
                  tunnel: w1746 -> [w1761 w1778]
                  tunnel: w1745 -> [_ w1777]
                  tunnel: w1744 -> [_ w1773]
                  tunnel: [w1761 w1776] -> w1738
                  tunnel: [w1760 1 ("index")] -> w1741
                  tunnel: w1739 -> [w1760 _]
                  tunnel: w1733 -> [_ w1772]
                  tunnel: w1732 -> [_ w1762]
                  frame False {
                  }
                  frame True {
                    n414 = Increment(x=w1775) -> (x+1=w1782:i32)
                    n415 = Increment(x=w1782) -> (x+1=w1781:i32)
                    n416 = Increment(x=w1781) -> (x+1=w1780:i32)
                    n417 = Increment(x=w1780) -> (x+1=w1779:i32)
                    n418 = Increment(x=w1779) -> (x+1=w1767:i32)
                    n419 = call "OSC_Calc_Digital.vi"("Flow"=w1771, "Lambda 2 Array"=w1762, "Lambda 1 Array"=w1772, "MFC"=w1773) -> ("OSC MFC"=w1764:dbl, "OSC-Meas Flow"=w1768:dbl, "OSC- Calc Flow"=w1769:dbl, "Calculated Flow"=w1770:dbl, "Time"=w1763:dbl)  [unwired: 3 in]
                    n420 = Increment(x=w1767) -> (x+1=w1766:i32)
                    n421 = Increment(x=w1766) -> (x+1=w1765:i32)
                    n422 = Replace Array Subset(array=w1778, new element #1=w1777, index #1=w1775, new element #2=w1771, index #2=w1782, new element #3=w1770, index #3=w1781, new element #4=w1768, index #4=w1780, new element #5=w1769, index #5=w1779, new element #6=w1773, index #6=w1767, new element #7=w1764, index #7=w1766, new element #8=w1763, index #8=w1765) -> (w1776:dbl[])
                  }
                }
                n423 = Decrement(x=w1756) -> (x-1=w1729:dbl)
                n424 = Less Or Equal?(x=w1729, y=0.0) -> (x <= y?=w1759:bool)
                n425 = case shown="True" w1759 {
                  tunnel: w1758 -> [w1784 _]
                  tunnel: [w1784 i16 2] -> w1757
                  tunnel: w1729 -> [w1783 _]
                  tunnel: [w1783 w1785] -> w1755
                  tunnel: w1742 -> [_ w1785]
                  frame False {
                  }
                  frame True {
                  }
                }
              }
              frame 2 {
                # "CO Injection"
                # "Duration"
                # "Loop"
                n426 = local read "Inlet Temp"() -> (w1790:sgl)
                n427 = local read "Flow rate g/s"() -> (w1789:dbl)
                n428 = Reciprocal(x=w1801) -> (1/x=w1800:dbl)
                n429 = Reciprocal(x=w1802) -> (1/x=w1799:dbl)
                n430 = call "210pt Mov Avg.vi"("Value in"=w1790) -> ("Value out"=w1791:dbl)  [unwired: 10 in]
                n431 = call "Array_Builder_Dual.vi"("OSC Number"=w1797, "Cycle Length"=w1796, "Array In 2"=w1803, "Input 2"=w1800, "Array In"=w1804, "Input"=w1799) -> ("Array Out Main 2"=w1805:dbl[], "Array Out Main"=w1806:dbl[])  [unwired: 4 in]
                n432 = call "210pt Mov Avg.vi"("Value in"=w1789) -> ("Value out"=w1792:dbl)  [unwired: 10 in]
                n433 = Decrement(x=w1816) -> (x-1=w1788:dbl)
                n434 = call "210pt Mov Avg.vi"("Value in"=w1794) -> ("Value out"=w1793:dbl)  [unwired: 10 in]
                n435 = Build Array(w1791, w1792, w1793) -> (w1795:dbl[])
                n436 = Less Or Equal?(x=w1788, y=0.0) -> (x <= y?=w1819:bool)
                n437 = local write "OSCArray"(w1795) -> ()
                n438 = case shown="True" w1819 {
                  tunnel: w1818 -> [w1821 _]
                  tunnel: [w1821 i16 3] -> w1817
                  tunnel: w1788 -> [w1820 _]
                  tunnel: [w1820 w1822] -> w1815
                  tunnel: w1809 -> [_ w1822]
                  frame False {
                  }
                  frame True {
                  }
                }
              }
              frame 3 {
                w1844 = 3 ("length")
                w1843 = 0 ("index")
                # "Wait"
                # "Duration"
                # "Loop"
                n439 = local read "OSCArray"() -> (w1847:dbl[])
                n440 = Multiply(x=w1833, y=13) -> (x*y=w1827:i32)
                n441 = Add(x=w1827, y=2) -> (x+y=w1828:i32)
                n442 = Delete From Array(array=w1837, length=w1844, index=w1843) -> (array with subset deleted=w1842:dbl[])  [unwired: 1 out]
                n443 = Delete From Array(array=w1836, length=w1844, index=w1843) -> (array with subset deleted=w1841:dbl[])  [unwired: 1 out]
                n444 = Add(x=w1827, y=8) -> (x+y=w1832:i32)
                n445 = Index Array(array=w1847) -> (element #2=w1839:dbl, element #3=w1840:dbl)  [unwired: 3 in, 1 out]
                n446 = Index Array(array=w1831, index=w1828) -> (element=w1829:dbl)
                n447 = Equal To 0?(x=w1845) -> (x = 0?=w1846:bool)
                n448 = case shown="True" w1846 {
                  tunnel: w1842 -> [_ w1877]
                  tunnel: w1841 -> [_ w1876]
                  tunnel: w1839 -> [_ w1875]
                  tunnel: w1840 -> [_ w1863]
                  tunnel: [w1861 1 ("index")] -> w1838
                  tunnel: w1845 -> [w1861 _]
                  tunnel: w1831 -> [w1860 w1874]
                  tunnel: [w1860 w1869] -> w1835
                  tunnel: w1832 -> [_ w1868]
                  tunnel: w1829 -> [_ w1862]
                  frame False {
                  }
                  frame True {
                    n449 = Increment(x=w1868) -> (x+1=w1867:i32)
                    n450 = Increment(x=w1867) -> (x+1=w1866:i32)
                    n451 = Increment(x=w1866) -> (x+1=w1865:i32)
                    n452 = Increment(x=w1865) -> (x+1=w1864:i32)
                    n453 = call "OSC_Red_Calc.vi"("Ox Calc Flow"=w1862, "Flow"=w1875, "Lambda 2 Array"=w1876, "Lambda 1 Array"=w1877, "MFC"=w1863) -> ("OSC MFC"=w1870:dbl, "OSC-Meas Flow"=w1873:dbl, "OSC- Calc Flow"=w1872:dbl, "Time"=w1871:dbl)  [unwired: 2 in, 1 out]
                    n454 = Replace Array Subset(array=w1874, new element #1=w1873, index #1=w1868, new element #2=w1872, index #2=w1867, new element #3=w1863, index #3=w1866, new element #4=w1870, index #4=w1865, new element #5=w1871, index #5=w1864) -> (w1869:dbl[])
                  }
                }
                n455 = Decrement(x=w1856) -> (x-1=w1825:dbl)
                n456 = Less Or Equal?(x=w1825, y=0.0) -> (x <= y?=w1859:bool)
                n457 = case shown="True" w1859 {
                  tunnel: w1858 -> [w1880 _]
                  tunnel: [w1880 i16 0] -> w1857
                  tunnel: w1825 -> [w1879 _]
                  tunnel: [w1879 w1881] -> w1855
                  tunnel: w1850 -> [_ w1881]
                  frame False {
                  }
                  frame True {
                  }
                }
              }
            }
            n458 = case shown="True" w1649 {
              tunnel: [w1681 w1685] -> w1668
              tunnel: w1663 -> [w1681 w1684]
              tunnel: [i16 0 ("y") i16 1 ("y")] -> w1651
              tunnel: w1648 -> [_ w1682]
              frame False {
              }
              frame True {
                # "Determines end of last loop and Stops"
                n459 = case shown="True" w1682 {
                  tunnel: [w1686 w1688] -> w1685
                  tunnel: w1684 -> [w1686 w1687]
                  frame False {
                  }
                  frame True {
                    n460 = Increment(x=w1687) -> (x+1=w1688:i32)
                  }
                }
              }
            }
            n461 = Equal?(x=w1668, y=i16 6) -> (x = y?=→"OSC Stop":bool)
            n462 = Increment(x=w1662) -> (x+1=w1661:i16)
          }
          frame 4 {
            w1887 = 0.0
            (unwired) 0.0 ("Numeric")
            w1970 = dbl[] [] ("Array Out Main")
            w1977 = i16 0
            # "O2-2"
            # "CO- 2"
            # "Air 2 Add Addition"
            # "Air 2"
            # "HC 2 Add Addition"
            # "HC 2 Cyc"
            # "O2"
            # "Valve 4"
            # "5Hz Ageing Loop"
            # "NO"
            # "CO"
            # "Air Bal"
            # "Air Addition"
            # "Air 1"
            # "HC Bal"
            # "HC 1 Add Addition"
            # "MFC's\n\nHC\nAir_1\nAir_B\nHC_B\nAir_2"
            # "HC 1 Cyc"
            n463 = local read "Spike Control"() -> (w1893:bool)
            n464 = case shown="True" w1893 {
              tunnel: ["HC Cyc Add Factor" w2019] -> w1892
              frame False {
              }
              frame True {
                n465 = local read "HC Add"() -> (w2019:dbl)
              }
            }
            n466 = case shown="True" "ETAS Control" {
              tunnel: w1964 -> [_ w2041]
              tunnel: [w2040 w2041] -> w1963
              tunnel: w1962 -> [w2040 _]
              frame False {
              }
              frame True {
              }
            }
            n467 = Equal?(x=w2003, y=w1889) -> (x = y?=w2010:bool)
            n468 = Index Array(array=w1935, index=w1889) -> (element=w1994:dbl)
            n469 = Index Array(array=w1993, index=w1889) -> (element=w1997:dbl)
            n470 = Index Array(array=w1992, index=w1889) -> (element=w1996:dbl)
            n471 = Index Array(array=w1934, index=w1889) -> (element=w2008:dbl)
            n472 = Index Array(array=w1933, index=w1889) -> (element=w2006:dbl)
            n473 = Index Array(array=w1932, index=w1889) -> (element=w1980:dbl)
            n474 = Index Array(array=w1931, index=w1889) -> (element=w1930:dbl)
            n475 = Index Array(array=w1937, index=w1889) -> (element=w1948:dbl)
            n476 = Index Array(array=w1936, index=w1889) -> (element=w1955:dbl)
            n477 = Index Array(array=w1926, index=w1889) -> (element=w1928:dbl)
            n478 = Index Array(array=w1925, index=w1889) -> (element=w1911:dbl)
            n479 = Index Array(array=w1924, index=w1889) -> (element=w1912:dbl)
            n480 = Index Array(array=w1923, index=w1889) -> (element=w1913:dbl)
            n481 = Index Array(array=w1922, index=w1889) -> (element=w1914:dbl)
            n482 = Index Array(array=w1921, index=w1889) -> (element=w1915:dbl)
            n483 = Increment(x=w1889) -> (x+1=w2013:i32)
            n484 = Select(t=0, s=w2010, f=w2013) -> (s? t:f=w2011:i32)
            n485 = call "Mov_Avg_JS.vi"("Array In"=w1990, "Cycle Length"=60, "Input"=w1963) -> ("Array Out Main"=w1989:dbl[], "Mean"=w1960:dbl)  [unwired: 7 in]
            "Lambda Avg" <- w1960
            n486 = case shown="True" w1927 {
              tunnel: w1930 -> [w2020 _]
              tunnel: [w2020 w2021] -> w1929
              tunnel: w1928 -> [_ w2021]
              frame False {
              }
              frame True {
              }
            }
            n487 = Multiply(x=w1994, y="CO Factor") -> (x*y=w1909:dbl)
            n488 = Multiply(x=w1997, y="HC Cyc Factor") -> (x*y=w1971:dbl)
            n489 = Multiply(x=w1996, y=w1892) -> (x*y=w1972:dbl)
            n490 = Multiply(x=w2008, y="Air Cyc Factor") -> (x*y=w1974:dbl)
            n491 = Multiply(x=w2006, y="Air Cyc Add Factor") -> (x*y=w1973:dbl)
            n492 = Multiply(x=w1980, y="O2 Factor") -> (x*y=w1899:dbl)
            n493 = Add(x=w1974, y=w1973) -> (x+y=w1902:dbl)
            n494 = Add(x=w1971, y=w1972) -> (x+y=w1907:dbl)
            n495 = Multiply(x=w1911, y="HC 2 Factor") -> (x*y=w1896:dbl)
            n496 = Multiply(x=w1912, y="HC 2 Add Factor") -> (x*y=w1895:dbl)
            n497 = Multiply(x=w1913, y="Air-2 Factor") -> (x*y=w1897:dbl)
            n498 = Multiply(x=w1914, y="Air-2 Add Factor") -> (x*y=w1894:dbl)
            n499 = Add(x=w1902, y=w1894) -> (x+y=w1903:dbl)
            n500 = Multiply(x=w1915, y="O2-2 Factor") -> (x*y=w1898:dbl)
            n501 = Add(x=w1898, y=w1899) -> (x+y=w1900:dbl)
            n502 = Build Array(w1903, w1900) -> (w1904:dbl[])
            n503 = case shown="True" "HC Bal Adaptive Control" {
              tunnel: "HC Bal Factor" -> [w2031 w2039]
              tunnel: w1937 -> [_ w2037]
              tunnel: w1904 -> [_ w2036]
              tunnel: "HC Bal Transient" -> [_ w2035]
              tunnel: [w2032 w2034] -> w1956
              tunnel: w1955 -> [w2033 _]
              frame False {
                n504 = Multiply(x=w2031, y=w2033) -> (x*y=w2032:dbl)
              }
              frame True {
                # "F = Omega"
                n505 = call "HC-Bal_Calc.vi"("Omicron?"=TRUE, "HC Bal Transient"=w2035, "HC Bal Factor"=w2039, "Air_Inj"=w2036, "Air_Bal_Array"=w2037) -> ("HC Bal Inj"=w2034:dbl)  [unwired: 6 in]
              }
            }
            n506 = Add(x=w1897, y=w1894) -> (x+y=w1901:dbl)
            n507 = Add(x=w1896, y=w1895) -> (x+y=w1906:dbl)
            n508 = Add(x=w1907, y=w1895) -> (x+y=w1905:dbl)
            n509 = Index Array(array=w1938, index=w1889) -> (element=w1985:dbl)
            n510 = Index Array(array=w1939, index=w1889) -> (element=w1984:dbl)
            n511 = Index Array(array=w1940, index=w1889) -> (element=w1941:dbl)
            n512 = Index Array(array=w1945, index=w1889) -> (element=w1888:dbl)
            n513 = Index Array(array=w1944, index=w1889) -> (element=w1885:dbl)
            n514 = Multiply(x=w1929, y="NO/CO-2 Factor") -> (x*y=w1910:dbl)
            n515 = Add(x=w1910, y=w1909) -> (x+y=w1908:dbl)
            n516 = Build Array(w1908, w1905) -> (w1952:dbl[])
            n517 = case shown="True" "Air Bal Adaptive Control" {
              tunnel: w1937 -> [_ w2030]
              tunnel: "Air Bal Factor" -> [w2022 w2029]
              tunnel: "Air Bal Transient" -> [_ w2028]
              tunnel: w1952 -> [_ w2026]
              tunnel: [w2024 w2027] -> w1949
              tunnel: w1948 -> [w2023 _]
              frame False {
                n518 = Multiply(x=w2023, y=w2022) -> (x*y=w2024:dbl)
              }
              frame True {
                n519 = call "Air-Bal_Calc.vi"("Omicron?"=TRUE, "Air Bal Transient Factor"=w2028, "Air Bal Factor"=w2029, "Air_Bal_Array"=w2030, "Fuel_Inj"=w2026) -> ("Air Bal"=w2027:dbl)  [unwired: 6 in]
              }
            }
            n520 = case shown="True" "Fan Speed Recipe" {
              tunnel: w1885 -> [_ w2017]
              tunnel: [w2014 w2015] -> w1884
              frame False {
                n521 = local read "Fan Speed V"() -> (w2014:dbl)
              }
              frame True {
                n522 = local read "Fan Speed V"() -> (w2016:dbl)
                n523 = Multiply(x=w2017, y=w2016) -> (x*y=w2015:dbl)
              }
            }
            "Fan Factor Speed" <- w1884
            n524 = case shown="True" "Lambda Control" {
              tunnel: w1999 -> [_ w2061]
              tunnel: w2000 -> [_ w2063]
              tunnel: "Lambda SP 3" -> [_ w2062]
              tunnel: w1960 -> [_ w2060]
              tunnel: w1949 -> [w2056 w2058]
              tunnel: [w2056 w2057] -> w1951
              frame False {
              }
              frame True {
                n525 = call-poly <vilib>:"PID.vi"("output range"=w2063, "PID gains"=w2061, "process variable"=w2060, "setpoint"=w2062) -> ("output"=w2059:dbl)  [unwired: 6 in, 1 out]
                n526 = Add(x=w2058, y=w2059) -> (x+y=w2057:dbl)
              }
            }
            n527 = Not Equal To 0?(x=w1887) -> (x != 0?=w1969:bool)
            n528 = Not Equal To 0?(x=w1887) -> (x != 0?=w1967:bool)
            n529 = case shown="False" "Manual Valve" {
              tunnel: w1988 -> [_ w2055]
              tunnel: w1987 -> [_ w2054]
              tunnel: w1985 -> [w2050 _]
              tunnel: w1984 -> [w2051 _]
              tunnel: [w2051 w2054] -> w1983
              tunnel: [w2050 w2055] -> w1982
              tunnel: w1943 -> [_ w2053]
              tunnel: [w2049 w2053] -> w1942
              tunnel: w1941 -> [w2049 _]
              tunnel: w1891 -> [_ w2052]
              tunnel: [w2048 w2052] -> w1890
              tunnel: w1888 -> [w2048 _]
              frame False {
              }
              frame True {
              }
            }
            n530 = case shown="False" "Dual Evac" {
              tunnel: w1969 -> [w2045 w2047]
              tunnel: [w2045 w2047] -> w1968
              tunnel: w1967 -> [w2042 w2046]
              tunnel: [FALSE w2047] -> w1966
              tunnel: [w2042 w2046] -> w1947
              tunnel: [FALSE w2046] -> w1946
              frame False {
              }
              frame True {
              }
            }
            n531 = Boolean To (0,1)(Boolean=FALSE ("CUToff 1")) -> (0, 1=w2004:i16)
          }
        }
      }
      frame 4 {
        w2066 = dbl[] [] ("Array Out Main")
        w2069 = i16 0
        w2064 = FALSE
        w2073 = 45.0 ("Valve 1 SP")
        w2074 = 0.0 ("Numeric")
      }
      frame 5 {
        w2080 = dbl[] [] ("Array Out Main")
        w2083 = i16 0
        w2078 = FALSE
        w2087 = 45.0 ("Valve 1 SP")
        w2088 = 0.0 ("Numeric")
      }
    }
    n532 = call "Valve_SP.vi"("Valve 1 SP"=w1225) -> ("Output"=w1226:u8[])  [unwired: 10 in]
    n533 = call "Valve_SP.vi"("Valve 1 SP"=w1224) -> ("Output"=w1227:u8[])  [unwired: 10 in]
    n534 = call "Valve_SP.vi"("Valve 1 SP"=w1199) -> ("Output"=w1201:u8[])  [unwired: 10 in]
    n535 = call "Valve_SP.vi"("Valve 1 SP"=w1198) -> ("Output"=w1200:u8[])  [unwired: 10 in]
    n536 = local read "Omicron"() -> (w1091:bool)
    n537 = xnode "Read/Write Control"("FPGA VI Reference In"=w1178, "Evac 1"=w1177, "Evac 2"=w1176, "Evac 3"=w1104, "Evac 4"=w1103) -> ()  [unwired: 1 in, 2 out]
    n538 = Build Array(w1257, w1269, w1298, w1297, w1270, w1296, w1268, w1258, w1196, w1195, w1194) -> (w1282:dbl[])
    n539 = Delete From Array(array=w1105, length=11, index=37) -> (deleted portion=w1130:dbl[])  [unwired: 1 out]
    n540 = Build Array (concatenate)(w1226, w1227, w1201, w1200) -> (w1197:u8[])
    n541 = call "MFR Flow to SP 2-2_RS232.vi"("Omicron"=w1091, "MFC Size"=w1130, "MFC SPs"=w1282) -> ("MFC array"=w1191:u8[], "SV Array"=w1185:bool[])  [unwired: 7 in]
    n542 = shared-variable "RT CompactRIO Target\\Library 1.lvlib\\OSC"(w1111) -> ()  [unwired: 1 in, 1 out]
    n543 = Build Array (concatenate)(w1185, "HC Switch") -> (w1184:bool[])
    n544 = Build Array (concatenate)(w1159, w1282, w1261, w1262, w1192, w1112) -> (w1283:dbl[])
    n545 = shared-variable "RT CompactRIO Target\\Library 1.lvlib\\DATA_2"(w1283) -> ()  [unwired: 1 in, 1 out]
    n546 = xnode "Read/Write Control"("FPGA VI Reference In"=w1178, "MFC Array Out"=w1191, "DO SV Array Out"=w1184, "Valve Array Out"=w1197) -> ()  [unwired: 1 in, 2 out]
    n547 = node-c288() -> ()  [unwired: 1 in, 1 out]
    "Time Step" <- w1290
  }
  n548 = node-c288(w27) -> ()  [unwired: 1 out]
  n549 = node-c288(w43) -> ()  [unwired: 1 out]
  n550 = node-c288(w49) -> ()  [unwired: 1 out]
  n551 = xnode "Close FPGA VI Reference"("FPGA VI Reference In"=w36, "error in"=w35) -> ()  [unwired: 1 out]
